vi "NI845X EEPROM Programmer.vi"() -> ()   [LabVIEW 2025]
doc: "This example shows a more generalized way to use the SPI advanced API to write data. It allows the user to change the following parameters: page size, write delay, the endianness of the address bytes, and the number of bytes in an address.\n\nThe parameters will have the following effects:\n\nTarget Page Size (bytes): This places an additional constraint on the amount of bytes written. The smaller value will be used, and that number of bytes written.\nWrite Delay Between Pages (ms): This will force a mandatory delay after writing bytes to a device.\nData Address Width: This will allow the user to specify the EEPROM Data Address as either 1 or 2 bytes.\nData Address Endianness: This control will change the ordering of the bytes in the EEPROM Data Address, note that this only has an effect if there are 2 bytes in the address.\n\nFor connection information see the NI-845x Hardware and Software manual and the manual for your specific SPI device."
uses:
  Subs/ni845x.llb/NI-845x SPI Close Script Reference.vi
  Subs/ni845x.llb/NI-845x SPI Script Us Delay.vi
  <vilib>/LAVA/UI Tools/Dialog/Dialog/Dialog/Dialog__lava_lib_ui_tools.lvclass
  Subs/ni845x.llb/NI-845x SPI Script Ms Delay.vi
  <resource>/objmgr/NI845x.rc
  <userlib>/_OpenG.lib/md5/md5.llb/MD5 Message Digest (Hexadecimal String)__ogtk.vi
  Subs/ni845x.llb/ni845xControl.ctl
  Subs/ni845x.llb/ni845xSpiScriptControl.ctl
panel:
  in  "SPI Script Reference":T1
  in  "Verbose?":bool
  in  "Config INI Save":bool
  in  "Help":bool
  in  "QUIT":bool
  in  "Main Panel":T2(tab)
  in  "Sub-Panel":T3(tab)
  out "Program Data Array":i32(slide) scale=0.0..32.0
  in  "Path to MD5 Fingerprint":path
  in  "Path to BIN file":path
  in  "Upload BIN File":bool
  in  "EEPROM Program Data":string[][](table)
  out "Data Bytes Written":u8[](array[numeric]) format="%x"
  in  "Write Device":bool
  in  "Save to BIN File":bool
  in  "Read Device":bool
  in  "Read ALL Device":bool
  in  "Address":u16 step=1 format="%04x"
  in  "Bytes to Read":u32=2048 min=2 step=2 format="%04x"
  out "Bin Table":string[][](table)
  out "Hex Table":string[][](table)
  in  "Enable Debug?":bool
  in  "Debug Device":bool
  in  "WRITE Data":u8[](array[numeric]) format="%x"
  out "Read Data":u8[](array[numeric]) format="%x"
  out "Status":string
  out "Binary String_Load":string
  out "MD5_File":string
  out "MD5_Calc":string
  out "Binary String_Save":string
  in  "Invert Data Bits [LSB]":bool
  in  "Invert Data Bits [MSB]":bool
  in  "Endianness (WRITE)":bool=TRUE
  in  "Target Page Size (bytes)":u32=2 min=2 step=2 format="%04x"
  in  "Page Write Delay (ms)":u8=7
  in  "Bit Pattern (WRITE ALL)":T4(ring)=enum."All ONES"
  in  "Erase ALL Device":bool
  in  "Write ALL Device":bool
  in  "EWDS":u8=16 format="%08b"
  in  "EWEN":u8=19 format="%08b"
  in  "WRITE":u8=20 format="%08b"
  in  "READ":u8=24 format="%08b"
  in  "ERAL":u8=18 format="%08b"
  in  "WRAL":u8=17 format="%08b"
  in  "Invert Address":bool
  in  "Invert Opcode":bool=TRUE
  in  "CLK Rate (kHz)":u16=2000
  in  "CS/SS Line (0-6)":u32
  in  "IO Level (V)":i32(ring)=33 items=["3.3V"=33, "2.5V"=25, "1.8V"=18, "1.5V"=15, "1.2V"=12]
  in  "CLK Polarity (CPOL)":i32(ring) items=["0 (Idle Low)", "1 (Idle High)"]
  in  "CLK Phase (CPHS)":i32(ring) items=["0 (First Edge)", "1 (Second Edge)"]
  in  "CS Idle Level":enum16{"Low (Assert High)", "High (Assert Low)"}(ring)
  in  "NI845x Device ID":T5="NI-8452"
  in  "Device Mode":enum16{"SPI", "I2C", "DIO"}(ring)
  in  "EEPROM Device Type":T6(ring)=enum."Microchip 93LC86C [8452]"
  in  "Burst Width":enum16{"8 bits", "16 bits", "32 bits"}(ring)=enum."16 bits" caption="Burst Width\n(NI-8452 Only)"
  in  "Address Width":enum16{"8 bits", "16 bits", "32 bits"}(ring)=enum."16 bits"
  # "EEPROM Programmer\n(NI-USB-845x SPI for 8, 16, 32, 64-bit Devices)"
  # "v2.1"
  # "Note: \n1. NI-8451 is 8-bits only!\n2. NI-8452 is 4-64 bits addressable.\n3. NI-845x SPI/I2C programmer device\nsends MSB first!"
  # "<<-- Opcode + 2 bits Address (MSB)"
  # "<<-- Address: 8 bits (LSB)"
  # "<<-- Data: MSB (8 bits)"
  # "<<-- Data: LSB (8 bits)"
  # "WRITE only"
  # "Big Endian"
  # "Little Endian"
  # "WRITE & READ"
  # "Note: SPI programming mode only! I2C & DIO modes not implemented."
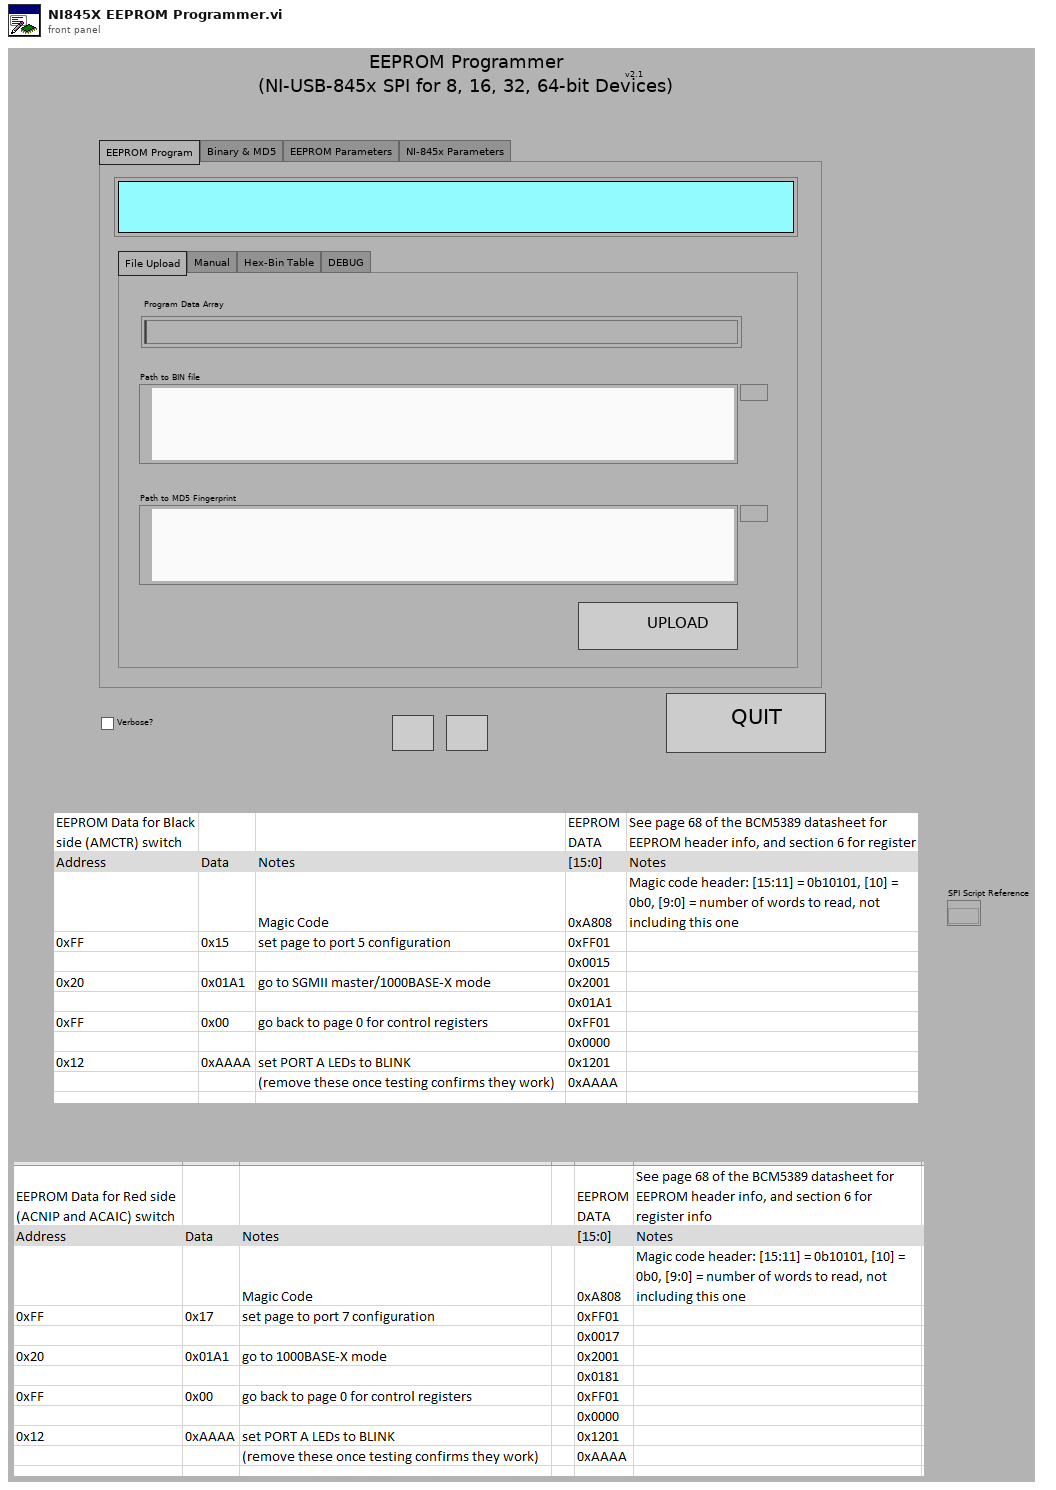
[diagram p1: front panel]
types:
  T1 = typedef "ni845xSpiScriptControl.ctl" = refnum<k20>
  T2 = enum32{"EEPROM Program", "Binary & MD5", "EEPROM Parameters", "NI-845x Parameters"}
  T3 = enum32{"File Upload", "Manual", "Hex-Bin Table", "DEBUG"}
  T4 = enum8{"0xABCD", "0xEEEE", "0xAAAA", "0x5555", "All ONES", "All ZEROES"}
  T5 = typedef "ni845xControl.ctl" = refnum<k21>
  T6 = enum16{"Generic EEPROM", "Microchip LC56BT", "Microchip 93LC86C [8451]", "Microchip 93LC86C [8452]", "ST-M93C86"}
  T7 = enum32{"Invalid", "Standard", "Closed", "Hidden", "Minimized", "Maximized"}
  T8 = enum32{"invalid app kind", "Development System", "Run Time System", "Student Edition", "Embedded LabVIEW", "Evaluation", "Custom"}
  T9 = enum16{"big-endian, network order", "native, host order", "little-endian"}
  T10 = cluster{"INI Path":path, "SPI Script Reference":T1, "NI845x Device ID":T5, "Device Mode":enum16{"SPI", "I2C", "DIO"}, "EEPROM Device Type":enum16{"Generic EEPROM", "Microchip LC56BT", "Microchip 93LC86C [8451]", "Microchip 93LC86C [8452]", "ST-M93C86"}, "Core":cluster{"Current VI Reference":refnum<vi>, "Close Panel on Exit?":bool}, "IO Level (V)":i32, "CS/SS Line (0-6)":u32, "CLK Rate (kHz)":u16, "CLK Polarity (CPOL)":i32, "CLK Phase (CPHS)":i32, " Address Width":enum16{"8 bits", "16 bits", "32 bits"}, "Burst Width":enum16{"8 bits", "16 bits", "32 bits"}, "Address":u16, "Bytes to Read":u32, "Target Page Size (bytes)":u32, "Page Write Delay (ms)":u8, "Array of Write Cluster Information":cluster{"EEPROM Address":u16, "Length":u32, "Data Index":u32}[], "CS Idle Level":enum16{"Low (Assert High)", "High (Assert Low)"}, "script read index":u32, "Bit Pattern (WRITE ALL)":enum8{"0xABCD", "0xEEEE", "0xAAAA", "0x5555", "All ONES", "All ZEROES"}, "READ":u8, "WRITE":u8, "EWEN":u8, "EWDS":u8, "WRAL":u8, "ERAL":u8, "Hex Table":string[][], "Bin Table ":string[][], "EEPROM Program Data ":string[][], "EEPROM Binary File Array":string[][], "Read Data":u8[], "Data Bytes Written":u8[], "WRITE Data":u8[], "Endianness (WRITE)":bool, "Verbose?":bool, "Enable Debug?":bool, "Read ALL":bool, "Invert Data Bits [MSB]":bool, "Invert Data Bits [LSB]":bool, "Invert Opcode":bool, "Invert Address":bool}
  T11 = cluster{"Current VI Reference":refnum<vi>, "Close Panel on Exit?":bool}
  T12 = cluster{"EEPROM Address":u16, "Length":u32, "Data Index":u32}[]
  T13 = typedef "imagedata.ctl" = cluster{"image type":i32, "image depth":i32, "image":u8[], "mask":u8[], "colors":u32[], "Rectangle":cluster{"left":i16, "top":i16, "right":i16, "bottom":i16}}
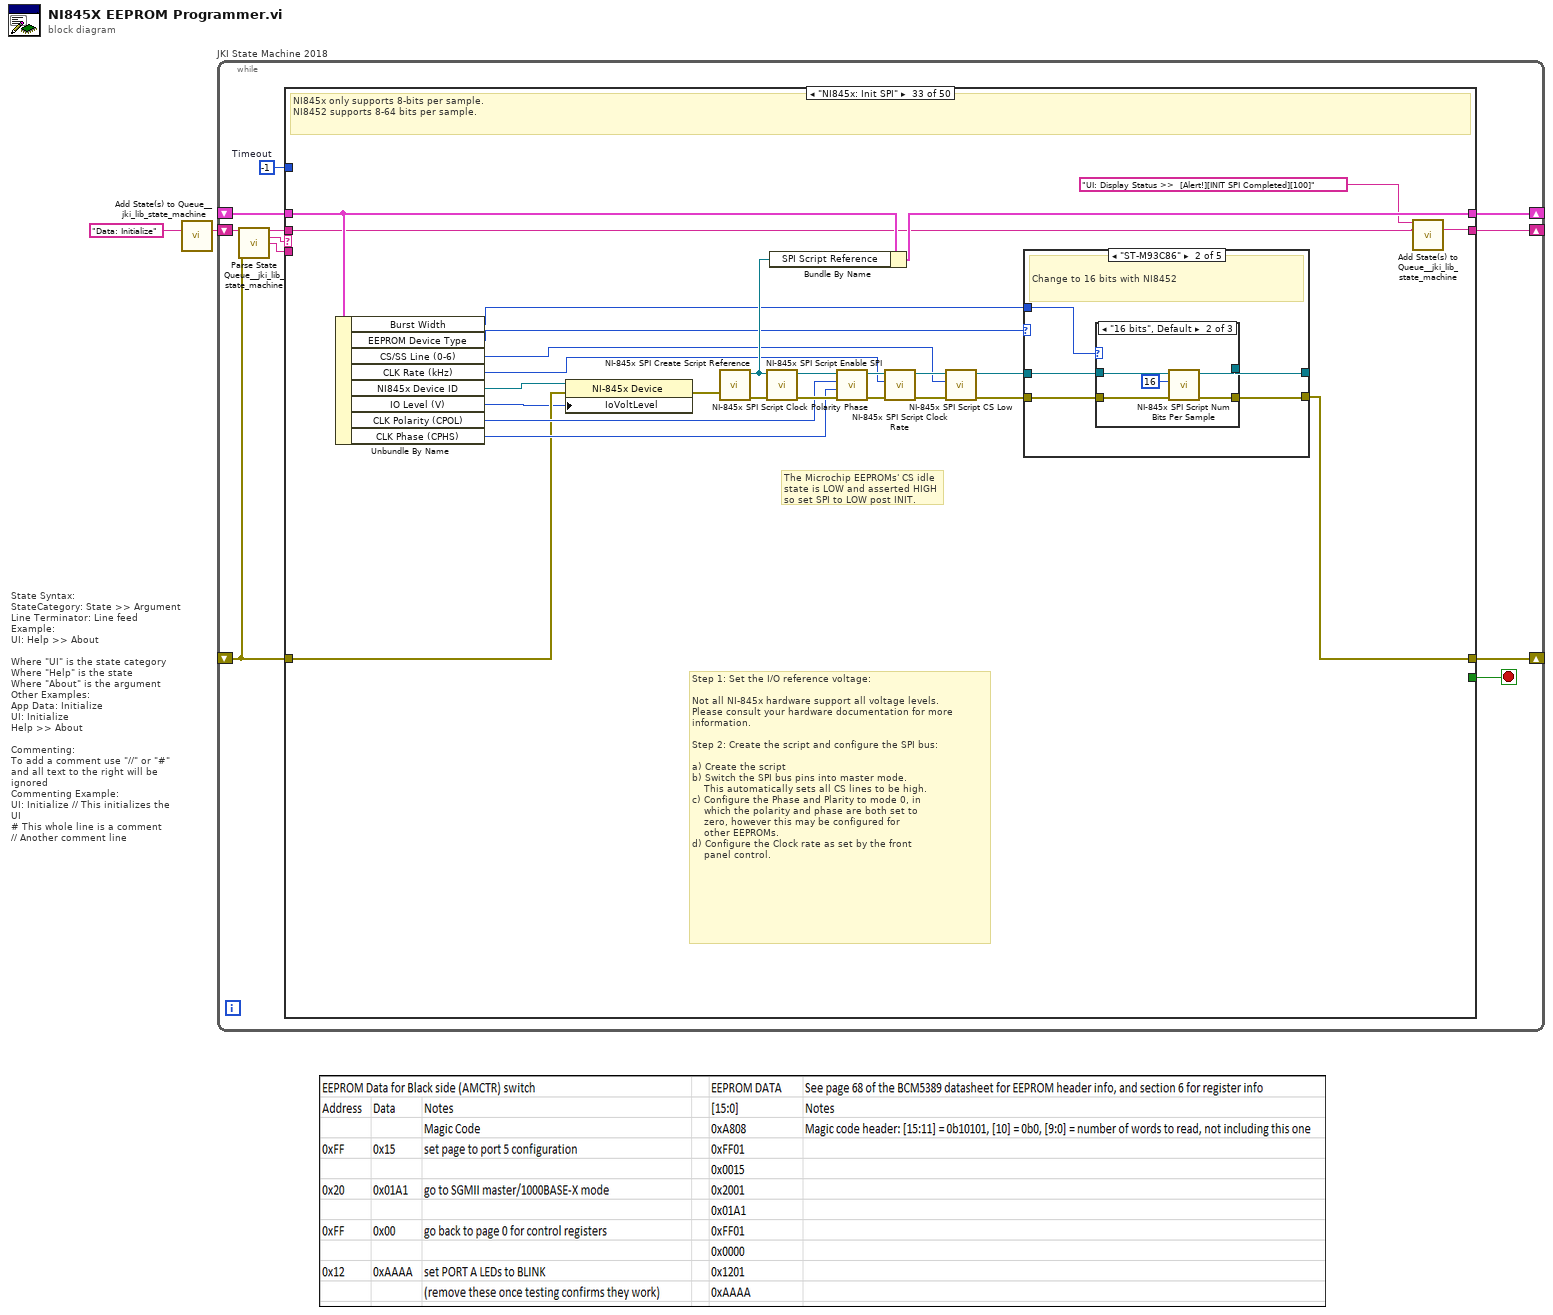
[diagram p0: block diagram]
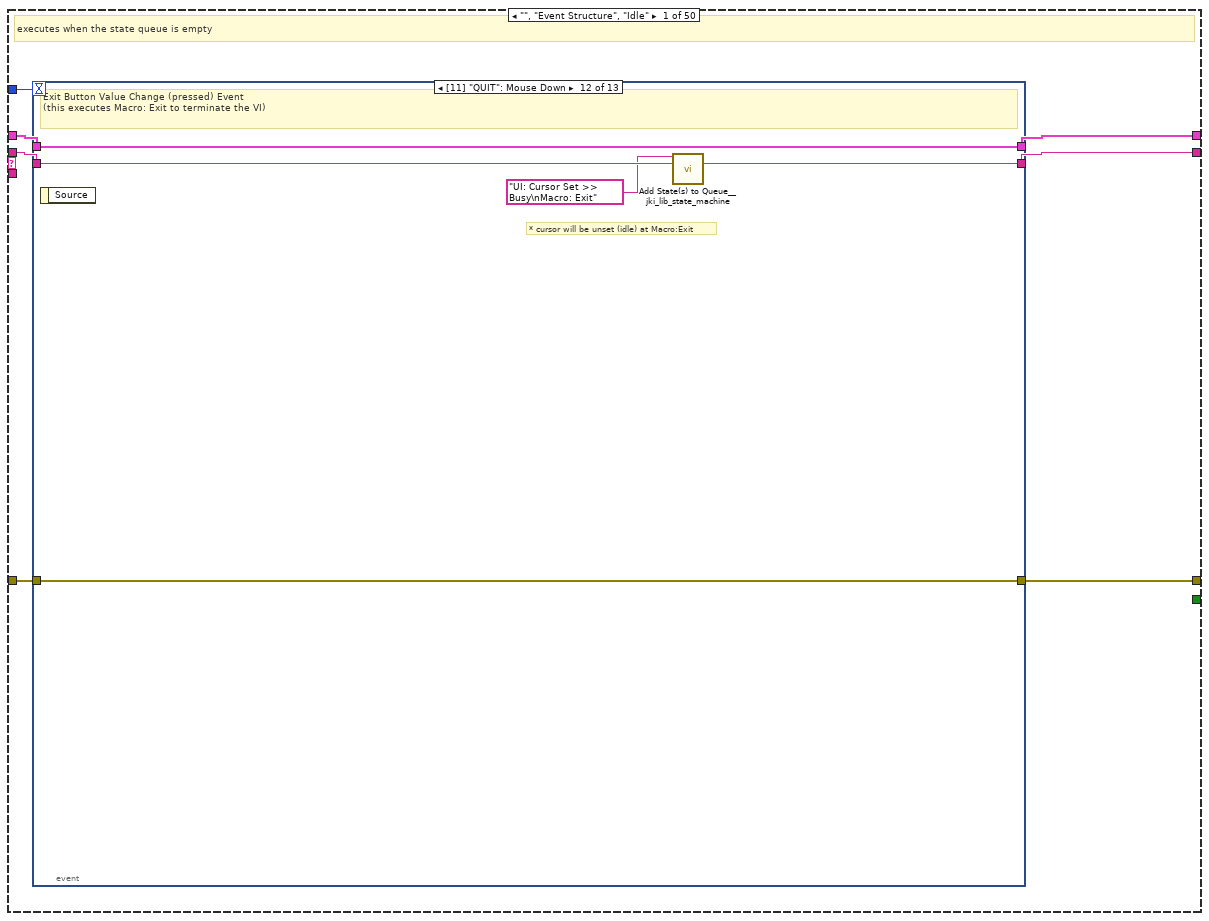
[diagram p2: hidden frame]
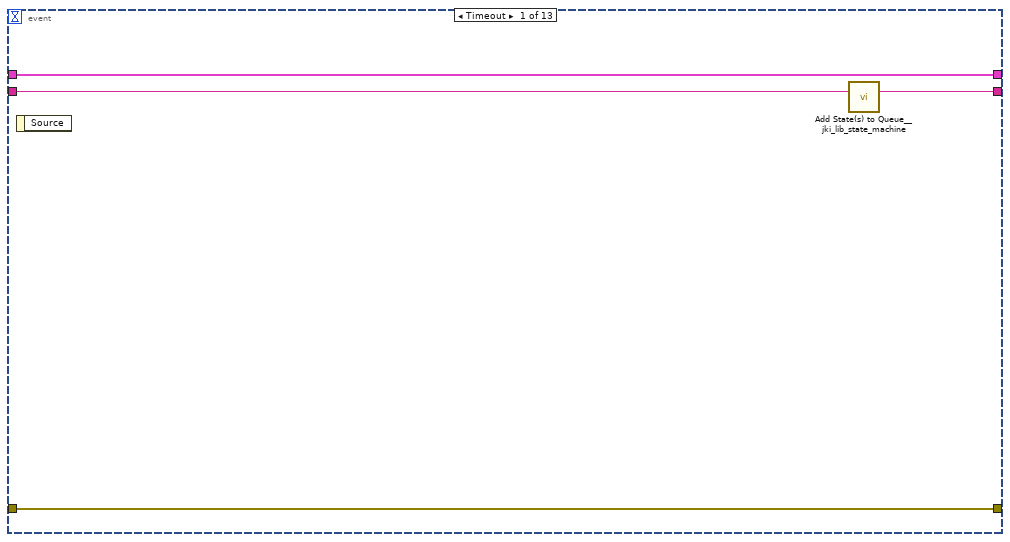
[diagram p3: hidden frame]
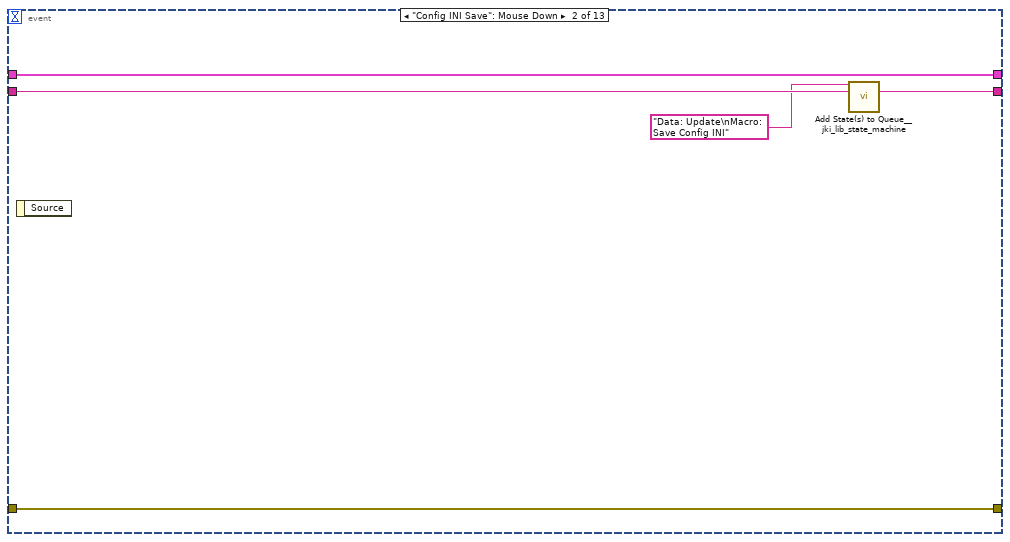
[diagram p4: hidden frame]
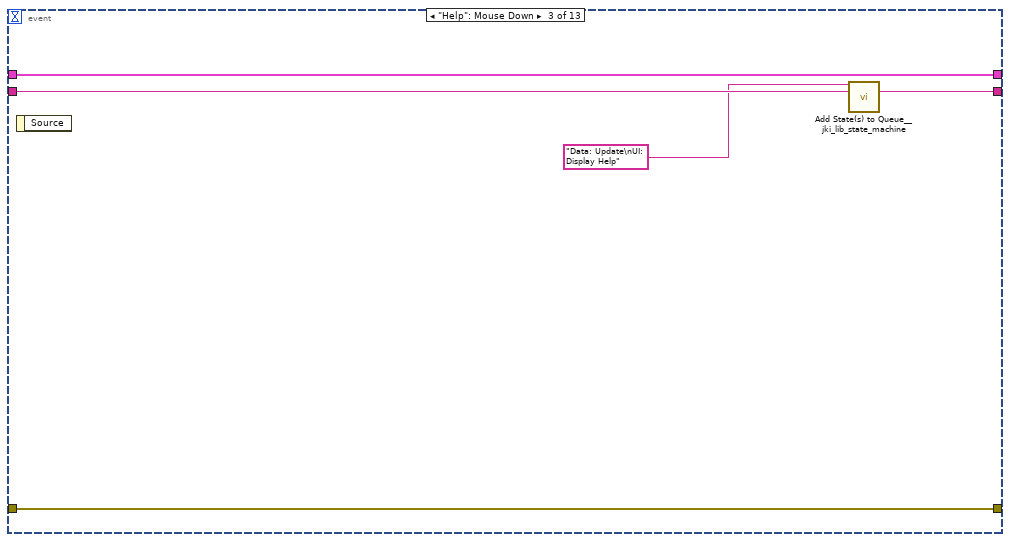
[diagram p5: hidden frame]
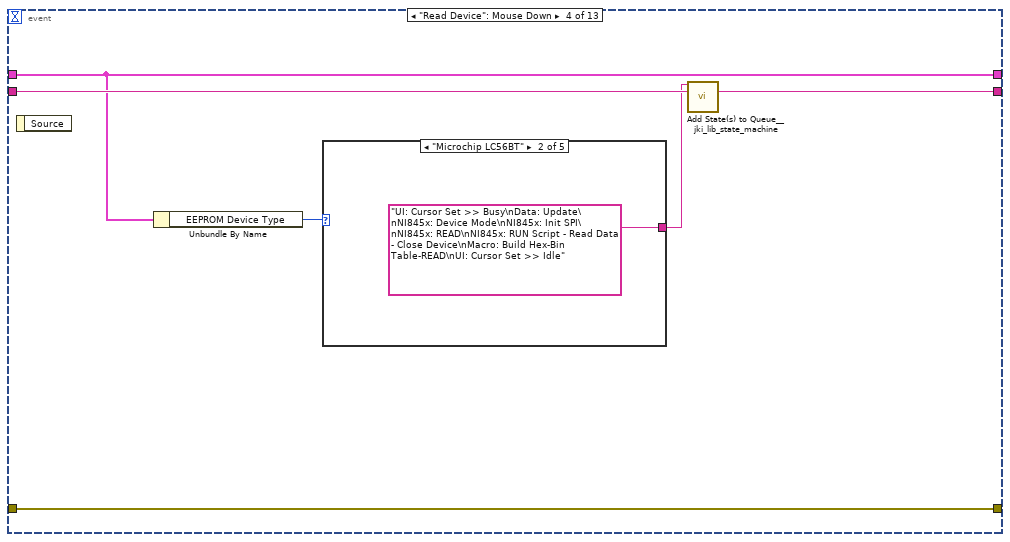
[diagram p6: hidden frame]
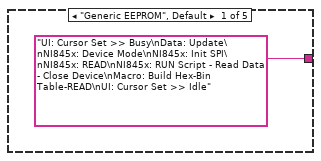
[diagram p7: hidden frame]
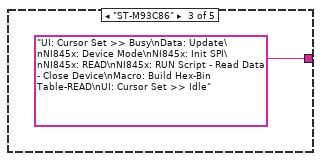
[diagram p8: hidden frame]
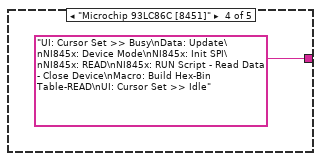
[diagram p9: hidden frame]
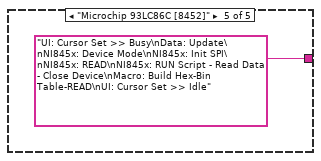
[diagram p10: hidden frame]
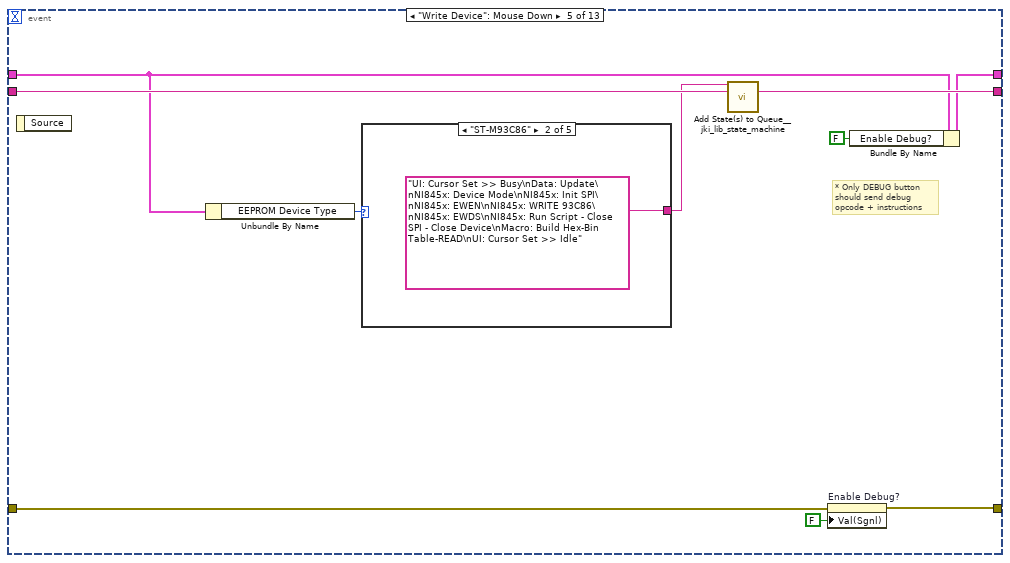
[diagram p11: hidden frame]
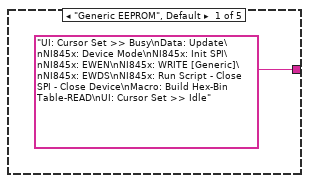
[diagram p12: hidden frame]
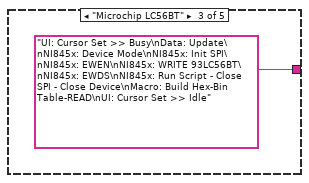
[diagram p13: hidden frame]
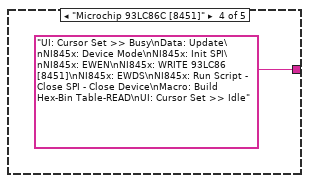
[diagram p14: hidden frame]
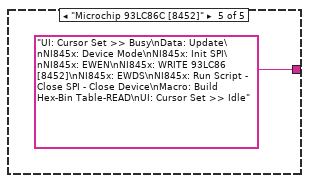
[diagram p15: hidden frame]
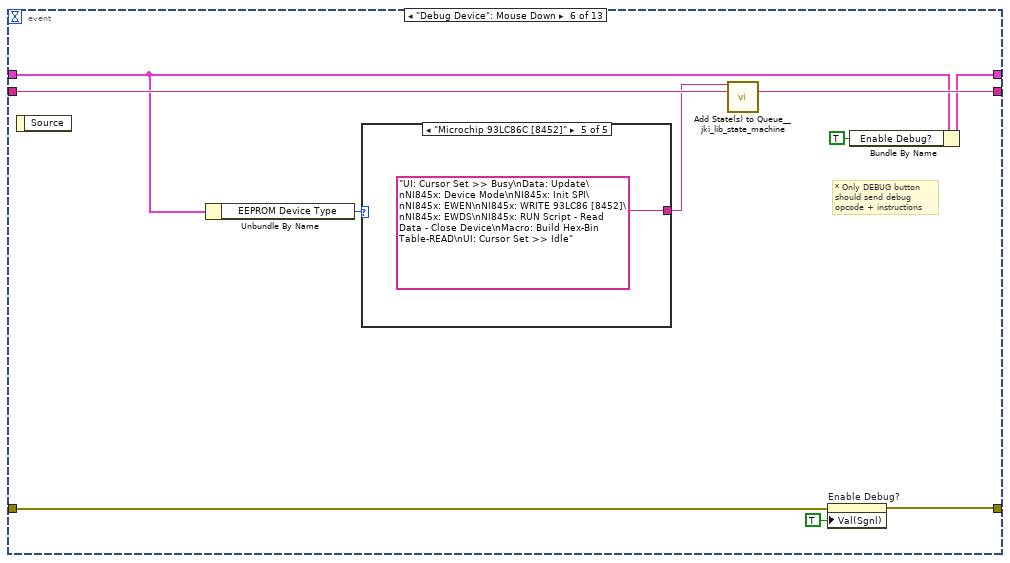
[diagram p16: hidden frame]
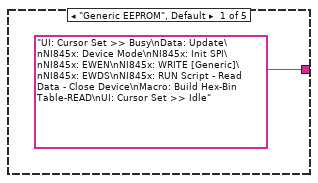
[diagram p17: hidden frame]
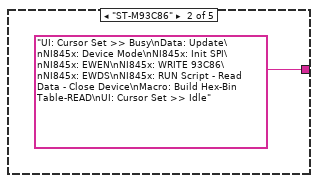
[diagram p18: hidden frame]
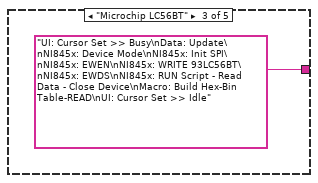
[diagram p19: hidden frame]
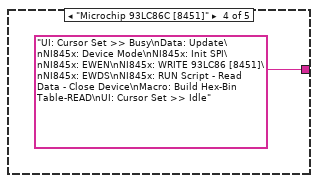
[diagram p20: hidden frame]
diagram:
  # "State Syntax:\nStateCategory: State >> Argument\nLine Terminator: Line feed\nExample:\nUI: Help >> About\n\nWhere \"UI\" is the state category\nWhere \"Help\" is the state\nWhere \"About\" is the argument\nOther Examples:\nApp Data: Initialize\nUI: Initialize\nHelp >> About\n\nCommenting:\nTo add a comment use \"//\" or \"#\" and all text to the right will be ignored\nCommenting Example:\nUI: Initialize // This initializes the UI\n# This whole line is a comment\n// Another comment line"
  n1 = call <vilib>:"Add State(s) to Queue__jki_lib_state_machine.vi"("State(s) in (\"\")"="Data: Initialize") -> ("States Out"=w2:string)  [unwired: 14 in]
  n2 = while "JKI State Machine 2018" {
    shift-right: [w6] -> _
    shift-left: _ -> [w5]
    shift-right: [w9] -> _
    shift-left: _ -> [w3]
    shift-right: [w8] -> _
    shift-left: w2 -> [w10]
    stop <- w7 stop-if-true
    w4 = -1  # Timeout
    n3 = call <vilib>:"Parse State Queue__jki_lib_state_machine.vi"("State Queue"=w10, "Error In (no error)"=w3) -> ("Remaining States"=w12:string, "Current State"=w13:string, "Arguments"=w11:string)  [unwired: 11 in]
    n4 = case shown="\"NI845x: Init SPI\"" w13 {
      selector: w13 -> [_ _ w144 _ _ _ _ _ _ _ _ _ _ _ _ _ _ _ _ _ _ _ _ _ _ _ _ _ _ _ _ _ _ _ _ _ _ _ _ _ _ _ _ _ _ _ _ _ _ _]
      tunnel: w12 -> [w20 w143 w148 w166 w172 w176 w179 w236 w266 w271 w274 w277 w282 w292 w366 w378 w398 w434 w456 w466 w480 w531 w587 w622 w676 w690 w702 w705 w708 w711 w714 w716 w726 w820 w850 w925 w1015 w1103 w1201 w1239 w1348 w1489 w1611 w1653 w1723 w1737 _ w1843 w1860 w1944]
      tunnel: w11 -> [_ _ _ _ _ _ _ _ _ _ _ _ w278 w287 _ w375 w395 _ _ _ _ _ _ _ _ _ _ _ _ _ _ _ _ _ _ _ _ _ _ _ _ _ _ _ _ _ _ _ _ _]
      tunnel: w5 -> [w18 w140 w146 w163 w169 w175 w177 _ w247 w267 w272 w276 w281 w289 w365 w373 w393 w432 w454 w463 w477 w528 w584 w639 w675 w684 w693 w703 w706 w709 w712 w718 w742 w812 w848 w914 w1004 w1093 w1195 w1234 w1343 w1485 w1607 w1646 w1716 w1730 w1766 w1840 w1856 w1941]
      tunnel: [w17 w141 w150 w164 errorcluster {"status"=FALSE, "code"=0, "source"=""} ("error out") w174 w178 w202 w265 w268 w273 w275 w279 w290 w364 w377 w397 w433 w441 w464 w478 w529 w589 w623 w668 w687 w696 w704 w707 w710 w713 w719 w735 w802 w840 w917 w1007 w1095 w1175 w1215 w1319 w1455 w1588 w1648 w1718 w1732 w1768 w1841 w1854 w1934] -> w9
      tunnel: w3 -> [w16 w141 w149 w164 w168 w174 w178 w185 w265 w269 w273 w275 w280 w291 w362 w376 w396 w433 w447 w464 w478 w529 w589 w640 w665 w688 w697 w704 w707 w710 w713 w719 w730 w813 w846 w923 w1013 w1101 w1190 w1230 w1336 w1474 w1587 w1649 w1719 w1733 w1754 w1841 w1855 w1942]
      tunnel: [w19 w142 w147 w166 w171 w176 w179 w235 w266 w271 w274 w277 w282 w292 w366 w378 w398 w434 w455 w465 w479 w530 w586 w621 w676 w689 w701 w705 w708 w711 w714 w720 w725 w819 w849 w924 w1014 w1102 w1200 w1238 w1347 w1488 w1610 w1652 w1722 w1736 w1772 w1842 w1859 w1943] -> w8
      tunnel: [_ _ _ _ _ TRUE _ _ _ _ _ _ _ _ _ _ _ _ _ _ _ _ _ _ _ _ _ _ _ _ _ _ _ _ _ _ _ _ _ _ _ _ _ _ _ _ _ _ _ _] -> w7
      tunnel: [w15 w140 w146 w165 w169 w175 w177 w209 w264 w267 w272 w276 w281 w289 w365 w373 w393 w432 w454 w463 w476 w527 w588 w638 w675 w684 w693 w703 w706 w709 w712 w718 w734 w812 w847 w921 w1011 w1099 w1195 w1232 w1341 w1478 w1597 w1638 w1712 w1726 w1771 w1840 w1850 w1937] -> w6
      tunnel: w4 -> [w14 _ _ _ _ _ _ _ _ _ _ _ _ _ _ _ _ _ _ _ _ _ _ _ _ _ _ _ _ _ _ _ _ _ _ _ _ _ _ _ _ _ _ _ _ _ _ _ _ _]
      frame "", "Event Structure", "Idle" {
        # "executes when the state queue is empty"
        n5 = event shown="[11] \"QUIT\": Mouse Down" {
          selector: _ -> [_ _ _ _ _ _ _ _ _ _ _ _ _]
          dyn-events: _ -> [_ _ _ _ _ _ _ _ _ _ _ _ _]
          timeout: w14 -> [_ _ _ _ _ _ _ _ _ _ _ _ _]
          tunnel: w20 -> [w24 w29 w34 w39 w55 w70 w80 w91 w102 w113 w127 w133 w139]
          tunnel: [w23 w28 w33 w38 w54 w69 w79 w90 w101 w112 w126 w132 w138] -> w19
          tunnel: w18 -> [w21 w26 w31 w36 w52 w67 w77 w88 w99 w110 w124 w130 w136]
          tunnel: [w22 w27 w32 w40 w47 w62 w81 w92 w103 w114 w120 w131 w137] -> w17
          tunnel: w16 -> [w22 w27 w32 w40 w48 w63 w81 w92 w103 w114 w120 w131 w137]
          tunnel: [w21 w26 w31 w36 w50 w65 w77 w88 w99 w110 w122 w130 w136] -> w15
          event Timeout {
            n6 = event-data() -> ()  [unwired: 1 in, 1 out]
            n7 = call <vilib>:"Add State(s) to Queue__jki_lib_state_machine.vi"("State(s) in (\"\")"=w24) -> ("States Out"=w23:string)  [unwired: 14 in]
          }
          event "Config INI Save": Mouse Down {
            n8 = event-data() -> ()  [unwired: 1 in, 1 out]
            n9 = call <vilib>:"Add State(s) to Queue__jki_lib_state_machine.vi"("State(s) in Front (\"\")"="Data: Update\nMacro: Save Config INI" ("State(s) in Front (\"\")"), "State(s) in (\"\")"=w29) -> ("States Out"=w28:string)  [unwired: 13 in]
          }
          event "Help": Mouse Down {
            n10 = event-data() -> ()  [unwired: 1 in, 1 out]
            n11 = call <vilib>:"Add State(s) to Queue__jki_lib_state_machine.vi"("State(s) in Front (\"\")"="Data: Update\nUI: Display Help" ("State(s) in Front (\"\")"), "State(s) in (\"\")"=w34) -> ("States Out"=w33:string)  [unwired: 13 in]
          }
          event "Read Device": Mouse Down {
            n12 = event-data() -> ()  [unwired: 1 in, 1 out]
            n13 = Unbundle By Name(w36) -> ("EEPROM Device Type"=w35:T6)
            n14 = case shown="\"Microchip LC56BT\"" w35 {
              tunnel: ["UI: Cursor Set >> Busy\nData: Update\nNI845x: Device Mode\nNI845x: Init SPI\nNI845x: READ\nNI845x: RUN Script - Read Data - Close Device\nMacro: Build Hex-Bin Table-READ\nUI: Cursor Set >> Idle" ("State(s) in Front (\"\")") "UI: Cursor Set >> Busy\nData: Update\nNI845x: Device Mode\nNI845x: Init SPI\nNI845x: READ\nNI845x: RUN Script - Read Data - Close Device\nMacro: Build Hex-Bin Table-READ\nUI: Cursor Set >> Idle" ("State(s) in Front (\"\")") "UI: Cursor Set >> Busy\nData: Update\nNI845x: Device Mode\nNI845x: Init SPI\nNI845x: READ\nNI845x: RUN Script - Read Data - Close Device\nMacro: Build Hex-Bin Table-READ\nUI: Cursor Set >> Idle" ("State(s) in Front (\"\")") "UI: Cursor Set >> Busy\nData: Update\nNI845x: Device Mode\nNI845x: Init SPI\nNI845x: READ\nNI845x: RUN Script - Read Data - Close Device\nMacro: Build Hex-Bin Table-READ\nUI: Cursor Set >> Idle" ("State(s) in Front (\"\")") "UI: Cursor Set >> Busy\nData: Update\nNI845x: Device Mode\nNI845x: Init SPI\nNI845x: READ\nNI845x: RUN Script - Read Data - Close Device\nMacro: Build Hex-Bin Table-READ\nUI: Cursor Set >> Idle" ("State(s) in Front (\"\")")] -> w37
              frame "Generic EEPROM", Default {
              }
              frame "Microchip LC56BT" {
              }
              frame "ST-M93C86" {
              }
              frame "Microchip 93LC86C [8451]" {
              }
              frame "Microchip 93LC86C [8452]" {
              }
            }
            n15 = call <vilib>:"Add State(s) to Queue__jki_lib_state_machine.vi"("State(s) in Front (\"\")"=w37, "State(s) in (\"\")"=w39) -> ("States Out"=w38:string)  [unwired: 13 in]
          }
          event "Write Device": Mouse Down {
            # "* Only DEBUG button\nshould send debug\nopcode + instructions"
            n16 = event-data() -> ()  [unwired: 1 in, 1 out]
            n17 = Unbundle By Name(w52) -> ("EEPROM Device Type"=w51:T6)
            n18 = case shown="\"ST-M93C86\"" w51 {
              tunnel: ["UI: Cursor Set >> Busy\nData: Update\nNI845x: Device Mode\nNI845x: Init SPI\nNI845x: EWEN\nNI845x: WRITE [Generic]\nNI845x: EWDS\nNI845x: Run Script - Close SPI - Close Device\nMacro: Build Hex-Bin Table-READ\nUI: Cursor Set >> Idle" ("State(s) in Front (\"\")") "UI: Cursor Set >> Busy\nData: Update\nNI845x: Device Mode\nNI845x: Init SPI\nNI845x: EWEN\nNI845x: WRITE 93C86\nNI845x: EWDS\nNI845x: Run Script - Close SPI - Close Device\nMacro: Build Hex-Bin Table-READ\nUI: Cursor Set >> Idle" ("State(s) in Front (\"\")") "UI: Cursor Set >> Busy\nData: Update\nNI845x: Device Mode\nNI845x: Init SPI\nNI845x: EWEN\nNI845x: WRITE 93LC56BT\nNI845x: EWDS\nNI845x: Run Script - Close SPI - Close Device\nMacro: Build Hex-Bin Table-READ\nUI: Cursor Set >> Idle" ("State(s) in Front (\"\")") "UI: Cursor Set >> Busy\nData: Update\nNI845x: Device Mode\nNI845x: Init SPI\nNI845x: EWEN\nNI845x: WRITE 93LC86 [8451]\nNI845x: EWDS\nNI845x: Run Script - Close SPI - Close Device\nMacro: Build Hex-Bin Table-READ\nUI: Cursor Set >> Idle" ("State(s) in Front (\"\")") "UI: Cursor Set >> Busy\nData: Update\nNI845x: Device Mode\nNI845x: Init SPI\nNI845x: EWEN\nNI845x: WRITE 93LC86 [8452]\nNI845x: EWDS\nNI845x: Run Script - Close SPI - Close Device\nMacro: Build Hex-Bin Table-READ\nUI: Cursor Set >> Idle" ("State(s) in Front (\"\")")] -> w53
              frame "Generic EEPROM", Default {
              }
              frame "ST-M93C86" {
              }
              frame "Microchip LC56BT" {
              }
              frame "Microchip 93LC86C [8451]" {
              }
              frame "Microchip 93LC86C [8452]" {
              }
            }
            n19 = call <vilib>:"Add State(s) to Queue__jki_lib_state_machine.vi"("State(s) in Front (\"\")"=w53, "State(s) in (\"\")"=w55) -> ("States Out"=w54:string)  [unwired: 13 in]
            n20 = property on="Enable Debug?" class="Bool (strict)"(error in=w48, "Val(Sgnl)"=FALSE ("Value (Signaling)")) -> (error out=w47:errorcluster)  [unwired: 1 in, 1 out]
            n21 = Bundle By Name(cluster=w52, "Enable Debug?"=FALSE) -> (w50:T10)
          }
          event "Debug Device": Mouse Down {
            # "* Only DEBUG button\nshould send debug\nopcode + instructions"
            n22 = event-data() -> ()  [unwired: 1 in, 1 out]
            n23 = Unbundle By Name(w67) -> ("EEPROM Device Type"=w66:T6)
            n24 = case shown="\"Microchip 93LC86C [8452]\"" w66 {
              tunnel: ["UI: Cursor Set >> Busy\nData: Update\nNI845x: Device Mode\nNI845x: Init SPI\nNI845x: EWEN\nNI845x: WRITE [Generic]\nNI845x: EWDS\nNI845x: RUN Script - Read Data - Close Device\nMacro: Build Hex-Bin Table-READ\nUI: Cursor Set >> Idle" ("State(s) in Front (\"\")") "UI: Cursor Set >> Busy\nData: Update\nNI845x: Device Mode\nNI845x: Init SPI\nNI845x: EWEN\nNI845x: WRITE 93C86\nNI845x: EWDS\nNI845x: RUN Script - Read Data - Close Device\nMacro: Build Hex-Bin Table-READ\nUI: Cursor Set >> Idle" ("State(s) in Front (\"\")") "UI: Cursor Set >> Busy\nData: Update\nNI845x: Device Mode\nNI845x: Init SPI\nNI845x: EWEN\nNI845x: WRITE 93LC56BT\nNI845x: EWDS\nNI845x: RUN Script - Read Data - Close Device\nMacro: Build Hex-Bin Table-READ\nUI: Cursor Set >> Idle" ("State(s) in Front (\"\")") "UI: Cursor Set >> Busy\nData: Update\nNI845x: Device Mode\nNI845x: Init SPI\nNI845x: EWEN\nNI845x: WRITE 93LC86 [8451]\nNI845x: EWDS\nNI845x: RUN Script - Read Data - Close Device\nMacro: Build Hex-Bin Table-READ\nUI: Cursor Set >> Idle" ("State(s) in Front (\"\")") "UI: Cursor Set >> Busy\nData: Update\nNI845x: Device Mode\nNI845x: Init SPI\nNI845x: EWEN\nNI845x: WRITE 93LC86 [8452]\nNI845x: EWDS\nNI845x: RUN Script - Read Data - Close Device\nMacro: Build Hex-Bin Table-READ\nUI: Cursor Set >> Idle" ("State(s) in Front (\"\")")] -> w68
              frame "Generic EEPROM", Default {
              }
              frame "ST-M93C86" {
              }
              frame "Microchip LC56BT" {
              }
              frame "Microchip 93LC86C [8451]" {
              }
              frame "Microchip 93LC86C [8452]" {
              }
            }
            n25 = call <vilib>:"Add State(s) to Queue__jki_lib_state_machine.vi"("State(s) in Front (\"\")"=w68, "State(s) in (\"\")"=w70) -> ("States Out"=w69:string)  [unwired: 13 in]
            n26 = property on="Enable Debug?" class="Bool (strict)"(error in=w63, "Val(Sgnl)"=TRUE ("Value (Signaling)")) -> (error out=w62:errorcluster)  [unwired: 1 in, 1 out]
            n27 = Bundle By Name(cluster=w67, "Enable Debug?"=TRUE) -> (w65:T10)
          }
          event "Read ALL Device": Mouse Down {
            n28 = event-data() -> ()  [unwired: 1 in, 1 out]
            n29 = Unbundle By Name(w77) -> ("EEPROM Device Type"=w76:T6)
            n30 = case shown="\"Generic EEPROM\", Default" w76 {
              tunnel: ["UI: Cursor Set >> Busy\nData: Update\nNI845x: Device Mode\nNI845x: Init SPI\nNI845x: READ ALL\nNI845x: RUN Script - Read Data - Close Device\nMacro: Build Hex-Bin Table-READ-ALL\nUI: Cursor Set >> Idle" ("State(s) in Front (\"\")") "UI: Cursor Set >> Busy\nData: Update\nNI845x: Device Mode\nNI845x: Init SPI\nNI845x: READ ALL\nNI845x: RUN Script - Read Data - Close Device\nMacro: Build Hex-Bin Table-READ-ALL\nUI: Cursor Set >> Idle" ("State(s) in Front (\"\")") "UI: Cursor Set >> Busy\nData: Update\nNI845x: Device Mode\nNI845x: Init SPI\nNI845x: READ ALL\nNI845x: RUN Script - Read Data - Close Device\nMacro: Build Hex-Bin Table-READ-ALL\nUI: Cursor Set >> Idle" ("State(s) in Front (\"\")") "UI: Cursor Set >> Busy\nData: Update\nNI845x: Device Mode\nNI845x: Init SPI\nNI845x: READ ALL\nNI845x: RUN Script - Read Data - Close Device\nMacro: Build Hex-Bin Table-READ-ALL\nUI: Cursor Set >> Idle" ("State(s) in Front (\"\")") "UI: Cursor Set >> Busy\nData: Update\nNI845x: Device Mode\nNI845x: Init SPI\nNI845x: READ ALL\nNI845x: RUN Script - Read Data - Close Device\nMacro: Build Hex-Bin Table-READ-ALL\nUI: Cursor Set >> Idle" ("State(s) in Front (\"\")")] -> w78
              frame "Microchip LC56BT" {
              }
              frame "ST-M93C86" {
              }
              frame "Microchip 93LC86C [8452]" {
              }
              frame "Microchip 93LC86C [8451]" {
              }
              frame "Generic EEPROM", Default {
              }
            }
            n31 = call <vilib>:"Add State(s) to Queue__jki_lib_state_machine.vi"("State(s) in Front (\"\")"=w78, "State(s) in (\"\")"=w80) -> ("States Out"=w79:string)  [unwired: 13 in]
          }
          event "Write ALL Device": Mouse Down {
            n32 = event-data() -> ()  [unwired: 1 in, 1 out]
            n33 = Unbundle By Name(w88) -> ("EEPROM Device Type"=w87:T6)
            n34 = case shown="\"Microchip 93LC86C [8452]\"" w87 {
              tunnel: ["UI: Cursor Set >> Busy\nData: Update\nNI845x: Device Mode\nNI845x: Init SPI\nNI845x: EWEN\nNI845x: WRITE ALL\nNI845x: EWDS\nNI845x: Run Script - Close SPI - Close Device\nUI: Cursor Set >> Idle" ("State(s) in Front (\"\")") "UI: Cursor Set >> Busy\nData: Update\nNI845x: Device Mode\nNI845x: Init SPI\nNI845x: EWEN\nNI845x: WRITE ALL\nNI845x: EWDS\nNI845x: Run Script - Close SPI - Close Device\nUI: Cursor Set >> Idle" ("State(s) in Front (\"\")") "UI: Cursor Set >> Busy\nData: Update\nNI845x: Device Mode\nNI845x: Init SPI\nNI845x: EWEN\nNI845x: WRITE ALL\nNI845x: EWDS\nNI845x: Run Script - Close SPI - Close Device\nUI: Cursor Set >> Idle" ("State(s) in Front (\"\")") "UI: Cursor Set >> Busy\nData: Update\nNI845x: Device Mode\nNI845x: Init SPI\nNI845x: EWEN\nNI845x: WRITE ALL\nNI845x: EWDS\nNI845x: Run Script - Close SPI - Close Device\nUI: Cursor Set >> Idle" ("State(s) in Front (\"\")") "UI: Cursor Set >> Busy\nData: Update\nNI845x: Device Mode\nNI845x: Init SPI\nNI845x: EWEN\nNI845x: WRITE ALL\nNI845x: EWDS\nNI845x: Run Script - Close SPI - Close Device\nUI: Cursor Set >> Idle" ("State(s) in Front (\"\")")] -> w89
              frame "Generic EEPROM", Default {
              }
              frame "ST-M93C86" {
              }
              frame "Microchip LC56BT" {
              }
              frame "Microchip 93LC86C [8451]" {
              }
              frame "Microchip 93LC86C [8452]" {
              }
            }
            n35 = call <vilib>:"Add State(s) to Queue__jki_lib_state_machine.vi"("State(s) in Front (\"\")"=w89, "State(s) in (\"\")"=w91) -> ("States Out"=w90:string)  [unwired: 13 in]
          }
          event "Erase ALL Device": Mouse Down {
            n36 = event-data() -> ()  [unwired: 1 in, 1 out]
            n37 = Unbundle By Name(w99) -> ("EEPROM Device Type"=w98:T6)
            n38 = case shown="\"Microchip 93LC86C [8452]\"" w98 {
              tunnel: ["UI: Cursor Set >> Busy\nData: Update\nNI845x: Device Mode\nNI845x: Init SPI\nNI845x: EWEN\nNI845x: ERASE ALL\nNI845x: EWDS\nNI845x: Run Script - Close SPI - Close Device\nUI: Cursor Set >> Idle" ("State(s) in Front (\"\")") "UI: Cursor Set >> Busy\nData: Update\nNI845x: Device Mode\nNI845x: Init SPI\nNI845x: EWEN\nNI845x: ERASE ALL\nNI845x: EWDS\nNI845x: Run Script - Close SPI - Close Device\nUI: Cursor Set >> Idle" ("State(s) in Front (\"\")") "UI: Cursor Set >> Busy\nData: Update\nNI845x: Device Mode\nNI845x: Init SPI\nNI845x: EWEN\nNI845x: ERASE ALL\nNI845x: EWDS\nNI845x: Run Script - Close SPI - Close Device\nUI: Cursor Set >> Idle" ("State(s) in Front (\"\")") "UI: Cursor Set >> Busy\nData: Update\nNI845x: Device Mode\nNI845x: Init SPI\nNI845x: EWEN\nNI845x: ERASE ALL\nNI845x: EWDS\nNI845x: Run Script - Close SPI - Close Device\nUI: Cursor Set >> Idle" ("State(s) in Front (\"\")") "UI: Cursor Set >> Busy\nData: Update\nNI845x: Device Mode\nNI845x: Init SPI\nNI845x: EWEN\nNI845x: ERASE ALL\nNI845x: EWDS\nNI845x: Run Script - Close SPI - Close Device\nUI: Cursor Set >> Idle" ("State(s) in Front (\"\")")] -> w100
              frame "Generic EEPROM", Default {
              }
              frame "ST-M93C86" {
              }
              frame "Microchip LC56BT" {
              }
              frame "Microchip 93LC86C [8451]" {
              }
              frame "Microchip 93LC86C [8452]" {
              }
            }
            n39 = call <vilib>:"Add State(s) to Queue__jki_lib_state_machine.vi"("State(s) in Front (\"\")"=w100, "State(s) in (\"\")"=w102) -> ("States Out"=w101:string)  [unwired: 13 in]
          }
          event "Save to BIN File": Mouse Down {
            n40 = event-data() -> ()  [unwired: 1 in, 1 out]
            n41 = Unbundle By Name(w110) -> ("EEPROM Device Type"=w109:T6)
            n42 = case shown="\"Microchip 93LC86C [8451]\"" w109 {
              tunnel: ["UI: Cursor Set >> Busy\nData: Update\nNI845x: Device Mode\nNI845x: Init SPI\nNI845x: READ ALL\nNI845x: RUN Script - Read Data - Close Device\nMacro: Build Hex-Bin Table-READ-ALL\nMacro: Save Binary File\nUI: Cursor Set >> Idle" ("State(s) in Front (\"\")") "UI: Cursor Set >> Busy\nData: Update\nNI845x: Device Mode\nNI845x: Init SPI\nNI845x: READ ALL\nNI845x: RUN Script - Read Data - Close Device\nMacro: Build Hex-Bin Table-READ-ALL\nMacro: Save Binary File\nUI: Cursor Set >> Idle" ("State(s) in Front (\"\")") "UI: Cursor Set >> Busy\nData: Update\nNI845x: Device Mode\nNI845x: Init SPI\nNI845x: READ ALL\nNI845x: RUN Script - Read Data - Close Device\nMacro: Build Hex-Bin Table-READ-ALL\nMacro: Save Binary File\nUI: Cursor Set >> Idle" ("State(s) in Front (\"\")") "UI: Cursor Set >> Busy\nData: Update\nNI845x: Device Mode\nNI845x: Init SPI\nNI845x: READ ALL\nNI845x: RUN Script - Read Data - Close Device\nMacro: Build Hex-Bin Table-READ-ALL\nMacro: Save Binary File\nUI: Cursor Set >> Idle" ("State(s) in Front (\"\")") "UI: Cursor Set >> Busy\nData: Update\nNI845x: Device Mode\nNI845x: Init SPI\nNI845x: READ ALL\nNI845x: RUN Script - Read Data - Close Device\nMacro: Build Hex-Bin Table-READ-ALL\nMacro: Save Binary File\nUI: Cursor Set >> Idle" ("State(s) in Front (\"\")")] -> w111
              frame "Microchip LC56BT" {
              }
              frame "ST-M93C86" {
              }
              frame "Microchip 93LC86C [8452]" {
              }
              frame "Microchip 93LC86C [8451]" {
              }
              frame "Generic EEPROM", Default {
              }
            }
            n43 = call <vilib>:"Add State(s) to Queue__jki_lib_state_machine.vi"("State(s) in Front (\"\")"=w111, "State(s) in (\"\")"=w113) -> ("States Out"=w112:string)  [unwired: 13 in]
          }
          event "Upload BIN File": Mouse Down {
            # "* Enable Debug Mode\nfor Binary File Upload\nto EEPROM"
            n44 = event-data() -> ()  [unwired: 1 in, 1 out]
            n45 = Unbundle By Name(w124) -> ("EEPROM Device Type"=w123:T6)
            n46 = case shown="\"Microchip 93LC86C [8452]\", Default" w123 {
              tunnel: ["UI: Display Status >>  [Alert!][Uploading BInary File][100]\nUI: Cursor Set >> Busy\nData: Update\nMacro: Load Binary File\nMacro: Build Program Data\nNI845x: Device Mode\nNI845x: Init SPI\nNI845x: EWEN\nNI845x: Upload BInary File" ("State(s) in Front (\"\")")] -> w125
              frame "Microchip 93LC86C [8452]", Default {
              }
            }
            n47 = call <vilib>:"Add State(s) to Queue__jki_lib_state_machine.vi"("State(s) in Front (\"\")"=w125, "State(s) in (\"\")"=w127) -> ("States Out"=w126:string)  [unwired: 13 in]
            n48 = Bundle By Name(cluster=w124, "Enable Debug?"=TRUE) -> (w122:T10)
          }
          event "QUIT": Mouse Down {
            # "* cursor will be unset (idle) at Macro:Exit"
            # "Exit Button Value Change (pressed) Event\n(this executes Macro: Exit to terminate the VI)"
            n49 = event-data() -> ()  [unwired: 1 in, 1 out]
            n50 = call <vilib>:"Add State(s) to Queue__jki_lib_state_machine.vi"("State(s) in Front (\"\")"="UI: Cursor Set >> Busy\nMacro: Exit", "State(s) in (\"\")"=w133) -> ("States Out"=w132:string)  [unwired: 13 in]
          }
          event Panel Close? {
            # "Discard the event because we'll close the front panel ourselves in Macro: Exit"
            # "Close Panel button (pressed) Event\n(this executes Macro: Exit to terminate the VI)"
            n51 = event-data() -> ()  [unwired: 1 in, 1 out]
            n52 = call <vilib>:"Add State(s) to Queue__jki_lib_state_machine.vi"("State(s) in Front (\"\")"="UI: Cursor Set >> Idle\nMacro: Exit", "State(s) in (\"\")"=w139) -> ("States Out"=w138:string)  [unwired: 13 in]
            n53 = event-data("Discard?"=TRUE) -> ()  [unwired: 1 in, 1 out]
          }
        }
      }
      frame "---------- Core ----------" {
        # "Do not put any code in this frame.\n(it is a separator no-op)"
        n54 = call <vilib>:"Add State(s) to Queue__jki_lib_state_machine.vi"("State(s) in (\"\")"=w143) -> ("States Out"=w142:string)  [unwired: 14 in]
      }
      frame Default {
        w153 = 42 items=["No error", "Argument error", "Memory is full", "Out of zone", "End of file", "File already open", "Generic file I/O error", "File not found", "File permission error", "Disk is full", "Duplicate path", "Too many files open", "System feature not enabled", "Resource file not found", "Cannot add resource", "Resource not found", "Image not found", "Image memory error", "Pen does not exist", "Config type invalid", "Config token not found", "Config parse error", "Config memory error", "Bad external code format", "Bad external code offset", "External code not present", "Null window", "Destroy window error", "Null menu", "Print aborted", "Bad print record", "Print driver error", "Windows error during printing", "Memory error during printing", "Print dialog error", "Generic print error", "Invalid device refnum", "Device not found", "Device parameter error", "Device unit error", "Cannot open device", "Device call aborted", "Generic error", "Cancelled by user", "Object ID too low", "Object ID too high", "Object not in heap", "Unknown heap", "Unknown object (invalid DefProc)", "Unknown object (DefProc not in table)", "Message out of range", "Invalid (null) method", "Unknown message", "Manager call not supported", "Bad address", "Network operation in progress", "Network operation timed out", "Connection is busy", "Network attribute not supported", "Network error", "Address in use", "System out of memory", "Connection aborted", "Connection refused", "Not connected", "Already connected", "Connection closed", "Initialization error (interapplication manager)", "Bad occurrence", "Wait on unbound occurrence handler", "Occurrence queue overflow", "Datalog type conflict", "Unused", "Unrecognized type (interapplication manager)", "Memory corrupt", "Failed to make temporary DLL", "Old CIN version", "Drag socket not found", "Failed to load drop-object", "Failed to register OLE object", "Failed to release OLE object", "Format specifier type mismatch", "Unknown format specifier", "Too few format specifiers", "Too many format specifiers", "Scan failed", "Newer CIN version", "Error converting to variant", "Runtime menu error", "Password tampered", "Variant attribute not found", "Incompatible variant data type", "Event data is not available", "Event Store is not present", "Occurrence is not found", "Event Queue is not created", "Event info is not available", "Refnum passed is NULL", "Error retrieving Class GUID", "Error retrieving CoClass GUID", "Error retrieving TypeLib GUID.", "Bad built application magic bytes.", "Specific driver is different from the specific driver associated with the Logical Name.", "There is no session opened to the class driver.", "Max Error", "MAX - Error with config objects", "MAX - Error loading configuration", "MAX - Group not supported"]
        # "Current State"
        # "Handle mistyped state name (developer tool)"
        # "Do not delete, rename, or modify this frame.\n(this is used to capture unhandled states and typos)"
        n55 = Format Into String(format string="Software Exception: Unhandled State \"%s\"." ("message"), error in=w149, w144) -> (resulting string=w152:string, error out=w151:errorcluster)  [unwired: 1 in]
        n56 = call <vilib>:"Error Cluster From Error Code.vi"("show call chain? (False)"=TRUE, "error in (no error)"=w151, "error message (\"\")"=w152, "error code (0)"=w153) -> ("error out"=w150:errorcluster)  [unwired: 5 in]
        n57 = call <vilib>:"Add State(s) to Queue__jki_lib_state_machine.vi"("State(s) in (\"\")"=w148) -> ("States Out"=w147:string)  [unwired: 14 in]
      }
      frame "Initialize Core Data" {
        # "originally closed?"
        # "exe?"
        # "If panel starts closed or is an EXE, then close it when we exit"
        # "Do not delete, rename, or modify this frame.\n(this is used to determine panel behavior on exit)"
        n58 = property class="VI"() -> ("FP.State"=w158:T7)  [unwired: 2 in, 2 out]
        n59 = property class="App"() -> ("App.Kind"=w161:T8)  [unwired: 2 in, 2 out]
        n60 = control-ref of="Current VI Reference"() -> (w162:refnum<vi>)
        n61 = Equal?(x=w158, y=T7."Closed" ("Front Panel Window:State")) -> (x = y?=w156:bool)
        n62 = Equal?(x=w161, y=T8."Run Time System" ("Application:Kind")) -> (x = y?=w159:bool)
        n63 = Or(x=w156, y=w159) -> (x .or. y?=w155:bool)
        n64 = Bundle By Name(cluster=w163, "Core.Current VI Reference"=w162, "Core.Close Panel on Exit?"=w155) -> (w165:T10)
      }
      frame "Error Handler" {
        # "Unhandled Error -- Display it"
        # "Clear error"
        # "Handle any errors here.\nYou can also output any states to clean-up after errors occur"
        n65 = call <vilib>:"General Error Handler.vi"("error in (no error)"=w168) -> ()  [unwired: 10 in, 5 out]
        n66 = call <vilib>:"Add State(s) to Queue__jki_lib_state_machine.vi"("State(s) in Front (\"\")"="/* Post Error States", "State(s) in (\"\")"=w172) -> ("States Out"=w171:string)  [unwired: 13 in]
      }
      frame "Exit" {
        # "Do not put any code in this frame.\n(No errors that occur here will be handled.)"
      }
      frame "---------- Data ----------" {
        # "Do not put any code in this frame.\n(It is a separator no-op. You can make a copy of this frame to create a new Data frame)"
      }
      frame "Data: Initialize" {
        w180 = string[][] []  # EEPROM Program Data
        w181 = string[][] []  # EEPROM Binary File Array
        w183 = ""
        w192 = FALSE  # Read ALL
        w195 = string[][] []  # Bin Table
        w196 = string[][] []  # Hex Table
        w197 = string[][] []  # Hex Table
        w199 = u8[] []  # Data Bytes Written
        w200 = u8[] []  # Read Data
        w210 = path ""  # INI Path
        w219 = u8[] [] ("Read Data")
        w224 = u32 0  # script read index
        w205 = T11 {"Current VI Reference"=refnum, "Close Panel on Exit?"=FALSE}  # Core
        # "do not delete - used by framework"
        # "Initialize variables & master cluster here\n(data names are defined by what you wire into the bundle function)"
        n67 = property on="QUIT" class="Bool (strict)"(error in=w185, "Value"=FALSE ("QUIT")) -> (error out=w186:errorcluster)  [unwired: 1 in, 1 out]
        n68 = call "CreateWriteCluster.vi"("Page Size in Bytes"="Target Page Size (bytes)", "EEPROM Starting Address"="Address", "Number of Bytes to Write"="Bytes to Read") -> ("Array of Write Cluster Information"=w213:T12)  [unwired: 1 in]
        n69 = control-ref of="This VI"() -> (w203:refnum<vi>)
        n70 = call "Set Config INI PATH.vi"("error in (no error)"=w186, "reference"=w203) -> ("error out"=w202:errorcluster, "appended path"=w201:path)  [unwired: 2 in]
        n71 = Bundle("INI Path"=w210, "SPI Script Reference"="SPI Script Reference", "NI845x Device ID"="NI845x Device ID", "Device Mode"="Device Mode", "EEPROM Device Type"="EEPROM Device Type", "Core"=w205, "IO Level (V)"="IO Level (V)", "CS/SS Line (0-6)"="CS/SS Line (0-6)", "CLK Rate (kHz)"="CLK Rate (kHz)", "CLK Polarity (CPOL)"="CLK Polarity (CPOL)", "CLK Phase (CPHS)"="CLK Phase (CPHS)", "Address Width"="Address Width", "Burst Width"="Burst Width", "Address"="Address", "Bytes to Read"="Bytes to Read", "Target Page Size (bytes)"="Target Page Size (bytes)", "Page Write Delay (ms)"="Page Write Delay (ms)", "Array of Write Cluster Information"=w213, "CS Idle Level"="CS Idle Level", "script read index"=w224, "Bit Pattern (WRITE ALL)"="Bit Pattern (WRITE ALL)", "READ"="READ", "WRITE"="WRITE", "EWEN"="EWEN", "EWDS"="EWDS", "WRAL"="WRAL", "ERAL"="ERAL", "Hex Table"=w196, "Bin Table"=w195, "EEPROM Program Data"=w180, "EEPROM Binary File Array"=w181, "Read Data"=w200, "Data Bytes Written"=w199, "WRITE Data"="WRITE Data", "Endianness (WRITE)"="Endianness (WRITE)", "Verbose?"="Verbose?", "Enable Debug?"="Enable Debug?", "Read ALL"=w192, "Invert Data Bits [MSB]"="Invert Data Bits [MSB]", "Invert Data Bits [LSB]"="Invert Data Bits [LSB]", "Invert Opcode"="Invert Opcode", "Invert Address"="Invert Address") -> (w234:T10)  [unwired: 1 in]
        n72 = Bundle By Name(cluster=w234, "INI Path"=w201) -> (w209:T10)
        n73 = call <vilib>:"Add State(s) to Queue__jki_lib_state_machine.vi"("State(s) in Front (\"\")"="Initialize Core Data\nMacro: Initialize", "State(s) in (\"\")"=w236) -> ("States Out"=w235:string)  [unwired: 13 in]
        "Read Data" <- w219
        "Data Bytes Written" <- w219
        "Hex Table" <- w197
        "Bin Table" <- w197
        "Status" <- w183
        "Binary String_Load" <- w183
        "Binary String_Save" <- w183
        "Program Data Array" <- u8 0 ("Slide")
      }
      frame "Data: Update" {
        # "Update the master cluster for any config changes"
        n74 = Unbundle By Name(w247) -> ("Hex Table"=w246:string[][], "Bin Table"=w245:string[][])
        n75 = local write "Hex Table"(w246) -> ()
        n76 = local write "Bin Table"(w245) -> ()
        n77 = local read "Target Page Size (bytes)"() -> (w257:u32)
        n78 = local read "Bit Pattern (WRITE ALL)"() -> (w240:T4)
        n79 = local read "EEPROM Program Data"() -> (w244:string[][])
        n80 = local read "EEPROM Device Type"() -> (w250:T6)
        n81 = local read "Page Write Delay (ms)"() -> (w263:u8)
        n82 = local read "Bytes to Read"() -> (w259:u32)
        n83 = local read "Invert Data Bits [MSB]"() -> (w241:bool)
        n84 = local read "Invert Data Bits [LSB]"() -> (w239:bool)
        n85 = local read "Endianness (WRITE)"() -> (w249:bool)
        n86 = local read "NI845x Device ID"() -> (w253:T5)
        n87 = local read "Burst Width"() -> (w251:enum16{"8 bits", "16 bits", "32 bits"})
        n88 = local read "CLK Rate (kHz)"() -> (w256:u16)
        n89 = local read "Address Width"() -> (w261:enum16{"8 bits", "16 bits", "32 bits"})
        n90 = local read "Enable Debug?"() -> (w243:bool)
        n91 = local read "Invert Address"() -> (w237:bool)
        n92 = local read "Invert Opcode"() -> (w238:bool)
        n93 = local read "Device Mode"() -> (w252:enum16{"SPI", "I2C", "DIO"})
        n94 = local read "CS Idle Level"() -> (w262:enum16{"Low (Assert High)", "High (Assert Low)"})
        n95 = local read "Address"() -> (w258:u16)
        n96 = local read "WRITE Data"() -> (w242:u8[])
        n97 = local read "IO Level (V)"() -> (w254:i32)
        n98 = local read "CS/SS Line (0-6)"() -> (w255:u32)
        n99 = local read "Verbose?"() -> (w248:bool)
        n100 = call "CreateWriteCluster.vi"("Page Size in Bytes"=w257, "EEPROM Starting Address"=w258, "Number of Bytes to Write"=w259) -> ("Array of Write Cluster Information"=w260:T12)  [unwired: 1 in]
        n101 = Bundle By Name(cluster=w247, "EEPROM Device Type"=w250, "NI845x Device ID"=w253, "Device Mode"=w252, "IO Level (V)"=w254, "CS/SS Line (0-6)"=w255, "CLK Rate (kHz)"=w256, "Bit Pattern (WRITE ALL)"=w240, "Bytes to Read"=w259, "Target Page Size (bytes)"=w257, "Page Write Delay (ms)"=w263, "CS Idle Level"=w262, "script read index"=w261, "Burst Width"=w251, "Address"=w258, "Array of Write Cluster Information"=w260, "WRITE Data"=w242, "Invert Opcode"=w238, "Invert Address"=w237, "Endianness (WRITE)"=w249, "Verbose?"=w248, "Enable Debug?"=w243, "Invert Data Bits [MSB]"=w241, "Invert Data Bits [LSB]"=w239, "EEPROM Program Data"=w244) -> (w264:T10)
      }
      frame "Data: Cleanup" {
        # "Cleanup any data and references, here.\n(this is called automatically, by the Macro: Exit)"
        n102 = Unbundle By Name(w267) -> ("Core.Current VI Reference"=w270:refnum<vi>)
        n103 = Close Reference(reference=w270, error in (no error)=w269) -> (error out=w268:errorcluster)
      }
      frame "---------- UI ----------" {
        # "Do not put any code in this frame.\n(It is a separator no-op. You can make a copy of this frame to create a new UI frame)"
      }
      frame "UI: Initialize" {
        # "Initialize the User Interface, here.\n(this is called automatically, by the Macro: Init)"
      }
      frame "UI: Cursor Set" {
        # "Argument"
        # "Set and Unset Cursor Busy.\n(Usage: \"UI: Cursor Set >> Busy|Idle\")"
        n104 = case shown="\"Busy\"" w278 {
          tunnel: w280 -> [w284 w286]
          tunnel: [w283 w285] -> w279
          frame "Idle", Default {
            n105 = call <vilib>:"Unset Busy.vi"("error in (no error)"=w284) -> ("error out"=w283:errorcluster)  [unwired: 10 in]
          }
          frame "Busy" {
            n106 = call <vilib>:"Set Busy.vi"("error in (no error)"=w286) -> ("error out"=w285:errorcluster)  [unwired: 9 in, 1 out]
          }
        }
      }
      frame "UI: Front Panel State" {
        # "Argument"
        # "Set Front Panel Open or Closed\n(Usage: \"UI: Front Panel State >> Open|Close\")"
        n107 = Unbundle By Name(w289) -> ("Core.Current VI Reference"=w288:refnum<vi>)
        n108 = case shown="\"Minimize\", \"Minimized\"" w287 {
          tunnel: w291 -> [w298 w313 w324 w337 w350]
          tunnel: [w300 w314 w326 w339 w352] -> w290
          tunnel: w288 -> [w299 w311 w325 w338 w351]
          frame "Open", "Standard", Default {
            w293 = T7."Standard" ("State")
            n109 = property class="VI"(reference=w299, error in=w298) -> (reference out=w296:refnum<vi>, error out=w297:errorcluster, "FP.State"=w295:T7)
            n110 = Not Equal?(x=w295, y=w293) -> (x != y?=w294:bool)
            n111 = case shown="True" w294 {
              tunnel: [w304 w306] -> w300
              tunnel: w297 -> [w303 w306]
              tunnel: w296 -> [w302 _]
              tunnel: w293 -> [w301 _]
              frame True {
                n112 = invoke class="VI" method="FP.Open"(reference=w302, error in=w303, "Activate"=TRUE, "State"=w301) -> (error out=w304:errorcluster)  [unwired: 1 in, 4 out]
              }
              frame False {
              }
            }
          }
          frame "Close", "Closed" {
            n113 = property class="VI"(reference=w311, error in=w313) -> (reference out=w310:refnum<vi>, error out=w312:errorcluster, "FP.State"=w308:T7)
            n114 = Not Equal?(x=w308, y=T7."Closed" ("Front Panel Window:State")) -> (x != y?=w307:bool)
            n115 = case shown="True" w307 {
              tunnel: [w315 w318] -> w314
              tunnel: w312 -> [w315 w317]
              tunnel: w310 -> [_ w316]
              frame False {
              }
              frame True {
                n116 = invoke class="VI" method="FP.Close"(reference=w316, error in=w317) -> (error out=w318:errorcluster)  [unwired: 1 in, 2 out]
              }
            }
          }
          frame "Hidden", "Hide" {
            w319 = T7."Hidden" ("State")
            n117 = property class="VI"(reference=w325, error in=w324) -> (reference out=w322:refnum<vi>, error out=w323:errorcluster, "FP.State"=w321:T7)
            n118 = Not Equal?(x=w321, y=w319) -> (x != y?=w320:bool)
            n119 = case shown="True" w320 {
              tunnel: [w330 w331] -> w326
              tunnel: w323 -> [w329 w331]
              tunnel: w322 -> [w328 _]
              tunnel: w319 -> [w327 _]
              frame True {
                n120 = invoke class="VI" method="FP.Open"(reference=w328, error in=w329, "State"=w327) -> (error out=w330:errorcluster)  [unwired: 2 in, 4 out]
              }
              frame False {
              }
            }
          }
          frame "Minimize", "Minimized" {
            w332 = T7."Minimized" ("State")
            n121 = property class="VI"(reference=w338, error in=w337) -> (reference out=w335:refnum<vi>, error out=w336:errorcluster, "FP.State"=w334:T7)
            n122 = Not Equal?(x=w334, y=w332) -> (x != y?=w333:bool)
            n123 = case shown="True" w333 {
              tunnel: [w343 w344] -> w339
              tunnel: w336 -> [w342 w344]
              tunnel: w335 -> [w341 _]
              tunnel: w332 -> [w340 _]
              frame True {
                n124 = invoke class="VI" method="FP.Open"(reference=w341, error in=w342, "State"=w340) -> (error out=w343:errorcluster)  [unwired: 2 in, 4 out]
              }
              frame False {
              }
            }
          }
          frame "Maximize", "Maximized" {
            w345 = T7."Maximized" ("State")
            n125 = property class="VI"(reference=w351, error in=w350) -> (reference out=w348:refnum<vi>, error out=w349:errorcluster, "FP.State"=w347:T7)
            n126 = Not Equal?(x=w347, y=w345) -> (x != y?=w346:bool)
            n127 = case shown="True" w346 {
              tunnel: [w356 w357] -> w352
              tunnel: w349 -> [w355 w357]
              tunnel: w348 -> [w354 _]
              tunnel: w345 -> [w353 _]
              frame True {
                n128 = invoke class="VI" method="FP.Open"(reference=w354, error in=w355, "State"=w353) -> (error out=w356:errorcluster)  [unwired: 2 in, 4 out]
              }
              frame False {
              }
            }
          }
        }
      }
      frame "UI: Display Help" {
        n129 = call <vilib>:"Read JPEG File.vi"("error in (no error)"=w362, "path to JPEG file"=path "C:/projects/AldrinA_Test_Apps/NI-845x I2C-SPI Programmer GUI/NI8451_J6_wiring.jpg" ("Path")) -> ("error out"=w361:errorcluster, "image data"=w360:T13)  [unwired: 7 in, 1 out]
        n130 = call <vilib>:"Draw Flattened Pixmap.vi"("image data"=w360, "picture"=picture data[5B]) -> ("new picture"=w359:picture)  [unwired: 7 in]
        n131 = call "Picture Prompt.vi"("error in (no error)"=w361, "2D Picture 2"=w359) -> ("error out"=w364:errorcluster)  [unwired: 9 in]
      }
      frame "UI: Display Status" {
        # "// Command Format:  \"UI: Display Status >> [Window Title] [Message] [Timeout]\""
        n132 = call <vilib>:"Trim Whitespace.vi"("string"=w375) -> ("trimmed string"=w374:string)  [unwired: 1 in]
        n133 = Empty String/Path?(string/path=w374) -> (empty?=w372:bool)
        n134 = case shown="False" w372 {
          tunnel: w374 -> [w389 _]
          tunnel: [w386 w390] -> w370
          tunnel: [w385 w390] -> w368
          tunnel: [w379 -1] -> w367
          frame False {
            w382 = string[] ["[", "]"] ("delimiters (\\s,\\t,\\r,\\n)")
            n135 = Scan String For Tokens(6:w382, 9:w389) -> (1:w386:string, 2:w388:i32, 3:w387:string)  [unwired: 4 in, 1 out]
            n136 = Scan String For Tokens(6:w382, 8:w388, 9:w387) -> (1:w385:string, 2:w383:i32, 3:w384:string)  [unwired: 3 in, 1 out]
            n137 = Scan String For Tokens(6:w382, 8:w383, 9:w384) -> (1:w381:string)  [unwired: 3 in, 3 out]
            n138 = Decimal String To Number(string=w381, default (0L)=10000 ("Timeout (-1)")) -> (number=w379:i32)  [unwired: 1 in, 1 out]
          }
          frame True {
            w390 = "Important Message" ("token string")
          }
        }
        n139 = Wait (ms)(milliseconds to wait=w367) -> ()  [unwired: 1 out]
        n140 = Format Into String(format string="\n%s", initial string=w370, error in=w376, w368) -> (resulting string=w371:string, error out=w377:errorcluster)
        n141 = local write "Status"(w371) -> ()
      }
      frame "UI: Display Dialog" {
        # "// Command Format:  \"UI: Display Dialog >> [Window Title] [Message] [Timeout]\""
        n142 = Unbundle By Name(w393) -> ("Verbose?"=w392:bool)
        n143 = call <vilib>:"Trim Whitespace.vi"("string"=w395) -> ("trimmed string"=w394:string)  [unwired: 1 in]
        n144 = case shown="True" w392 {
          tunnel: [w399 w408] -> w397
          tunnel: w396 -> [w399 w407]
          tunnel: w394 -> [_ w406]
          frame False {
          }
          frame True {
            n145 = Empty String/Path?(string/path=w406) -> (empty?=w400:bool)
            n146 = case shown="False" w400 {
              tunnel: w406 -> [w419 _]
              tunnel: [w416 w420] -> w403
              tunnel: [w415 w420] -> w402
              tunnel: [w409 -1] -> w401
              frame False {
                w412 = string[] ["[", "]"] ("delimiters (\\s,\\t,\\r,\\n)")
                n147 = Scan String For Tokens(6:w412, 9:w419) -> (1:w416:string, 2:w418:i32, 3:w417:string)  [unwired: 4 in, 1 out]
                n148 = Scan String For Tokens(6:w412, 8:w418, 9:w417) -> (1:w415:string, 2:w413:i32, 3:w414:string)  [unwired: 3 in, 1 out]
                n149 = Scan String For Tokens(6:w412, 8:w413, 9:w414) -> (1:w411:string)  [unwired: 3 in, 3 out]
                n150 = Decimal String To Number(string=w411, default (0L)=10000 ("Timeout (-1)")) -> (number=w409:i32)  [unwired: 1 in, 1 out]
              }
              frame True {
                w420 = "Important Message" ("token string")
              }
            }
            n151 = call <vilib>:"Init Dialog__lava_lib_ui_tools.vi"("error in (no error)"=w407, "Timeout (-1)"=w401, "Message"=w402, "Dialog Title"=w403) -> ("error out"=w404:errorcluster, "Dialog out"=w405:refnum<class "Dialog__lava_lib_ui_tools.lvclass">)  [unwired: 6 in]
            n152 = while {
              tunnel: w405 -> [w429]
              shift-right: [w427] -> w408
              shift-left: w404 -> [w428]
              stop <- w424 stop-if-true
              n153 = call-dynamic "Dialog Box__lava_lib_ui_tools.vi"("error in (no error)"=w428, "Dialog in"=w429) -> ("error out"=w427:errorcluster, "timed out?"=w423:bool, "Selection"=w426:string)  [unwired: 6 in, 1 out]
              n154 = case shown="\"False\", Default" w426 {
                tunnel: [TRUE FALSE] -> w425
                frame "False", Default {
                }
                frame "True" {
                }
              }
              n155 = Or(x=w425, y=w423) -> (x .or. y?=w424:bool)
              n156 = Wait (ms)(milliseconds to wait=u32 100) -> ()  [unwired: 1 out]
            }
          }
        }
      }
      frame "---------- Macro ----------" {
        # "Do not put any code in this frame.\n(It is a separator no-op. You can make a copy of this frame to create a new Macro frame)"
      }
      frame "Macro: Initialize" {
        w438 = string[][] [] ("Hex Table")
        w444 = string[] ["Address", "1", "2", "3", "4"] ("Column Header Strings[]")
        w440 = FALSE ("QUIT")
        w453 = "UI: Initialize\nUI: Front Panel State >> Open\nMacro: Load Config INI\nData: Update"  # UI: Initialize UI: Front Panel State >> Open Macro: Load Config INI Data: Update
        # "Initialization Macro\n(This is called once, when the VI starts)"
        n157 = property on="Hex Table" class="Tbl (strict)"(error in=w447, "Column Headers[]"=w444, "Number of Columns"=u32 5, "Value"=w438) -> (error out=w445:errorcluster)  [unwired: 1 in, 1 out]
        n158 = property on="Bin Table" class="Tbl (strict)"(error in=w445, "Column Headers[]"=w444, "Number of Columns"=u32 5, "Value"=w438) -> (error out=w439:errorcluster)  [unwired: 1 in, 1 out]
        n159 = property on="EEPROM Program Data" class="Tbl (strict)"(error in=w439, "Column Headers[]"=string[] ["Address", "Data"] ("Column Header Strings[]"), "Number of Columns"=u32 2, "Value"=w438) -> (error out=w435:errorcluster)  [unwired: 1 in, 1 out]
        n160 = property on="QUIT" class="Bool (strict)"(error in=w435, "Value"=w440) -> (error out=w449:errorcluster)  [unwired: 1 in, 1 out]
        n161 = property on="Read ALL Device" class="Bool (strict)"(error in=w449, "Value"=w440) -> (error out=w450:errorcluster)  [unwired: 1 in, 1 out]
        n162 = property on="Write Device" class="Bool (strict)"(error in=w450, "Value"=w440) -> (error out=w451:errorcluster)  [unwired: 1 in, 1 out]
        n163 = property on="Write ALL Device" class="Bool (strict)"(error in=w451, "Value"=w440) -> (error out=w452:errorcluster)  [unwired: 1 in, 1 out]
        n164 = property on="Erase ALL Device" class="Bool (strict)"(error in=w452, "Value"=w440) -> (error out=w448:errorcluster)  [unwired: 1 in, 1 out]
        n165 = property on="Help" class="Bool (strict)"(error in=w448, "Value"=w440) -> (error out=w442:errorcluster)  [unwired: 1 in, 1 out]
        n166 = property on="Config INI Save" class="Bool (strict)"(error in=w442, "Value"=w440) -> (error out=w441:errorcluster)  [unwired: 1 in, 1 out]
        n167 = call <vilib>:"Add State(s) to Queue__jki_lib_state_machine.vi"("State(s) in Front (\"\")"=w453, "State(s) in (\"\")"=w456) -> ("States Out"=w455:string)  [unwired: 13 in]
      }
      frame "Macro: Exit" {
        # "// connecting this will close\nthe window immediately.\n// disconnect to keep window\nopen to re-launch when needed"
        # "Exit Macro\n(This is called once, when the VI exits)"
        n168 = Unbundle By Name(w463) -> ()  [unwired: 1 out]
        n169 = Select(t="UI: Front Panel State >> Close", s=FALSE, f="") -> (s? t:f=w460:string)
        n170 = call <vilib>:"Add State(s) to Queue__jki_lib_state_machine.vi"("State(s) in (\"\")"=w460, "State(s) at Back (\"\")"="Data: Cleanup\nMacro: Save Config INI\nUI: Cursor Set >> Idle\nExit") -> ("States Out"=w458:string)  [unwired: 13 in]
        n171 = call <vilib>:"Add State(s) to Queue__jki_lib_state_machine.vi"("State(s) in Front (\"\")"=w458, "State(s) in (\"\")"=w466) -> ("States Out"=w465:string)  [unwired: 13 in]
      }
      frame "Macro: Build Hex-Bin Table-READ" {
        w474 = string[][] [] ("array")
        # "Update the Hex strings display post data capture from device"
        n172 = Unbundle By Name(w477) -> ("Address"=w471:u16, "Read Data"=w470:u8[], "Target Page Size (bytes)"=w467:u32)
        n173 = for {
          N: 1 -> [_]
          shift-right: [w499] -> w473
          shift-left: w474 -> [w498]
          shift-right: [w492] -> w472
          shift-left: w474 -> [w491]
          tunnel: w467 -> [w490]
          tunnel: w471 -> [w488]
          tunnel: w470 -> [w483]
          tunnel: string[] [] ("array") -> [w482]
          i -> [w489]
          w486 = ""
          # "This is how many 8-bit columns\nare displayed on Hex-Bin tables"
          n174 = for {
            tunnel: w483 -> [w514] mode=indexing
            shift-right: [w512] -> _
            shift-left: w486 -> [w511]
            shift-right: [w510] -> _
            shift-left: w486 -> [w509]
            shift-right: [w507] -> w484
            shift-left: w482 -> [w505]
            shift-right: [w501] -> w485
            shift-left: w482 -> [w502]
            i -> [w504]
            w508 = "\t"
            n175 = Number To Hexadecimal String(2:w514) -> (0:w513:string)  [unwired: 1 in]
            n176 = call "Hex_String_to_Binary_String.vi"("bitness"=enum16{"8", "16", "32", "64"}."8", "Hexadecimal String"=w513) -> ("Hex String"=w506:string, "Binary String"=w503:string)  [unwired: 1 in, 1 out]
            n177 = Concatenate Strings(w511, w503, w508) -> (w512:string)
            n178 = Insert Into Array(array=w502, index=w504, new element=w503) -> (w501:string[])
            n179 = Concatenate Strings(w509, w506, w508) -> (w510:string)
            n180 = Insert Into Array(array=w505, index=w504, new element=w506) -> (w507:string[])
          }
          n181 = Number To Hexadecimal String(1:i16 4 ("width (-)"), 2:w488) -> (0:w494:string)
          n182 = Increment(x=w490) -> (x+1=w481:u32)
          n183 = Build Array (concatenate)(w494, w484) -> (w497:string[])
          n184 = Build Array (concatenate)(w494, w485) -> (w495:string[])
          n185 = Reshape Array(w497, w481) -> (w496:string[])
          n186 = Reshape Array(w495, w481) -> (w493:string[])
          n187 = Insert Into Array(array=w491, index (row)=w489, new element=w493) -> (w492:string[][])  [unwired: 1 in]
          n188 = Insert Into Array(array=w498, index (row)=w489, new element=w496) -> (w499:string[][])  [unwired: 1 in]
        }
        n189 = local write "Bin Table"(w472) -> ()
        n190 = local write "Hex Table"(w473) -> ()
        n191 = call <vilib>:"Add State(s) to Queue__jki_lib_state_machine.vi"("State(s) in Front (\"\")"="UI: Display Status >>  [Alert!][Hex & Binary Table Parsed][100]" ("State(s) in Front (\"\")"), "State(s) in (\"\")"=w480) -> ("States Out"=w479:string)  [unwired: 13 in]
        n192 = Bundle By Name(cluster=w477, "Bin Table"=w472, "Hex Table"=w473) -> (w476:T10)
      }
      frame "Macro: Build Hex-Bin Table-READ-ALL" {
        w525 = string[][] [] ("array")
        # "// always start READ from address  0x000 to max address of chip"
        # "Update the Hex strings display post data capture from device"
        n193 = Unbundle By Name(w528) -> ("EEPROM Device Type"=w518:T6, "Read Data"=w521:u8[], "Target Page Size (bytes)"=w516:u32)
        n194 = case shown="\"ST-M93C86\"" w518 {
          tunnel: [u32 130 ("number") u32 2048 ("number") u32 2048 ("number") u32 2048 ("number") u32 2048 ("number")] -> w517
          frame "Microchip LC56BT" {
          }
          frame "Microchip 93LC86C [8451]" {
          }
          frame "Microchip 93LC86C [8452]" {
          }
          frame "ST-M93C86" {
          }
          frame "Generic EEPROM", Default {
          }
        }
        n195 = Quotient & Remainder(x=w517, y=w516) -> (floor(x/y)=w515:u32)  [unwired: 1 out]
        n196 = To Long Integer(number=u16 0) -> (32bit integer=w519:i32)
        n197 = for {
          N: w515 -> [_]
          shift-right: [w558] -> _
          shift-left: w521 -> [w557]
          shift-right: [w556] -> w524
          shift-left: w525 -> [w555]
          shift-right: [w549] -> w523
          shift-left: w525 -> [w548]
          tunnel: string[] [] ("array") -> [w540]
          tunnel: w516 -> [w539]
          tunnel: w519 -> [w537]
          i -> [w544]
          w545 = ""
          # "Extract n bytes at a time (per page size)\nRemaining elements to shift register"
          n198 = Delete From Array(array=w557, length=w539, index=0) -> (deleted portion=w559:u8[], array with subset deleted=w558:u8[])
          n199 = for {
            tunnel: w559 -> [w574] mode=indexing
            shift-right: [w572] -> _
            shift-left: w545 -> [w571]
            shift-right: [w570] -> _
            shift-left: w545 -> [w569]
            shift-right: [w567] -> w543
            shift-left: w540 -> [w565]
            shift-right: [w561] -> w542
            shift-left: w540 -> [w562]
            i -> [w564]
            w568 = "\t"
            n200 = Number To Hexadecimal String(2:w574) -> (0:w573:string)  [unwired: 1 in]
            n201 = call "Hex_String_to_Binary_String.vi"("bitness"=enum16{"8", "16", "32", "64"}."8", "Hexadecimal String"=w573) -> ("Hex String"=w566:string, "Binary String"=w563:string)  [unwired: 1 in, 1 out]
            n202 = Concatenate Strings(w571, w563, w568) -> (w572:string)
            n203 = Insert Into Array(array=w562, index=w564, new element=w563) -> (w561:string[])
            n204 = Concatenate Strings(w569, w566, w568) -> (w570:string)
            n205 = Insert Into Array(array=w565, index=w564, new element=w566) -> (w567:string[])
          }
          n206 = Add(x=w537, y=w544) -> (x+y=w538:i32)
          n207 = Number To Hexadecimal String(1:i16 4 ("width (-)"), 2:w538) -> (0:w551:string)
          n208 = Increment(x=w539) -> (x+1=w541:u32)
          n209 = Build Array (concatenate)(w551, w543) -> (w554:string[])
          n210 = Build Array (concatenate)(w551, w542) -> (w552:string[])
          n211 = Reshape Array(w554, w541) -> (w553:string[])
          n212 = Reshape Array(w552, w541) -> (w550:string[])
          n213 = Insert Into Array(array=w548, index (row)=w544, new element=w550) -> (w549:string[][])  [unwired: 1 in]
          n214 = Insert Into Array(array=w555, index (row)=w544, new element=w553) -> (w556:string[][])  [unwired: 1 in]
        }
        n215 = local write "Bin Table"(w523) -> ()
        n216 = local write "Hex Table"(w524) -> ()
        n217 = call <vilib>:"Add State(s) to Queue__jki_lib_state_machine.vi"("State(s) in Front (\"\")"="UI: Display Status >>  [Alert!][Hex & Binary Table Parsed][100]" ("State(s) in Front (\"\")"), "State(s) in (\"\")"=w531) -> ("States Out"=w530:string)  [unwired: 13 in]
        n218 = Bundle By Name(cluster=w528, "Bin Table"=w523, "Hex Table"=w524) -> (w527:T10)
      }
      frame "Macro: Build Program Data" {
        n219 = Unbundle By Name(w584) -> ("EEPROM Device Type"=w582:T6, "Target Page Size (bytes)"=w580:u32, "WRITE Data"=w583:u8[])
        n220 = case shown="\"Microchip 93LC86C [8452]\"" w582 {
          tunnel: [u32 128 ("number") u32 2050 ("number") u32 2048 ("number") u32 2048 ("number") u32 2048 ("number")] -> w581
          frame "Microchip LC56BT" {
          }
          frame "Microchip 93LC86C [8451]" {
          }
          frame "Microchip 93LC86C [8452]" {
          }
          frame "ST-M93C86" {
          }
          frame "Generic EEPROM", Default {
          }
        }
        n221 = Quotient & Remainder(x=w581, y=w580) -> (floor(x/y)=w579:u32)  [unwired: 1 out]
        n222 = Initialize Array("", w579, 2 ("dimension size")) -> (w576:string[][])
        n223 = for {
          N: w579 -> [_]
          tunnel: w580 -> [_]
          shift-right: [w610] -> w575
          shift-left: w576 -> [w611]
          shift-right: [w602] -> _
          shift-left: w583 -> [w604]
          i -> [w605]
          w612 = i16 4 ("width (-)")
          n224 = for {
            N: 2 -> [_]
            tunnel: [w616] -> w600
            tunnel: w604 -> [w619]
            tunnel: [w617] -> w602
            n225 = Delete From Array(array=w619, length=2, index=0) -> (deleted portion=w616:u8[], array with subset deleted=w617:u8[])
          }
          n226 = Add(x=u16 0 ("number"), y=w605) -> (x+y=w613:i32)
          n227 = To Unsigned Word Integer(number=w613) -> (unsigned 16bit integer=w601:u16)
          n228 = Number To Hexadecimal String(1:w612, 2:w601) -> (0:w608:string)
          n229 = Index Array(array=w600, index #1=0 ("index")) -> (element #1=w597:u8, element #2=w598:u8)  [unwired: 1 in]
          n230 = Join Numbers(hi=w597, lo=w598) -> ((hi.lo)=w596:u16)
          n231 = To Unsigned Word Integer(number=w596) -> (unsigned 16bit integer=w595:u16)
          n232 = Number To Hexadecimal String(1:w612, 2:w595) -> (0:w606:string)
          n233 = Replace Array Subset(array=w611, new element #1=w608, index (row) #1=w605, index (col) #1=0 ("disabled index (col)"), new element #2=w606, index (row) #2=w605, index (col) #2=1 ("index (row)")) -> (w610:string[][])
        }
        n234 = Bundle By Name(cluster=w584, "EEPROM Program Data"=w575, "EEPROM Binary File Array"=w575) -> (w588:T10)
        n235 = call <vilib>:"Add State(s) to Queue__jki_lib_state_machine.vi"("State(s) in Front (\"\")"="UI: Display Status >>  [Alert!][Build Program Data Completed][100]" ("State(s) in Front (\"\")"), "State(s) in (\"\")"=w587) -> ("States Out"=w586:string)  [unwired: 13 in]
      }
      frame "Macro: Load Binary File" {
        w633 = u8 0  # u8
        # "Use this string indicator to calculate the MD5 fingerprint"
        n236 = Unbundle By Name(w639) -> ("Burst Width"=w637:enum16{"8 bits", "16 bits", "32 bits"}, "Endianness (WRITE)"=w636:bool)
        n237 = case shown="True" w636 {
          tunnel: [T9."big-endian, network order" ("byte order (0:big-endian, network order)") T9."little-endian" ("byte order (0:big-endian, network order)")] -> w635
          frame True {
          }
          frame False {
          }
        }
        n238 = case shown="\"16 bits\"" w637 {
          tunnel: [u8[] [] u16[] [] u32[] []] -> _
          frame "8 bits" {
          }
          frame "16 bits" {
          }
          frame "32 bits" {
          }
        }
        n239 = Read from Binary File(5:w633, 8:w640, 9:w635, 10:-1 ("count (1)"), 11:"Path to BIN file") -> (0:w629:errorcluster, 2:w631:u8[])  [unwired: 1 in, 2 out]
        n240 = Byte Array To String(unsigned byte array=w631) -> (string=w630:string)
        n241 = Bundle By Name(cluster=w639, "WRITE Data"=w631) -> (w638:T10)
        n242 = local write "Binary String_Load"(w630) -> ()
        n243 = call-poly <userlib>:"MD5 Message Digest__ogtk.vi"("Message"=w630) -> ("MD5 Message Digest"=w627:string)
        "MD5_Calc" <- w627
        n244 = Read from Text File(file (use dialog)="Path to MD5 Fingerprint", error in=w629) -> (text=w626:string, error out=w624:errorcluster)  [unwired: 2 in, 2 out]
        "MD5_File" <- w626
        n245 = Equal?(x=w627, y=w626) -> (x = y?=w625:bool)
        n246 = case shown="True" w625 {
          tunnel: w624 -> [_ w647]
          tunnel: [errorcluster {"status"=TRUE, "code"=1, "source"="MD5 Checksum Mismatched!!"} ("error out") w647] -> w623
          tunnel: w622 -> [_ w646]
          tunnel: [w642 w645] -> w621
          tunnel: "NI845x: EWDS\nNI845x: Run Script - Close SPI - Close Device\nUI: Display Status >>  [Alert!][MD5 Fingerprint (Checksum) Verification Failed][3000]\nUI: Cursor Set >> Idle\nMacro: Exit" ("State(s) in Front (\"\")") -> [w641 _]
          frame False {
            # "MD5 Checksum Mismatched"
            n247 = call <vilib>:"Add State(s) to Queue__jki_lib_state_machine.vi"("State(s) in (\"\")"=w641) -> ("States Out"=w642:string)  [unwired: 14 in]
          }
          frame True {
            # "Checksum Matches"
            n248 = call <vilib>:"Add State(s) to Queue__jki_lib_state_machine.vi"("State(s) in Front (\"\")"="UI: Display Status >>  [Alert!][Checksum Check Passed][3000]" ("State(s) in Front (\"\")"), "State(s) in (\"\")"=w646) -> ("States Out"=w645:string)  [unwired: 13 in]
          }
        }
      }
      frame "Macro: Save Binary File" {
        # "// Prepends the string length at start of binary file\n// in this case it will add 0x00 0x00 0x08 0x02 at\n// the beginning of the file."
        n249 = Unbundle By Name(w675) -> ("Read Data"=w672:u8[], "Endianness (WRITE)"=w674:bool)
        n250 = control-ref of="This VI"() -> (w664:refnum<vi>)
        n251 = property class="VI"(reference=w664, error in=w665) -> (error out=w666:errorcluster, "Name"=w662:string)  [unwired: 1 out]
        n252 = case shown="True" w674 {
          tunnel: [T9."big-endian, network order" ("byte order (0:big-endian, network order)") T9."little-endian" ("byte order (0:big-endian, network order)")] -> w673
          frame True {
          }
          frame False {
          }
        }
        n253 = Match Pattern(string=w662, regular expression="[.]" ("search string")) -> (before substring=w654:string)  [unwired: 1 in, 3 out]
        n254 = Byte Array To String(unsigned byte array=w672) -> (string=w667:string)
        n255 = call "AMCTRDV Create File Path Type.vi"("File Type"=".bin", "Filename-Description"=w654, "Timestamp?"=FALSE, "Folder Name"=w654, "Serial #"="") -> ("File Path"=w658:path)  [unwired: 2 in]
        n256 = Write to Binary File(file (use dialog)=w658, data=w667, error in=w666, 5:FALSE ("prepend array or string size? (T)"), 9:w673) -> (error out=w670:errorcluster)  [unwired: 1 in, 2 out]
        n257 = call "AMCTRDV Create File Path Type.vi"("File Type"=".md5", "Filename-Description"=w654, "Timestamp?"=FALSE, "Folder Name"=w654, "Serial #"="") -> ("File Path"=w653:path)  [unwired: 2 in]
        n258 = local write "Binary String_Save"(w667) -> ()
        n259 = call-poly <userlib>:"MD5 Message Digest__ogtk.vi"("Message"=w667) -> ("MD5 Message Digest"=w669:string)
        n260 = Write to Text File(file (use dialog)=w653, text=w669, error in=w670) -> (error out=w668:errorcluster)  [unwired: 1 in, 2 out]
      }
      frame "Macro: Save Config INI" {
        # "// Save control values & states to INI file\n// Config.INI saved in directory as this VI"
        n261 = Unbundle By Name(w684) -> ("INI Path"=w683:path)
        n262 = control-ref of="This VI"() -> (w685:refnum<vi>)
        n263 = call "Utility Write Config INI to File.vi"("File Type"=".ini", "Error In"=w688, "reference"=w685, "Path In"=w683) -> ("Error Out"=w687:errorcluster, "Path Out"=w682:path)  [unwired: 6 in]
        n264 = Path To String(path=w682) -> (string=w680:string)
        n265 = Format Into String(format string="UI: Display Status >> [Configuration INI Saved To PATH: ][%s][100]" ("State(s) in Front (\"\")"), w680) -> (resulting string=w679:string)  [unwired: 2 in, 1 out]
        n266 = call <vilib>:"Add State(s) to Queue__jki_lib_state_machine.vi"("State(s) in Front (\"\")"=w679, "State(s) in (\"\")"=w690) -> ("States Out"=w689:string)  [unwired: 13 in]
      }
      frame "Macro: Load Config INI" {
        n267 = Unbundle By Name(w693) -> ("INI Path"=w692:path)
        n268 = control-ref of="This VI"() -> (w700:refnum<vi>)
        n269 = call "Utility Load Config INI from File.vi"("File Type"=".ini", "Error In"=w697, "reference"=w700, "Path In"=w692) -> ("Error Out"=w696:errorcluster, "Path Out"=w699:path)  [unwired: 6 in]
        n270 = Path To String(path=w699) -> (string=w694:string)
        n271 = Format Into String(format string="UI: Display Status >> [Configuration INI Loaded From PATH: ][%s][100]" ("State(s) in Front (\"\")"), w694) -> (resulting string=w691:string)  [unwired: 2 in, 1 out]
        n272 = call <vilib>:"Add State(s) to Queue__jki_lib_state_machine.vi"("State(s) in Front (\"\")"=w691, "State(s) in (\"\")"=w702) -> ("States Out"=w701:string)  [unwired: 13 in]
      }
      frame "---------- NI845x: Template ----------" {
        # "Template Separator\n(You can make a copy of, or modify, this frame)"
      }
      frame "NI-845x Notes" {
        # "Template Separator\n(You can make a copy of, or modify, this frame)"
      }
      frame "93LC56BT Notes" {
        # "Template Separator\n(You can make a copy of, or modify, this frame)"
        n273 = disable-structure shown="Enabled" {
          frame Enabled {
          }
          frame Disabled {
          }
          frame Disabled {
          }
        }
      }
      frame "93C86 Notes" {
        # "Microchip 93C76/86 8K/16K 5.0V Microwire Serial EEPROM"
        n274 = disable-structure shown="Enabled" {
          frame Enabled {
          }
          frame Disabled {
          }
          frame Disabled {
          }
        }
      }
      frame "NI845x: Device Mode" {
        # "Send Message if Mode is not yet supported\nCommand Format:  \"UI: Display Status >> [Window Title] [Message] [Timeout]\""
        n275 = Unbundle By Name(w718) -> ("Device Mode"=w717:enum16{"SPI", "I2C", "DIO"})
        n276 = case shown="\"SPI\", Default" w717 {
          tunnel: ["UI: Display Status >>  [Alert!][SPI Device Mode Set][100]" "UI: Display Status >>  [Alert!][I2C Mode is NOT supported at this time][100]\n" "UI: Display Status >>  [Alert!][DIO Mode is NOT supported at this time][100]"] -> w715
          frame "SPI", Default {
          }
          frame "I2C" {
          }
          frame "DIO" {
          }
        }
        n277 = call <vilib>:"Add State(s) to Queue__jki_lib_state_machine.vi"("State(s) in Front (\"\")"=w715, "State(s) in (\"\")"=w716) -> ("States Out"=w720:string)  [unwired: 13 in]
      }
      frame "NI845x: Init SPI" {
        # "The Microchip EEPROMs' CS idle\nstate is LOW and asserted HIGH\nso set SPI to LOW post INIT."
        # "Step 1: Set the I/O reference voltage:\n\nNot all NI-845x hardware support all voltage levels. \nPlease consult your hardware documentation for more information.\n\nStep 2: Create the script and configure the SPI bus:\n\na) Create the script\nb) Switch the SPI bus pins into master mode. \n    This automatically sets all CS lines to be high.\nc) Configure the Phase and Plarity to mode 0, in \n    which the polarity and phase are both set to \n    zero, however this may be configured for \n    other EEPROMs. \nd) Configure the Clock rate as set by the front \n    panel control."
        # "NI845x only supports 8-bits per sample. \nNI8452 supports 8-64 bits per sample."
        n278 = Unbundle By Name(w742) -> ("Burst Width"=w731:enum16{"8 bits", "16 bits", "32 bits"}, "EEPROM Device Type"=w732:T6, "CS/SS Line (0-6)"=w739:u32, "CLK Rate (kHz)"=w740:u16, "NI845x Device ID"=w727:T5, "IO Level (V)"=w728:i32, "CLK Polarity (CPOL)"=w738:i32, "CLK Phase (CPHS)"=w737:i32)
        n279 = property class="NI-845x Device"(reference=w727, error in=w730, "IoVoltLevel"=w728) -> (error out=w729:errorcluster)  [unwired: 1 out]
        n280 = call "NI-845x SPI Create Script Reference.vi"("error in (no error)"=w729) -> ("error out"=w745:errorcluster, "spi script reference"=w741:T1)  [unwired: 9 out]
        n281 = call "NI-845x SPI Script Enable SPI.vi"("error in (no error)"=w745, "spi script reference in"=w741) -> ("error out"=w746:errorcluster, "spi script reference out"=w747:T1)  [unwired: 8 out]
        n282 = Bundle By Name(cluster=w742, "SPI Script Reference"=w741) -> (w734:T10)
        n283 = call "NI-845x SPI Script Clock Polarity Phase.vi"("error in (no error)"=w746, "clock phase (0)"=w737, "clock polarity (0)"=w738, "spi script reference in"=w747) -> ("error out"=w743:errorcluster, "spi script reference out"=w744:T1)  [unwired: 2 in, 4 out]
        n284 = call "NI-845x SPI Script Clock Rate.vi"("error in (no error)"=w743, "clock rate in kHz (1000)"=w740, "spi script reference in"=w744) -> ("error out"=w748:errorcluster, "spi script reference out"=w749:T1)  [unwired: 1 in, 6 out]
        n285 = call "NI-845x SPI Script CS Low.vi"("error in (no error)"=w748, "chip select (0)"=w739, "spi script reference in"=w749) -> ("error out"=w736:errorcluster, "spi script reference out"=w733:T1)  [unwired: 7 in]
        n286 = case shown="\"ST-M93C86\"" w732 {
          tunnel: w736 -> [w751 w756 w773 w775 w780]
          tunnel: [w751 w755 w773 w775 w779] -> w735
          tunnel: w733 -> [w750 w753 w772 w774 w777]
          tunnel: [w750 w754 w772 w774 w778] -> _
          tunnel: w731 -> [_ w752 _ _ w776]
          frame "Generic EEPROM", Default {
            # "NI-8451 is 8-bit ONLY"
          }
          frame "ST-M93C86" {
            # "Change to 16 bits with NI8452"
            n287 = case shown="\"16 bits\", Default" w752 {
              tunnel: w756 -> [w761 w766 w771]
              tunnel: w753 -> [w760 w765 w770]
              tunnel: [w759 w764 w769] -> w754
              tunnel: [w758 w763 w768] -> w755
              frame "8 bits" {
                n288 = call "NI-845x SPI Script Num Bits Per Sample.vi"("error in (no error)"=w761, "num bits per sample (8)"=u16 8, "spi script reference in"=w760) -> ("error out"=w758:errorcluster, "spi script reference out"=w759:T1)  [unwired: 7 in]
              }
              frame "16 bits", Default {
                n289 = call "NI-845x SPI Script Num Bits Per Sample.vi"("error in (no error)"=w766, "num bits per sample (8)"=u16 16, "spi script reference in"=w765) -> ("error out"=w763:errorcluster, "spi script reference out"=w764:T1)  [unwired: 7 in]
              }
              frame "32 bits" {
                n290 = call "NI-845x SPI Script Num Bits Per Sample.vi"("error in (no error)"=w771, "num bits per sample (8)"=u16 32, "spi script reference in"=w770) -> ("error out"=w768:errorcluster, "spi script reference out"=w769:T1)  [unwired: 7 in]
              }
            }
          }
          frame "Microchip LC56BT" {
            # "NI-8451 is 8-bit ONLY"
          }
          frame "Microchip 93LC86C [8451]" {
            # "NI-8451 is 8-bit ONLY"
          }
          frame "Microchip 93LC86C [8452]" {
            # "Change to 16 bits with NI8452"
            n291 = case shown="\"8 bits\"" w776 {
              tunnel: w780 -> [w785 w790 w795]
              tunnel: w777 -> [w784 w789 w794]
              tunnel: [w783 w788 w793] -> w778
              tunnel: [w782 w787 w792] -> w779
              frame "8 bits" {
                n292 = call "NI-845x SPI Script Num Bits Per Sample.vi"("error in (no error)"=w785, "num bits per sample (8)"=u16 8, "spi script reference in"=w784) -> ("error out"=w782:errorcluster, "spi script reference out"=w783:T1)  [unwired: 7 in]
              }
              frame "16 bits", Default {
                n293 = call "NI-845x SPI Script Num Bits Per Sample.vi"("error in (no error)"=w790, "num bits per sample (8)"=u16 16, "spi script reference in"=w789) -> ("error out"=w787:errorcluster, "spi script reference out"=w788:T1)  [unwired: 7 in]
              }
              frame "32 bits" {
                n294 = call "NI-845x SPI Script Num Bits Per Sample.vi"("error in (no error)"=w795, "num bits per sample (8)"=u16 32, "spi script reference in"=w794) -> ("error out"=w792:errorcluster, "spi script reference out"=w793:T1)  [unwired: 7 in]
              }
            }
          }
        }
        n295 = call <vilib>:"Add State(s) to Queue__jki_lib_state_machine.vi"("State(s) in Front (\"\")"="UI: Display Status >>  [Alert!][INIT SPI Completed][100]" ("State(s) in Front (\"\")"), "State(s) in (\"\")"=w726) -> ("States Out"=w725:string)  [unwired: 13 in]
      }
      frame "NI845x: EWEN" {
        # "1. Send SB & EWEN Opcode for 93LC56BT\n2. A dummy address byte\n3. A dummy data byte"
        n296 = Unbundle By Name(w812) -> ("EEPROM Device Type"=w809:T6, "EWEN"=w810:u8, "SPI Script Reference"=w811:T1, "CS/SS Line (0-6)"=w803:u32)
        n297 = case shown="\"Microchip 93LC86C [8452]\"" w809 {
          tunnel: [w822 w825 w829 w831 w835] -> w818
          tunnel: w810 -> [w821 w824 w828 w830 w834]
          frame "Generic EEPROM", Default {
            w823 = u8 0
            # "16-bit Data & 8-bit Address"
            n298 = Build Array(w821, w823, w823) -> (w822:u8[])
          }
          frame "Microchip LC56BT" {
            w826 = u8 0
            # "16-bit Data & 8-bit Address"
            n299 = Build Array(w824, w826, w826) -> (w825:u8[])
          }
          frame "ST-M93C86" {
            w827 = u16 0
            # "16-bit Data & Address"
            n300 = Build Array(w828, w827, w827) -> (w829:u16[])
          }
          frame "Microchip 93LC86C [8451]" {
            w832 = u8 0
            # "16-bit Data & 8-bit Address"
            n301 = Build Array(w830, w832, w832) -> (w831:u8[])
          }
          frame "Microchip 93LC86C [8452]" {
            w833 = u8 0
            # "16-bit Data & Address"
            n302 = Build Array(w834, w833, w833, w833) -> (w835:u8[])
          }
        }
        n303 = call "NI-845x SPI Script CS High.vi"("error in (no error)"=w813, "chip select (0)"=w803, "spi script reference in"=w811) -> ("error out"=w814:errorcluster, "spi script reference out"=w815:T1)  [unwired: 7 in]
        n304 = call "NI-845x SPI Script Write Read.vi"("error in (no error)"=w814, "write data"=w818, "spi script reference in"=w815) -> ("error out"=w816:errorcluster, "spi script reference out"=w817:T1)  [unwired: 1 in, 6 out]
        n305 = call "NI-845x SPI Script CS Low.vi"("error in (no error)"=w816, "chip select (0)"=w803, "spi script reference in"=w817) -> ("error out"=w808:errorcluster, "spi script reference out"=w807:T1)  [unwired: 7 in]
        n306 = call-poly "NI-845x SPI Script Delay.vi"("error in (no error)"=w808, "delay in microseconds (0)"=u16 1, "spi script reference in"=w807) -> ("error out"=w805:errorcluster, "spi script reference out"=w804:T1)  [unwired: 7 in]
        n307 = call "NI-845x SPI Script CS High.vi"("error in (no error)"=w805, "chip select (0)"=w803, "spi script reference in"=w804) -> ("error out"=w801:errorcluster, "spi script reference out"=w800:T1)  [unwired: 7 in]
        n308 = call-poly "NI-845x SPI Script Delay.vi"("error in (no error)"=w801, "delay in microseconds (0)"=u16 1, "spi script reference in"=w800) -> ("error out"=w799:errorcluster, "spi script reference out"=w798:T1)  [unwired: 7 in]
        n309 = call "NI-845x SPI Script CS Low.vi"("error in (no error)"=w799, "chip select (0)"=w803, "spi script reference in"=w798) -> ("error out"=w802:errorcluster)  [unwired: 7 in, 1 out]
        n310 = call <vilib>:"Add State(s) to Queue__jki_lib_state_machine.vi"("State(s) in Front (\"\")"="UI: Display Status >>  [Alert!][WRITE ENABLE Completed][100]" ("State(s) in Front (\"\")"), "State(s) in (\"\")"=w820) -> ("States Out"=w819:string)  [unwired: 13 in]
      }
      frame "NI845x: WRITE 93LC56BT" {
        # "The Microchip 93LC56BT CS idle state is LOW and asserted HIGH\nNote: the NI-8451 can only send 8-bits at a time. Make sure the INIT configures the device properly\nData provided in write data and read back using script read index is organized in big endian format. \nEach sample is stored using the minimum number of bytes required, with the most significant bits padded with 0."
        n311 = Unbundle By Name(w848) -> ("CS/SS Line (0-6)"=w842:u32, "Page Write Delay (ms)"=w838:u8, "SPI Script Reference"=w843:T1, "WRITE"=w844:u8, "EEPROM Program Data"=w845:string[][], "Endianness (WRITE)"=w839:bool, "Invert Data Bits [MSB]"=w837:bool)
        n312 = for {
          tunnel: w846 -> [w884]
          tunnel: w843 -> [w883]
          tunnel: [w897] -> w841
          tunnel: w844 -> [w863]
          tunnel: w842 -> [w885]
          tunnel: [w869] -> w840
          tunnel: w845 -> [w876] mode=indexing
          tunnel: w839 -> [w874]
          tunnel: w838 -> [w870]
          tunnel: w837 -> [w853]
          # "93LC56BT address is only 7 bits!\nstrip the 8th bit!"
          # "Data"
          # "Address"
          # "Tcsl"
          n313 = Index Array(array=w876, index=1) -> (element=w882:string)
          n314 = Index Array(array=w876, index=0) -> (element=w879:string)
          n315 = Number To Boolean Array(number=w863) -> (Boolean array=w867:bool[])
          n316 = call "Hex_String_to_Binary_String.vi"("bitness"=enum16{"8", "16", "32", "64"}."16", "Hexadecimal String"=w879) -> ("number"=w856:u64)  [unwired: 1 in, 2 out]
          n317 = Delete From Array(array=w867, length=5 ("index"), index=0) -> (deleted portion=w860:bool[])  [unwired: 1 out]
          n318 = call "Hex_String_to_Binary_String.vi"("bitness"=enum16{"8", "16", "32", "64"}."16", "Hexadecimal String"=w882) -> ("number"=w875:u64)  [unwired: 1 in, 2 out]
          n319 = To Unsigned Word Integer(number=w875) -> (unsigned 16bit integer=w873:u16)
          n320 = Boolean Array To Number(Boolean array=w860) -> (number=w865:u32)
          n321 = Number To Boolean Array(number=w856) -> (Boolean array=w859:bool[])
          n322 = case shown="True" w874 {
            tunnel: [w901 w904] -> w871
            tunnel: [w900 w905] -> w872
            tunnel: w873 -> [w899 w903]
            tunnel: w853 -> [w898 w902]
            frame True {
              # "Big Endian\nMSB first"
              n323 = call "Split and Invert u16 to two u8.vi"("Invert MSB [F]"=w898, "Input (u16)"=w899) -> ("LSB (u8)"=w901:u8, "MSB (u8)"=w900:u8)  [unwired: 7 in, 1 out]
            }
            frame False {
              # "Little Endian\nLSB first"
              n324 = call "Split and Invert u16 to two u8.vi"("Invert MSB [F]"=w902, "Input (u16)"=w903) -> ("LSB (u8)"=w905:u8, "MSB (u8)"=w904:u8)  [unwired: 7 in, 1 out]
            }
          }
          n325 = To Unsigned Byte Integer(number=w865) -> (unsigned 8bit integer=w862:u8)
          n326 = Delete From Array(array=w859, length=7 ("index"), index=0) -> (deleted portion=w855:bool[])  [unwired: 1 out]
          n327 = Boolean Array To Number(Boolean array=w855) -> (number=w854:u32)
          n328 = To Unsigned Byte Integer(number=w854) -> (unsigned 8bit integer=w861:u8)
          n329 = call "NI-845x SPI Script CS High.vi"("error in (no error)"=w884, "chip select (0)"=w885, "spi script reference in"=w883) -> ("error out"=w888:errorcluster, "spi script reference out"=w889:T1)  [unwired: 7 in]
          n330 = Build Array(w862, w861, w872, w871) -> (w868:u8[])
          n331 = call "NI-845x SPI Script Write Read.vi"("error in (no error)"=w888, "write data"=w868, "spi script reference in"=w889) -> ("error out"=w896:errorcluster, "script read index"=w897:u32, "spi script reference out"=w895:T1)  [unwired: 1 in, 5 out]
          n332 = local write "Data Bytes Written"(w868) -> ()
          n333 = call "NI-845x SPI Script CS Low.vi"("error in (no error)"=w896, "chip select (0)"=w885, "spi script reference in"=w895) -> ("error out"=w894:errorcluster, "spi script reference out"=w893:T1)  [unwired: 7 in]
          n334 = call-poly "NI-845x SPI Script Delay.vi"("error in (no error)"=w894, "delay in microseconds (0)"=u16 1, "spi script reference in"=w893) -> ("error out"=w891:errorcluster, "spi script reference out"=w890:T1)  [unwired: 7 out]
          n335 = call "NI-845x SPI Script CS High.vi"("error in (no error)"=w891, "chip select (0)"=w885, "spi script reference in"=w890) -> ("error out"=w886:errorcluster, "spi script reference out"=w887:T1)  [unwired: 7 in]
          n336 = call-poly "NI-845x SPI Script Delay.vi"("error in (no error)"=w886, "delay in milliseconds (0)"=w870, "spi script reference in"=w887) -> ("error out"=w852:errorcluster, "spi script reference out"=w851:T1)  [unwired: 7 out]
          n337 = call "NI-845x SPI Script CS Low.vi"("error in (no error)"=w852, "chip select (0)"=w885, "spi script reference in"=w851) -> ("error out"=w869:errorcluster)  [unwired: 7 in, 1 out]
        }
        n338 = Bundle By Name(cluster=w848, "script read index"=w841) -> (w847:T10)
        n339 = call <vilib>:"Add State(s) to Queue__jki_lib_state_machine.vi"("State(s) in Front (\"\")"="UI: Display Status >>  [Alert!][WRITE Data Completed][100]" ("State(s) in Front (\"\")"), "State(s) in (\"\")"=w850) -> ("States Out"=w849:string)  [unwired: 13 in]
      }
      frame "NI845x: WRITE 93C86" {
        # "For MC93C86 the MSB is transmitted first (high endian). The Microchip 93C86 CS idle state is LOW and asserted HIGH\nNote: the NI-8452 can send 8-64 bits at a time. Make sure the INIT configures the device properly\nData provided in write data and read back using script read index is organized in big endian format. \nEach sample is stored using the minimum number of bytes required, with the most significant bits padded with 0."
        n340 = Unbundle By Name(w914) -> ("CS/SS Line (0-6)"=w918:u32, "Page Write Delay (ms)"=w916:u8, "SPI Script Reference"=w922:T1, "WRITE"=w919:u8, "Invert Opcode"=w907:bool, "EEPROM Program Data"=w915:string[][], "Endianness (WRITE)"=w910:bool, "Invert Data Bits [MSB]"=w909:bool, "Invert Data Bits [LSB]"=w908:bool)
        n341 = Unbundle By Name(w914) -> ("WRITE Data"=w913:u8[], "Enable Debug?"=w912:bool, "Burst Width"=w911:enum16{"8 bits", "16 bits", "32 bits"})
        n342 = for {
          tunnel: w923 -> [w960]
          tunnel: w922 -> [w961]
          tunnel: [w971] -> w920
          tunnel: w919 -> [w953]
          tunnel: w918 -> [w969]
          tunnel: [w930] -> w917
          tunnel: w916 -> [w966]
          tunnel: w915 -> [w976] mode=indexing
          tunnel: w912 -> [w952]
          tunnel: w913 -> [w951]
          tunnel: w911 -> [_]
          tunnel: w910 -> [w945]
          tunnel: w909 -> [w941]
          tunnel: w908 -> [w938]
          tunnel: w907 -> [w926]
          w929 = FALSE ("Invert [F]")
          w942 = 10 ("index")
          # "1. 93C86 has 10-bit address field 2 MSB bits must be merged\ninto the LSB of the opcode field\n2. NI-845x transmits MSb (bit) first so rotate the bits??\n3. ST MC93C86 is big-endian arrangement (MSB byte stored at higher-order byte of word and stored at lowest address."
          # "Data"
          # "Address"
          n343 = Number To Boolean Array(number=w953) -> (Boolean array=w964:bool[])
          n344 = Index Array(array=w976, index=0) -> (element=w978:string)
          n345 = Index Array(array=w976, index=1) -> (element=w974:string)
          n346 = Delete From Array(array=w964, length=5 ("index"), index=0) -> (deleted portion=w928:bool[])  [unwired: 1 out]
          n347 = call "Hex_String_to_Binary_String.vi"("bitness"=enum16{"8", "16", "32", "64"}."16", "Hexadecimal String"=w974) -> ("number"=w973:u64)  [unwired: 1 in, 2 out]
          n348 = case shown="True" w926 {
            tunnel: w928 -> [w981 w983]
            tunnel: [w981 w982] -> w927
            frame False {
            }
            frame True {
              n349 = Reverse 1D Array(array=w983) -> (reversed array=w982:bool[])
            }
          }
          n350 = call "Hex_String_to_Binary_String.vi"("bitness"=enum16{"8", "16", "32", "64"}."16", "Hexadecimal String"=w978) -> ("number"=w965:u64)  [unwired: 1 in, 2 out]
          n351 = To Unsigned Word Integer(number=w973) -> (unsigned 16bit integer=w944:u16)
          n352 = To Unsigned Word Integer(number=w965) -> (unsigned 16bit integer=w954:u16)
          n353 = Number To Boolean Array(number=w954) -> (Boolean array=w958:bool[])
          n354 = case shown="False" w945 {
            tunnel: [w988 w992] -> w947
            tunnel: [w987 w993] -> w946
            tunnel: w944 -> [w986 w991]
            tunnel: w941 -> [w985 w990]
            tunnel: w938 -> [w984 w989]
            frame True {
              # "Big Endian\nMSB first"
              n355 = call "Split and Invert u16 to two u8.vi"("Invert LSB [F]"=w984, "Invert MSB [F]"=w985, "Input (u16)"=w986) -> ("LSB (u8)"=w988:u8, "MSB (u8)"=w987:u8)  [unwired: 6 in, 1 out]
            }
            frame False {
              # "Little Endian\nLSB first"
              n356 = call "Split and Invert u16 to two u8.vi"("Invert LSB [F]"=w989, "Invert MSB [F]"=w990, "Input (u16)"=w991) -> ("LSB (u8)"=w993:u8, "MSB (u8)"=w992:u8)  [unwired: 6 in, 1 out]
            }
          }
          n357 = Delete From Array(array=w958, length=w942, index=0) -> (deleted portion=w943:bool[])  [unwired: 1 out]
          n358 = Insert Into Array(array=w943, index=w942, new element=w927) -> (w962:bool[])
          n359 = Boolean Array To Number(Boolean array=w962) -> (number=w949:u32)
          n360 = call "Split and Invert u16 to two u8.vi"("Invert LSB [F]"=w929, "Invert MSB [F]"=w929, "Input (u16)"=w949) -> ("LSB (u8)"=w939:u8, "MSB (u8)"=w940:u8)  [unwired: 6 in, 1 out]
          n361 = call "NI-845x SPI Script CS High.vi"("error in (no error)"=w960, "chip select (0)"=w969, "spi script reference in"=w961) -> ("error out"=w956:errorcluster, "spi script reference out"=w955:T1)  [unwired: 7 in]
          n362 = Build Array(w940, w939, w946, w947) -> (w950:u8[])
          n363 = case shown="False" w952 {
            tunnel: w951 -> [_ w995]
            tunnel: w950 -> [w994 _]
            tunnel: [w994 w995] -> w948
            frame False {
            }
            frame True {
            }
          }
          n364 = call "NI-845x SPI Script Write Read.vi"("error in (no error)"=w956, "write data"=w948, "spi script reference in"=w955) -> ("error out"=w972:errorcluster, "script read index"=w971:u32, "spi script reference out"=w970:T1)  [unwired: 1 in, 5 out]
          n365 = local write "Data Bytes Written"(w948) -> ()
          n366 = call "NI-845x SPI Script CS Low.vi"("error in (no error)"=w972, "chip select (0)"=w969, "spi script reference in"=w970) -> ("error out"=w937:errorcluster, "spi script reference out"=w936:T1)  [unwired: 7 in]
          n367 = call-poly "NI-845x SPI Script Delay.vi"("error in (no error)"=w937, "delay in microseconds (0)"=u16 1, "spi script reference in"=w936) -> ("error out"=w934:errorcluster, "spi script reference out"=w933:T1)  [unwired: 7 in]
          n368 = call "NI-845x SPI Script CS High.vi"("error in (no error)"=w934, "chip select (0)"=w969, "spi script reference in"=w933) -> ("error out"=w968:errorcluster, "spi script reference out"=w967:T1)  [unwired: 7 in]
          n369 = call-poly "NI-845x SPI Script Delay.vi"("error in (no error)"=w968, "delay in milliseconds (0)"=w966, "spi script reference in"=w967) -> ("error out"=w932:errorcluster, "spi script reference out"=w931:T1)  [unwired: 7 in]
          n370 = call "NI-845x SPI Script CS Low.vi"("error in (no error)"=w932, "spi script reference in"=w931) -> ("error out"=w930:errorcluster)  [unwired: 8 in, 1 out]
        }
        n371 = Bundle By Name(cluster=w914, "script read index"=w920) -> (w921:T10)
        n372 = call <vilib>:"Add State(s) to Queue__jki_lib_state_machine.vi"("State(s) in Front (\"\")"="UI: Display Status >>  [Alert!][WRITE Data Completed][100]" ("State(s) in Front (\"\")"), "State(s) in (\"\")"=w925) -> ("States Out"=w924:string)  [unwired: 13 in]
      }
      frame "NI845x: WRITE 93LC86 [8452]" {
        # "For 93LC86 the MSB is transmitted first (high endian). The Microchip 93LC86 CS idle state is LOW and asserted HIGH\nNote: the NI-8452 can send 8-64 bits at a time. Make sure the INIT configures the device properly\nData provided in write data and read back using script read index is organized in big endian format. \nEach sample is stored using the minimum number of bytes required, with the most significant bits padded with 0."
        n373 = Unbundle By Name(w1004) -> ("CS/SS Line (0-6)"=w1008:u32, "Page Write Delay (ms)"=w1006:u8, "SPI Script Reference"=w1012:T1, "WRITE"=w1009:u8, "Invert Opcode"=w997:bool, "EEPROM Program Data"=w1005:string[][], "Endianness (WRITE)"=w1000:bool, "Invert Data Bits [MSB]"=w999:bool, "Invert Data Bits [LSB]"=w998:bool)
        n374 = Unbundle By Name(w1004) -> ("WRITE Data"=w1003:u8[], "Enable Debug?"=w1002:bool, "Burst Width"=w1001:enum16{"8 bits", "16 bits", "32 bits"})
        n375 = for {
          tunnel: w1013 -> [w1031]
          tunnel: w1012 -> [w1030]
          tunnel: [w1061] -> w1010
          tunnel: w1009 -> [w1041]
          tunnel: w1008 -> [w1059]
          tunnel: [w1021] -> w1007
          tunnel: w1006 -> [w1056]
          tunnel: w1005 -> [w1066] mode=indexing
          tunnel: w1002 -> [w1035]
          tunnel: w1003 -> [w1040]
          tunnel: w1001 -> [_]
          tunnel: w1000 -> [w1028]
          tunnel: w999 -> [w1029]
          tunnel: w998 -> [w1020]
          tunnel: w997 -> [w1016]
          w1019 = FALSE ("Invert LSB [F]")
          w1034 = 10 ("index")
          # "1. 93C86 has 10-bit address field 2 MSB bits must be merged\ninto the LSB of the opcode field\n2. NI-845x transmits MSb (bit) first so rotate the bits??\n3. ST MC93C86 is big-endian arrangement (MSB byte stored at higher-order byte of word and stored at lowest address."
          # "// 93LC series EEPROMs do need the CS low\nbetween last CLK rising edge to next CLK\nrising edge. Just toggle the CS to assert"
          # "Data"
          # "Address"
          n376 = Number To Boolean Array(number=w1041) -> (Boolean array=w1054:bool[])
          n377 = Index Array(array=w1066, index=0) -> (element=w1068:string)
          n378 = Index Array(array=w1066, index=1) -> (element=w1064:string)
          n379 = Delete From Array(array=w1054, length=5 ("index"), index=0) -> (deleted portion=w1018:bool[])  [unwired: 1 out]
          n380 = call "Hex_String_to_Binary_String.vi"("bitness"=enum16{"8", "16", "32", "64"}."16", "Hexadecimal String"=w1068) -> ("number"=w1055:u64)  [unwired: 1 in, 2 out]
          n381 = case shown="True" w1016 {
            tunnel: w1018 -> [w1071 w1073]
            tunnel: [w1071 w1072] -> w1017
            frame False {
            }
            frame True {
              n382 = Reverse 1D Array(array=w1073) -> (reversed array=w1072:bool[])
            }
          }
          n383 = call "Hex_String_to_Binary_String.vi"("bitness"=enum16{"8", "16", "32", "64"}."16", "Hexadecimal String"=w1064) -> ("number"=w1063:u64)  [unwired: 1 in, 2 out]
          n384 = To Unsigned Word Integer(number=w1055) -> (unsigned 16bit integer=w1042:u16)
          n385 = To Unsigned Word Integer(number=w1063) -> (unsigned 16bit integer=w1027:u16)
          n386 = Number To Boolean Array(number=w1042) -> (Boolean array=w1046:bool[])
          n387 = case shown="True" w1028 {
            tunnel: [w1078 w1082] -> w1026
            tunnel: [w1077 w1083] -> w1025
            tunnel: w1027 -> [w1076 w1081]
            tunnel: w1029 -> [w1075 w1080]
            tunnel: w1020 -> [w1074 w1079]
            frame True {
              # "Big Endian\nMSB first"
              n388 = call "Split and Invert u16 to two u8.vi"("Invert LSB [F]"=w1074, "Invert MSB [F]"=w1075, "Input (u16)"=w1076) -> ("LSB (u8)"=w1078:u8, "MSB (u8)"=w1077:u8)  [unwired: 6 in, 1 out]
            }
            frame False {
              # "Little Endian\nLSB first"
              n389 = call "Split and Invert u16 to two u8.vi"("Invert LSB [F]"=w1079, "Invert MSB [F]"=w1080, "Input (u16)"=w1081) -> ("LSB (u8)"=w1083:u8, "MSB (u8)"=w1082:u8)  [unwired: 6 in, 1 out]
            }
          }
          n390 = Delete From Array(array=w1046, length=w1034, index=0) -> (deleted portion=w1024:bool[])  [unwired: 1 out]
          n391 = Insert Into Array(array=w1024, index=w1034, new element=w1017) -> (w1048:bool[])
          n392 = Boolean Array To Number(Boolean array=w1048) -> (number=w1038:u32)
          n393 = call "Split and Invert u16 to two u8.vi"("Invert LSB [F]"=w1019, "Invert MSB [F]"=w1019, "Input (u16)"=w1038) -> ("LSB (u8)"=w1032:u8, "MSB (u8)"=w1033:u8)  [unwired: 6 in, 1 out]
          n394 = call "NI-845x SPI Script CS High.vi"("error in (no error)"=w1031, "chip select (0)"=w1059, "spi script reference in"=w1030) -> ("error out"=w1044:errorcluster, "spi script reference out"=w1043:T1)  [unwired: 7 in]
          n395 = Build Array(w1033, w1032, w1025, w1026) -> (w1039:u8[])
          n396 = case shown="True" w1035 {
            tunnel: w1040 -> [_ w1085]
            tunnel: w1039 -> [w1084 _]
            tunnel: [w1084 w1085] -> w1037
            frame False {
            }
            frame True {
            }
          }
          n397 = call "NI-845x SPI Script Write Read.vi"("error in (no error)"=w1044, "write data"=w1037, "spi script reference in"=w1043) -> ("error out"=w1062:errorcluster, "script read index"=w1061:u32, "spi script reference out"=w1060:T1)  [unwired: 1 in, 5 out]
          n398 = local write "Data Bytes Written"(w1037) -> ()
          n399 = call "NI-845x SPI Script CS Low.vi"("error in (no error)"=w1062, "chip select (0)"=w1059, "spi script reference in"=w1060) -> ("error out"=w1052:errorcluster, "spi script reference out"=w1050:T1)  [unwired: 7 in]
          n400 = call-poly "NI-845x SPI Script Delay.vi"("error in (no error)"=w1052, "delay in microseconds (0)"=u16 1, "spi script reference in"=w1050) -> ("error out"=w1051:errorcluster, "spi script reference out"=w1049:T1)  [unwired: 7 in]
          n401 = call "NI-845x SPI Script CS High.vi"("error in (no error)"=w1051, "chip select (0)"=w1059, "spi script reference in"=w1049) -> ("error out"=w1058:errorcluster, "spi script reference out"=w1057:T1)  [unwired: 7 in]
          n402 = call-poly "NI-845x SPI Script Delay.vi"("error in (no error)"=w1058, "delay in milliseconds (0)"=w1056, "spi script reference in"=w1057) -> ("error out"=w1023:errorcluster, "spi script reference out"=w1022:T1)  [unwired: 7 in]
          n403 = call "NI-845x SPI Script CS Low.vi"("error in (no error)"=w1023, "spi script reference in"=w1022) -> ("error out"=w1021:errorcluster)  [unwired: 8 in, 1 out]
        }
        n404 = Bundle By Name(cluster=w1004, "script read index"=w1010) -> (w1011:T10)
        n405 = call <vilib>:"Add State(s) to Queue__jki_lib_state_machine.vi"("State(s) in Front (\"\")"="UI: Display Status >>  [Alert!][WRITE Data Completed][100]" ("State(s) in Front (\"\")"), "State(s) in (\"\")"=w1015) -> ("States Out"=w1014:string)  [unwired: 13 in]
      }
      frame "NI845x: WRITE 93LC86 [8451]" {
        # "For MC93C86 the MSB is transmitted first (high endian). The Microchip 93C86 CS idle state is LOW and asserted HIGH\nNote: the NI-8451 can only send 8 bits at a time. Make sure the INIT configures the device properly\nData provided in write data and read back using script read index is organized in big endian format. \nEach sample is stored using the minimum number of bytes required, with the most significant bits padded with 0."
        n406 = Unbundle By Name(w1093) -> ("Page Write Delay (ms)"=w1088:u8, "CS/SS Line (0-6)"=w1096:u32, "SPI Script Reference"=w1100:T1, "WRITE"=w1097:u8, "EEPROM Program Data"=w1094:string[][], "Endianness (WRITE)"=w1090:bool, "Invert Data Bits [MSB]"=w1089:bool, "Invert Data Bits [LSB]"=w1087:bool)
        n407 = Unbundle By Name(w1093) -> ("WRITE Data"=w1092:u8[], "Enable Debug?"=w1091:bool)
        n408 = for {
          tunnel: w1101 -> [w1135]
          tunnel: w1100 -> [w1136]
          tunnel: [w1150] -> w1098
          tunnel: w1097 -> [w1129]
          tunnel: w1096 -> [w1148]
          tunnel: [w1111] -> w1095
          tunnel: w1088 -> [w1145]
          tunnel: w1094 -> [w1155] mode=indexing
          tunnel: w1091 -> [w1123]
          tunnel: w1092 -> [w1128]
          tunnel: w1090 -> [w1117]
          tunnel: w1089 -> [w1118]
          tunnel: w1087 -> [w1109]
          w1106 = 10 ("index")
          # "1. 93C86 has 10-bit address field 2 MSB bits must be merged\ninto the LSB of the opcode field\n2. NI-845x transmits MSb (bit) first so rotate the bits??\n3. ST MC93C86 is big-endian arrangement (MSB byte stored at higher-order byte of word and stored at lowest address."
          # "// 93LC series EEPROMs do need the CS low\nbetween last CLK rising edge to next CLK\nrising edge. Just toggle the CS to assert"
          # "Data"
          # "Address"
          n409 = Number To Boolean Array(number=w1129) -> (Boolean array=w1143:bool[])
          n410 = Index Array(array=w1155, index=0) -> (element=w1157:string)
          n411 = Index Array(array=w1155, index=1) -> (element=w1153:string)
          n412 = Delete From Array(array=w1143, length=5 ("index"), index=0) -> (deleted portion=w1122:bool[])  [unwired: 1 out]
          n413 = call "Hex_String_to_Binary_String.vi"("bitness"=enum16{"8", "16", "32", "64"}."16", "Hexadecimal String"=w1157) -> ("number"=w1144:u64)  [unwired: 1 in, 2 out]
          n414 = call "Hex_String_to_Binary_String.vi"("bitness"=enum16{"8", "16", "32", "64"}."16", "Hexadecimal String"=w1153) -> ("number"=w1152:u64)  [unwired: 1 in, 2 out]
          n415 = To Unsigned Word Integer(number=w1144) -> (unsigned 16bit integer=w1130:u16)
          n416 = To Unsigned Word Integer(number=w1152) -> (unsigned 16bit integer=w1116:u16)
          n417 = Number To Boolean Array(number=w1130) -> (Boolean array=w1133:bool[])
          n418 = case shown="True" w1117 {
            tunnel: [w1164 w1168] -> w1115
            tunnel: [w1163 w1169] -> w1114
            tunnel: w1116 -> [w1162 w1167]
            tunnel: w1118 -> [w1161 w1166]
            tunnel: w1109 -> [w1160 w1165]
            frame True {
              # "Big Endian\nMSB first"
              n419 = call "Split and Invert u16 to two u8.vi"("Invert LSB [F]"=w1160, "Invert MSB [F]"=w1161, "Input (u16)"=w1162) -> ("LSB (u8)"=w1164:u8, "MSB (u8)"=w1163:u8)  [unwired: 6 in, 1 out]
            }
            frame False {
              # "Little Endian\nLSB first"
              n420 = call "Split and Invert u16 to two u8.vi"("Invert LSB [F]"=w1165, "Invert MSB [F]"=w1166, "Input (u16)"=w1167) -> ("LSB (u8)"=w1169:u8, "MSB (u8)"=w1168:u8)  [unwired: 6 in, 1 out]
            }
          }
          n421 = Delete From Array(array=w1133, length=w1106, index=0) -> (deleted portion=w1121:bool[])  [unwired: 1 out]
          n422 = Reverse 1D Array(array=w1121) -> (reversed array=w1108:bool[])
          n423 = Insert Into Array(array=w1108, index=w1106, new element=w1122) -> (w1137:bool[])
          n424 = Boolean Array To Number(Boolean array=w1137) -> (number=w1126:u32)
          n425 = To Unsigned Word Integer(number=w1126) -> (unsigned 16bit integer=w1104:u16)
          n426 = call "Split and Invert u16 to two u8.vi"("Invert LSB [F]"=TRUE, "Invert MSB [F]"=FALSE, "Input (u16)"=w1104) -> ("LSB (u8)"=w1119:u8, "MSB (u8)"=w1120:u8)  [unwired: 6 in, 1 out]
          n427 = call "NI-845x SPI Script CS High.vi"("error in (no error)"=w1135, "chip select (0)"=w1148, "spi script reference in"=w1136) -> ("error out"=w1132:errorcluster, "spi script reference out"=w1131:T1)  [unwired: 7 in]
          n428 = Build Array(w1120, w1119, w1114, w1115) -> (w1127:u8[])
          n429 = case shown="False" w1123 {
            tunnel: w1128 -> [_ w1171]
            tunnel: w1127 -> [w1170 _]
            tunnel: [w1170 w1171] -> w1125
            frame False {
            }
            frame True {
            }
          }
          n430 = call "NI-845x SPI Script Write Read.vi"("error in (no error)"=w1132, "write data"=w1125, "spi script reference in"=w1131) -> ("error out"=w1151:errorcluster, "script read index"=w1150:u32, "spi script reference out"=w1149:T1)  [unwired: 1 in, 5 out]
          n431 = local write "Data Bytes Written"(w1125) -> ()
          n432 = call "NI-845x SPI Script CS Low.vi"("error in (no error)"=w1151, "chip select (0)"=w1148, "spi script reference in"=w1149) -> ("error out"=w1141:errorcluster, "spi script reference out"=w1139:T1)  [unwired: 7 in]
          n433 = call-poly "NI-845x SPI Script Delay.vi"("error in (no error)"=w1141, "delay in microseconds (0)"=u16 1, "spi script reference in"=w1139) -> ("error out"=w1140:errorcluster, "spi script reference out"=w1138:T1)  [unwired: 7 in]
          n434 = call "NI-845x SPI Script CS High.vi"("error in (no error)"=w1140, "chip select (0)"=w1148, "spi script reference in"=w1138) -> ("error out"=w1147:errorcluster, "spi script reference out"=w1146:T1)  [unwired: 7 in]
          n435 = call-poly "NI-845x SPI Script Delay.vi"("error in (no error)"=w1147, "delay in milliseconds (0)"=w1145, "spi script reference in"=w1146) -> ("error out"=w1113:errorcluster, "spi script reference out"=w1112:T1)  [unwired: 7 in]
          n436 = call "NI-845x SPI Script CS Low.vi"("error in (no error)"=w1113, "spi script reference in"=w1112) -> ("error out"=w1111:errorcluster)  [unwired: 8 in, 1 out]
        }
        n437 = Bundle By Name(cluster=w1093, "script read index"=w1098) -> (w1099:T10)
        n438 = call <vilib>:"Add State(s) to Queue__jki_lib_state_machine.vi"("State(s) in Front (\"\")"="UI: Display Status >>  [Alert!][WRITE Data Completed][100]" ("State(s) in Front (\"\")"), "State(s) in (\"\")"=w1103) -> ("States Out"=w1102:string)  [unwired: 13 in]
      }
      frame "NI845x: EWDS" {
        w1199 = u8 0
        # "1. Send SB & EWDS Opcode\n2. A dummy address byte\n3. A dummy data byte"
        n439 = Unbundle By Name(w1195) -> ("EWDS"=w1193:u8, "EEPROM Device Type"=w1185:T6, "SPI Script Reference"=w1188:T1, "CS/SS Line (0-6)"=w1173:u32, "Page Write Delay (ms)"=w1174:u8)
        n440 = case shown="\"ST-M93C86\"" w1185 {
          tunnel: w1190 -> [w1207 w1208]
          tunnel: [w1206 w1208] -> w1189
          tunnel: w1188 -> [w1205 w1209]
          tunnel: [w1204 w1209] -> w1187
          frame "ST-M93C86" {
            w1202 = 0 items=["0 (First Edge)", "1 (Second Edge)"] ("clock phase (0)")
            w1203 = 0 items=["0 (Idle Low)", "1 (Idle High)"] ("clock polarity (0)")
            n441 = call "NI-845x SPI Script Clock Polarity Phase.vi"("error in (no error)"=w1207, "clock phase (0)"=w1202, "clock polarity (0)"=w1203, "spi script reference in"=w1205) -> ("error out"=w1206:errorcluster, "spi script reference out"=w1204:T1)  [unwired: 6 in]
          }
          frame "Generic EEPROM", Default {
          }
        }
        n442 = call "NI-845x SPI Script CS Low.vi"("error in (no error)"=w1189, "chip select (0)"=w1173, "spi script reference in"=w1187) -> ("spi script reference out"=w1192:T1)  [unwired: 7 in, 1 out]
        n443 = To Unsigned Byte Integer(number=w1193) -> (unsigned 8bit integer=w1186:u8)
        n444 = call "NI-845x SPI Script CS High.vi"("error in (no error)"=w1189, "chip select (0)"=w1173, "spi script reference in"=w1192) -> ("error out"=w1191:errorcluster, "spi script reference out"=w1194:T1)  [unwired: 7 in]
        n445 = Build Array(w1186, w1199, w1199) -> (w1198:u8[])
        n446 = call "NI-845x SPI Script Write Read.vi"("error in (no error)"=w1191, "write data"=w1198, "spi script reference in"=w1194) -> ("error out"=w1196:errorcluster, "spi script reference out"=w1197:T1)  [unwired: 1 in, 6 out]
        n447 = call "NI-845x SPI Script CS Low.vi"("error in (no error)"=w1196, "chip select (0)"=w1173, "spi script reference in"=w1197) -> ("error out"=w1184:errorcluster, "spi script reference out"=w1183:T1)  [unwired: 7 in]
        n448 = call-poly "NI-845x SPI Script Delay.vi"("error in (no error)"=w1184, "delay in microseconds (0)"=u16 1, "spi script reference in"=w1183) -> ("error out"=w1181:errorcluster, "spi script reference out"=w1180:T1)  [unwired: 7 in]
        n449 = call "NI-845x SPI Script CS High.vi"("error in (no error)"=w1181, "chip select (0)"=w1173, "spi script reference in"=w1180) -> ("error out"=w1179:errorcluster, "spi script reference out"=w1178:T1)  [unwired: 7 in]
        n450 = call-poly "NI-845x SPI Script Delay.vi"("error in (no error)"=w1179, "delay in milliseconds (0)"=w1174, "spi script reference in"=w1178) -> ("error out"=w1177:errorcluster, "spi script reference out"=w1176:T1)  [unwired: 7 in]
        n451 = call "NI-845x SPI Script CS Low.vi"("error in (no error)"=w1177, "chip select (0)"=w1173, "spi script reference in"=w1176) -> ("error out"=w1175:errorcluster)  [unwired: 7 in, 1 out]
        n452 = call <vilib>:"Add State(s) to Queue__jki_lib_state_machine.vi"("State(s) in Front (\"\")"="UI: Display Status >>  [Alert!][WRITE/ERASE DISABLE Completed][100]" ("State(s) in Front (\"\")"), "State(s) in (\"\")"=w1201) -> ("States Out"=w1200:string)  [unwired: 13 in]
      }
      frame "NI845x: READ ALL" {
        # "For Microchip 93C86 the MSB is transmitted first (high endian)\nThe Microchip 93C86 CS idle state is LOW and asserted HIGH\nThis node needs the NI8452 model. NI845x only supports 8 bits\n*** READ ALL starts reading from address 0x0000 to 0xXXXX ***"
        n453 = Unbundle By Name(w1234) -> ("CS/SS Line (0-6)"=w1214:u32, "Page Write Delay (ms)"=w1218:u8, "SPI Script Reference"=w1229:T1, "EEPROM Device Type"=w1212:T6, "Invert Opcode"=w1211:bool, "READ"=w1233:u8, "Invert Address"=w1210:bool)
        n454 = case shown="\"ST-M93C86\"" w1212 {
          tunnel: w1233 -> [w1243 w1256 w1278 w1285 w1300]
          tunnel: [w1242 w1267 w1277 w1284 w1309] -> w1226
          tunnel: w1211 -> [_ w1248 _ _ w1290]
          tunnel: w1210 -> [_ w1247 _ _ w1289]
          frame "Generic EEPROM", Default {
            n455 = Initialize Array(u8 255 ("element"), 255 ("element")) -> (w1245:u8[])
            n456 = To Unsigned Byte Integer(number=w1243) -> (unsigned 8bit integer=w1244:u8)
            n457 = Build Array (concatenate)(w1244, u8 0 ("t"), w1245) -> (w1242:u8[])
          }
          frame "ST-M93C86" {
            w1249 = FALSE ("Invert MSB [F]")
            w1255 = 0 ("index")
            w1258 = 10 ("index")
            # "The Microchip/ST-M93C86 is organized as:\n1024 x16 bits,  *ORG = 1\n* here we read 2x the # mem array (0x800 + 2)\nsince the array is loaded from two 8-bits per element"
            n458 = Number To Boolean Array(number=w1256) -> (Boolean array=w1262:bool[])
            n459 = Number To Boolean Array(number=w1255) -> (Boolean array=w1261:bool[])
            n460 = Delete From Array(array=w1262, length=6 ("index"), index=0) -> (deleted portion=w1259:bool[])  [unwired: 1 out]
            n461 = Delete From Array(array=w1261, length=w1258, index=w1255) -> (deleted portion=w1260:bool[])  [unwired: 1 out]
            n462 = case shown="True" w1248 {
              tunnel: w1259 -> [w1272 w1274]
              tunnel: [w1272 w1273] -> w1250
              frame False {
              }
              frame True {
                n463 = Reverse 1D Array(array=w1274) -> (reversed array=w1273:bool[])
              }
            }
            n464 = case shown="True" w1247 {
              tunnel: w1260 -> [w1269 w1271]
              tunnel: [w1269 w1270] -> w1257
              frame False {
              }
              frame True {
                n465 = Reverse 1D Array(array=w1271) -> (reversed array=w1270:bool[])
              }
            }
            n466 = Insert Into Array(array=w1257, index=w1258, new element=w1250) -> (w1251:bool[])
            n467 = Boolean Array To Number(Boolean array=w1251) -> (number=w1254:u32)
            n468 = Initialize Array(u8 255 ("t"), 2050 ("t")) -> (w1268:u8[])
            n469 = call "Split and Invert u16 to two u8.vi"("Invert LSB [F]"=w1249, "Invert MSB [F]"=w1249, "Input (u16)"=w1254) -> ("LSB (u8)"=w1252:u8, "MSB (u8)"=w1253:u8)  [unwired: 6 in, 1 out]
            n470 = Build Array (concatenate)(w1253, w1252, w1268) -> (w1267:u8[])
          }
          frame "Microchip LC56BT" {
            # "* Dummy address"
            # "The LC56BT is organized as:\n128x16 bits *ORG = 1\n* here we read 2x the # mem array (0xFF + 1)\nsince the array is loaded 8 bits per element"
            n471 = Initialize Array(u8 255 ("element"), 258 ("t")) -> (w1281:u8[])
            n472 = To Unsigned Byte Integer(number=w1278) -> (unsigned 8bit integer=w1279:u8)
            n473 = Build Array (concatenate)(w1279, u8 0 ("t"), w1281) -> (w1277:u8[])
          }
          frame "Microchip 93LC86C [8451]" {
            # "* Dummy address"
            # "The Microchip 93C86 is organized as:\n1024 x16 bits,  *ORG = 1\n* here we read 2x the # mem array (0x800 + 2)\nsince the array is loaded from two 8-bits per element"
            n474 = Initialize Array(u8 255 ("element"), 2050 ("t")) -> (w1288:u8[])
            n475 = To Unsigned Byte Integer(number=w1285) -> (unsigned 8bit integer=w1286:u8)
            n476 = Build Array (concatenate)(w1286, u8 0 ("t"), w1288) -> (w1284:u8[])
          }
          frame "Microchip 93LC86C [8452]" {
            w1294 = FALSE ("Invert MSB [F]")
            w1299 = 0 ("index")
            w1302 = 10 ("index")
            # "invert address bit order"
            # "invert opcode bit order"
            # "The Microchip 93C86 is organized as:\n1024 x16 bits,  *ORG = 1\n* here we read 2x the # mem array (0x800 + 2)\nsince the array is loaded from two 8-bits per element"
            n477 = Number To Boolean Array(number=w1300) -> (Boolean array=w1304:bool[])
            n478 = Number To Boolean Array(number=w1299) -> (Boolean array=w1303:bool[])
            n479 = Delete From Array(array=w1304, length=6 ("index"), index=0) -> (deleted portion=w1292:bool[])  [unwired: 1 out]
            n480 = Delete From Array(array=w1303, length=w1302, index=w1299) -> (deleted portion=w1301:bool[])  [unwired: 1 out]
            n481 = case shown="True" w1290 {
              tunnel: w1292 -> [w1314 w1316]
              tunnel: [w1314 w1315] -> w1291
              frame False {
              }
              frame True {
                n482 = Reverse 1D Array(array=w1316) -> (reversed array=w1315:bool[])
              }
            }
            n483 = case shown="True" w1289 {
              tunnel: w1301 -> [w1311 w1313]
              tunnel: [w1311 w1312] -> w1293
              frame False {
              }
              frame True {
                n484 = Reverse 1D Array(array=w1313) -> (reversed array=w1312:bool[])
              }
            }
            n485 = Insert Into Array(array=w1293, index=w1302, new element=w1291) -> (w1295:bool[])
            n486 = Initialize Array(u8 255 ("t"), 2050 ("t")) -> (w1310:u8[])
            n487 = Boolean Array To Number(Boolean array=w1295) -> (number=w1298:u32)
            n488 = call "Split and Invert u16 to two u8.vi"("Invert LSB [F]"=w1294, "Invert MSB [F]"=w1294, "Input (u16)"=w1298) -> ("LSB (u8)"=w1296:u8, "MSB (u8)"=w1297:u8)  [unwired: 6 in, 1 out]
            n489 = Build Array (concatenate)(w1297, w1296, w1310) -> (w1309:u8[])
          }
        }
        n490 = call "NI-845x SPI Script CS High.vi"("error in (no error)"=w1230, "chip select (0)"=w1214, "spi script reference in"=w1229) -> ("error out"=w1228:errorcluster, "spi script reference out"=w1235:T1)  [unwired: 7 in]
        n491 = call "NI-845x SPI Script Write Read.vi"("error in (no error)"=w1228, "write data"=w1226, "spi script reference in"=w1235) -> ("error out"=w1237:errorcluster, "script read index"=w1231:u32, "spi script reference out"=w1236:T1)  [unwired: 1 in, 5 out]
        n492 = local write "Data Bytes Written"(w1226) -> ()
        n493 = call "NI-845x SPI Script CS Low.vi"("error in (no error)"=w1237, "chip select (0)"=w1214, "spi script reference in"=w1236) -> ("error out"=w1225:errorcluster, "spi script reference out"=w1224:T1)  [unwired: 7 in]
        n494 = Bundle By Name(cluster=w1234, "script read index"=w1231, "Read ALL"=TRUE) -> (w1232:T10)
        n495 = call-poly "NI-845x SPI Script Delay.vi"("error in (no error)"=w1225, "delay in microseconds (0)"=u16 1, "spi script reference in"=w1224) -> ("error out"=w1223:errorcluster, "spi script reference out"=w1222:T1)  [unwired: 7 in]
        n496 = call "NI-845x SPI Script CS High.vi"("error in (no error)"=w1223, "chip select (0)"=w1214, "spi script reference in"=w1222) -> ("error out"=w1220:errorcluster, "spi script reference out"=w1219:T1)  [unwired: 7 in]
        n497 = call-poly "NI-845x SPI Script Delay.vi"("error in (no error)"=w1220, "delay in milliseconds (0)"=w1218, "spi script reference in"=w1219) -> ("error out"=w1217:errorcluster, "spi script reference out"=w1216:T1)  [unwired: 7 in]
        n498 = call "NI-845x SPI Script CS Low.vi"("error in (no error)"=w1217, "chip select (0)"=w1214, "spi script reference in"=w1216) -> ("error out"=w1215:errorcluster)  [unwired: 7 in, 1 out]
        n499 = call <vilib>:"Add State(s) to Queue__jki_lib_state_machine.vi"("State(s) in Front (\"\")"="UI: Display Status >>  [Alert!][READ Data Completed][100]" ("State(s) in Front (\"\")"), "State(s) in (\"\")"=w1239) -> ("States Out"=w1238:string)  [unwired: 13 in]
      }
      frame "NI845x: READ" {
        # "FYI: The READ opcode works for all Microchip\n93C or 93LC EEPROM series with the only\ndifference of ORG data sizes. All return an\ninitial dummy bit \"0\" after the last address\nbit (LSb) is transferred."
        # "For Microchip 93C86 the MSB is transmitted first (high endian)\nThe Microchip 93C86 CS idle state is LOW and asserted HIGH\nThis node needs the NI8452 model. NI845x only supports 8 bits\n*** READ reads one  EEPROM address (8 or 16-bits) ***"
        n500 = Unbundle By Name(w1343) -> ("CS/SS Line (0-6)"=w1331:u32, "SPI Script Reference"=w1335:T1, "Invert Opcode"=w1318:bool, "READ"=w1342:u8, "Address"=w1339:u16, "EEPROM Device Type"=w1330:T6, "Invert Address"=w1317:bool, "Invert Data Bits [MSB]"=w1324:bool)  [unwired: 1 out]
        n501 = case shown="\"Microchip 93LC86C [8452]\"" w1330 {
          tunnel: w1342 -> [w1354 w1366 w1400 w1422 w1448]
          tunnel: [w1352 w1364 w1404 w1427 w1453] -> w1325
          tunnel: w1339 -> [w1353 w1365 w1395 w1411 w1437]
          tunnel: w1324 -> [_ _ _ _ _]
          tunnel: w1318 -> [_ w1358 _ w1406 _]
          tunnel: w1317 -> [_ w1357 _ w1405 _]
          frame "Generic EEPROM", Default {
            n502 = To Unsigned Byte Integer(number=w1354) -> (unsigned 8bit integer=w1355:u8)
            n503 = To Unsigned Byte Integer(number=w1353) -> (unsigned 8bit integer=w1356:u8)
            n504 = Initialize Array(u8 255 ("element"), 2 ("dimension size")) -> (w1350:u8[])
            n505 = Build Array (concatenate)(w1355, w1356, w1350) -> (w1352:u8[])
          }
          frame "ST-M93C86" {
            w1371 = 10 ("index")
            # "MSb transmitted first\nby NI-8452"
            # "93C86 has 10-bit address field\n2 MSB bits must be merged\ninto the LSB of the opcode field"
            n506 = Number To Boolean Array(number=w1366) -> (Boolean array=w1377:bool[])
            n507 = Number To Boolean Array(number=w1365) -> (Boolean array=w1375:bool[])
            n508 = Delete From Array(array=w1377, length=6 ("index"), index=0) -> (deleted portion=w1361:bool[])  [unwired: 1 out]
            n509 = Delete From Array(array=w1375, length=w1371, index=0) -> (deleted portion=w1372:bool[])  [unwired: 1 out]
            n510 = case shown="True" w1358 {
              tunnel: w1361 -> [w1384 w1386]
              tunnel: [w1384 w1385] -> w1359
              frame False {
              }
              frame True {
                n511 = Reverse 1D Array(array=w1386) -> (reversed array=w1385:bool[])
              }
            }
            n512 = case shown="True" w1357 {
              tunnel: w1372 -> [w1381 w1383]
              tunnel: [w1381 w1382] -> w1368
              frame False {
              }
              frame True {
                n513 = Reverse 1D Array(array=w1383) -> (reversed array=w1382:bool[])
              }
            }
            n514 = Insert Into Array(array=w1368, index=w1371, new element=w1359) -> (w1379:bool[])
            n515 = Boolean Array To Number(Boolean array=w1379) -> (number=w1374:u32)
            n516 = Initialize Array(u8 255 ("element"), 4 ("dimension size")) -> (w1370:u8[])
            n517 = call "Split and Invert u16 to two u8.vi"("Invert LSB [F]"=FALSE, "Invert MSB [F]"=FALSE ("Invert LSB [F]"), "Input (u16)"=w1374) -> ("LSB (u8)"=w1363:u8, "MSB (u8)"=w1362:u8)  [unwired: 6 in, 1 out]
            n518 = Build Array (concatenate)(w1362, w1363, w1370) -> (w1364:u8[])
          }
          frame "Microchip LC56BT" {
            # "LC56BT has 7-bit address field.\n93LC56BT opcode and address fits nicely in their separate\n8-bit fields. The READ data field is a dummy (1 or 0 bits) to\nindicate to self-timed READ how many addresses to automatically\nread post the first address."
            n519 = Number To Boolean Array(number=w1400) -> (Boolean array=w1401:bool[])
            n520 = Number To Boolean Array(number=w1395) -> (Boolean array=w1398:bool[])
            n521 = Delete From Array(array=w1401, length=5 ("index"), index=0) -> (deleted portion=w1394:bool[])  [unwired: 1 out]
            n522 = Delete From Array(array=w1398, length=7 ("index"), index=0) -> (deleted portion=w1392:bool[])  [unwired: 1 out]
            n523 = Boolean Array To Number(Boolean array=w1394) -> (number=w1393:u32)
            n524 = Boolean Array To Number(Boolean array=w1392) -> (number=w1391:u32)
            n525 = To Unsigned Byte Integer(number=w1393) -> (unsigned 8bit integer=w1387:u8)
            n526 = To Unsigned Byte Integer(number=w1391) -> (unsigned 8bit integer=w1390:u8)
            n527 = Initialize Array(u8 255 ("element"), 2 ("t")) -> (w1396:u8[])
            n528 = Build Array (concatenate)(w1387, w1390, w1396) -> (w1404:u8[])
          }
          frame "Microchip 93LC86C [8452]" {
            w1408 = FALSE ("Invert LSB [F]")
            w1415 = 10 ("index")
            # "MSb transmitted first\nby NI-8452"
            # "93C86 has 10-bit address field\n2 MSB bits must be merged\ninto the LSB of the opcode field"
            n529 = Number To Boolean Array(number=w1422) -> (Boolean array=w1423:bool[])
            n530 = Number To Boolean Array(number=w1411) -> (Boolean array=w1420:bool[])
            n531 = Delete From Array(array=w1423, length=6 ("index"), index=0) -> (deleted portion=w1416:bool[])  [unwired: 1 out]
            n532 = Delete From Array(array=w1420, length=w1415, index=0) -> (deleted portion=w1417:bool[])  [unwired: 1 out]
            n533 = case shown="True" w1406 {
              tunnel: w1416 -> [w1431 w1433]
              tunnel: [w1431 w1432] -> w1407
              frame False {
              }
              frame True {
                n534 = Reverse 1D Array(array=w1433) -> (reversed array=w1432:bool[])
              }
            }
            n535 = case shown="True" w1405 {
              tunnel: w1417 -> [w1428 w1430]
              tunnel: [w1428 w1429] -> w1409
              frame False {
              }
              frame True {
                n536 = Reverse 1D Array(array=w1430) -> (reversed array=w1429:bool[])
              }
            }
            n537 = Insert Into Array(array=w1409, index=w1415, new element=w1407) -> (w1425:bool[])
            n538 = Boolean Array To Number(Boolean array=w1425) -> (number=w1419:u32)
            n539 = Initialize Array(u8 255 ("element"), 4 ("dimension size")) -> (w1414:u8[])
            n540 = call "Split and Invert u16 to two u8.vi"("Invert LSB [F]"=w1408, "Invert MSB [F]"=w1408, "Input (u16)"=w1419) -> ("LSB (u8)"=w1413:u8, "MSB (u8)"=w1412:u8)  [unwired: 6 in, 1 out]
            n541 = Build Array (concatenate)(w1412, w1413, w1414) -> (w1427:u8[])
          }
          frame "Microchip 93LC86C [8451]" {
            w1434 = FALSE ("Invert LSB [F]")
            w1441 = 10 ("index")
            # "MSb transmitted first\nby NI-8452"
            # "93C86 has 10-bit address field\n2 MSB bits must be merged\ninto the LSB of the opcode field"
            n542 = Number To Boolean Array(number=w1437) -> (Boolean array=w1446:bool[])
            n543 = Number To Boolean Array(number=w1448) -> (Boolean array=w1449:bool[])
            n544 = Delete From Array(array=w1449, length=5 ("index"), index=0) -> (deleted portion=w1442:bool[])  [unwired: 1 out]
            n545 = Delete From Array(array=w1446, length=w1441, index=0) -> (deleted portion=w1443:bool[])  [unwired: 1 out]
            n546 = Reverse 1D Array(array=w1443) -> (reversed array=w1435:bool[])
            n547 = Insert Into Array(array=w1435, index=w1441, new element=w1442) -> (w1451:bool[])
            n548 = Boolean Array To Number(Boolean array=w1451) -> (number=w1445:u32)
            n549 = Initialize Array(u8 255 ("element"), 4 ("dimension size")) -> (w1440:u8[])
            n550 = call "Split and Invert u16 to two u8.vi"("Invert LSB [F]"=w1434, "Invert MSB [F]"=w1434, "Input (u16)"=w1445) -> ("LSB (u8)"=w1439:u8, "MSB (u8)"=w1438:u8)  [unwired: 6 in, 1 out]
            n551 = Build Array (concatenate)(w1438, w1439, w1440) -> (w1453:u8[])
          }
        }
        n552 = call "NI-845x SPI Script CS High.vi"("error in (no error)"=w1336, "chip select (0)"=w1331, "spi script reference in"=w1335) -> ("error out"=w1334:errorcluster, "spi script reference out"=w1344:T1)  [unwired: 7 in]
        n553 = call "NI-845x SPI Script Write Read.vi"("error in (no error)"=w1334, "write data"=w1325, "spi script reference in"=w1344) -> ("error out"=w1346:errorcluster, "script read index"=w1340:u32, "spi script reference out"=w1345:T1)  [unwired: 1 in, 5 out]
        n554 = local write "Data Bytes Written"(w1325) -> ()
        n555 = call "NI-845x SPI Script CS Low.vi"("error in (no error)"=w1346, "chip select (0)"=w1331, "spi script reference in"=w1345) -> ("error out"=w1338:errorcluster, "spi script reference out"=w1337:T1)  [unwired: 7 in]
        n556 = call-poly "NI-845x SPI Script Delay.vi"("error in (no error)"=w1338, "delay in microseconds (0)"=u16 1, "spi script reference in"=w1337) -> ("error out"=w1333:errorcluster, "spi script reference out"=w1332:T1)  [unwired: 7 in]
        n557 = Bundle By Name(cluster=w1343, "script read index"=w1340, "Read ALL"=FALSE) -> (w1341:T10)
        n558 = call "NI-845x SPI Script CS High.vi"("error in (no error)"=w1333, "chip select (0)"=w1331, "spi script reference in"=w1332) -> ("error out"=w1328:errorcluster, "spi script reference out"=w1327:T1)  [unwired: 7 in]
        n559 = call-poly "NI-845x SPI Script Delay.vi"("error in (no error)"=w1328, "delay in microseconds (0)"=u16 1, "spi script reference in"=w1327) -> ("error out"=w1321:errorcluster, "spi script reference out"=w1320:T1)  [unwired: 7 in]
        n560 = call "NI-845x SPI Script CS Low.vi"("error in (no error)"=w1321, "spi script reference in"=w1320) -> ("error out"=w1319:errorcluster)  [unwired: 8 in, 1 out]
        n561 = call <vilib>:"Add State(s) to Queue__jki_lib_state_machine.vi"("State(s) in Front (\"\")"="UI: Display Status >>  [Alert!][READ Data Completed][100]" ("State(s) in Front (\"\")"), "State(s) in (\"\")"=w1348) -> ("States Out"=w1347:string)  [unwired: 13 in]
      }
      frame "NI845x: WRITE ALL" {
        # "93LC56BT opcode and address fits nicely in their separate\n8-bit fields. The WRITE ALL address starts at 0x0000.\nData fiels are two 8-bit of endianness you want."
        # "Delay for Tcsl"
        # "1. Send SB & WRAL opcode.\n2. A dummy address byte.\n3. Desired data pattern to write."
        n562 = Unbundle By Name(w1485) -> ("WRAL"=w1483:u8, "EEPROM Device Type"=w1470:T6, "Bit Pattern (WRITE ALL)"=w1468:T4, "Endianness (WRITE)"=w1462:bool, "Invert Data Bits [MSB]"=w1461:bool, "Invert Data Bits [LSB]"=w1460:bool, "SPI Script Reference"=w1473:T1, "CS/SS Line (0-6)"=w1454:u32, "Page Write Delay (ms)"=w1463:u8)
        n563 = call "Bit Test Pattern.vi"("Bit Pattern(u64)"=w1468) -> ("msb-lo(u16)"=w1467:u16)  [unwired: 5 in, 5 out]
        n564 = case shown="\"Microchip 93LC86C [8452]\"" w1470 {
          tunnel: [w1498 w1514 w1534 w1554 w1576] -> w1469
          tunnel: w1483 -> [w1497 w1513 w1533 w1553 w1575]
          tunnel: w1467 -> [w1494 w1508 w1528 w1550 w1570]
          tunnel: w1462 -> [w1490 w1509 w1527 w1549 w1571]
          tunnel: w1461 -> [_ w1510 w1526 w1548 w1572]
          tunnel: w1460 -> [_ w1511 w1525 w1547 w1573]
          frame "Generic EEPROM", Default {
            n565 = To Unsigned Word Integer(number=w1494) -> (unsigned 16bit integer=w1491:u16)
            n566 = case shown="True" w1490 {
              tunnel: w1491 -> [w1499 w1502]
              tunnel: [w1501 w1503] -> w1492
              tunnel: [w1500 w1504] -> w1493
              frame True {
                # "Big Endian"
                n567 = call "Split and Invert u16 to two u8.vi"("Input (u16)"=w1499) -> ("LSB (u8)"=w1501:u8, "MSB (u8)"=w1500:u8)  [unwired: 8 in, 1 out]
              }
              frame False {
                # "Little Endian"
                n568 = call "Split and Invert u16 to two u8.vi"("Input (u16)"=w1502) -> ("LSB (u8)"=w1504:u8, "MSB (u8)"=w1503:u8)  [unwired: 8 in, 1 out]
              }
            }
            n569 = To Unsigned Byte Integer(number=w1497) -> (unsigned 8bit integer=w1496:u8)
            n570 = Build Array(w1496, u8 0 ("element"), w1493, w1492) -> (w1498:u8[])
          }
          frame "ST-M93C86" {
            # "93C/LC86 opcode + 2 bits of address MSB 8-bit burst. \nThe WRITE ALL address starts at 0x0000.\nData fiels are two 8-bit of endianness you want."
            n571 = case shown="True" w1509 {
              tunnel: [w1518 w1523] -> w1505
              tunnel: [w1517 w1524] -> w1506
              tunnel: w1508 -> [w1516 w1522]
              tunnel: w1511 -> [_ w1521]
              tunnel: w1510 -> [_ w1520]
              tunnel: [w1515 w1519] -> _
              frame True {
                # "Big Endian\nMSB first"
                n572 = call "Split and Invert u16 to two u8.vi"("Input (u16)"=w1516) -> ("Output(u16)"=w1515:u32, "LSB (u8)"=w1518:u8, "MSB (u8)"=w1517:u8)  [unwired: 8 in]
              }
              frame False {
                # "Little Endian\nLSB first"
                n573 = call "Split and Invert u16 to two u8.vi"("Invert LSB [F]"=w1521, "Invert MSB [F]"=w1520, "Input (u16)"=w1522) -> ("Output(u16)"=w1519:u32, "LSB (u8)"=w1524:u8, "MSB (u8)"=w1523:u8)  [unwired: 6 in]
              }
            }
            n574 = To Unsigned Byte Integer(number=w1513) -> (unsigned 8bit integer=w1512:u8)
            n575 = Build Array(w1512, u8 0 ("element"), w1506, w1505) -> (w1514:u8[])
          }
          frame "Microchip LC56BT" {
            # "93LC56BT opcode and address fits nicely in their separate\n8-bit fields. The WRITE ALL address starts at 0x0000.\nData fiels are two 8-bit of endianness you want."
            n576 = case shown="True" w1527 {
              tunnel: w1528 -> [w1537 w1542]
              tunnel: [w1539 w1543] -> w1529
              tunnel: [w1538 w1544] -> w1530
              tunnel: w1526 -> [w1536 w1541]
              tunnel: w1525 -> [w1535 w1540]
              frame True {
                # "Big Endian"
                n577 = call "Split and Invert u16 to two u8.vi"("Invert LSB [F]"=w1535, "Invert MSB [F]"=w1536, "Input (u16)"=w1537) -> ("LSB (u8)"=w1539:u8, "MSB (u8)"=w1538:u8)  [unwired: 6 in, 1 out]
              }
              frame False {
                # "Little Endian"
                n578 = call "Split and Invert u16 to two u8.vi"("Invert LSB [F]"=w1540, "Invert MSB [F]"=w1541, "Input (u16)"=w1542) -> ("LSB (u8)"=w1544:u8, "MSB (u8)"=w1543:u8)  [unwired: 6 in, 1 out]
              }
            }
            n579 = To Unsigned Byte Integer(number=w1533) -> (unsigned 8bit integer=w1532:u8)
            n580 = Build Array(w1532, u8 0 ("element"), w1530, w1529) -> (w1534:u8[])
          }
          frame "Microchip 93LC86C [8451]" {
            # "93C/LC86 opcode is 5 bits and address is 10-bit fields. \nThe WRITE ALL address starts at 0x0000.\nData fiels are two 8-bit of endianness you want."
            n581 = case shown="True" w1549 {
              tunnel: w1550 -> [w1558 w1564]
              tunnel: [w1560 w1565] -> w1545
              tunnel: [w1559 w1566] -> w1546
              tunnel: w1548 -> [w1557 w1563]
              tunnel: w1547 -> [w1556 w1562]
              tunnel: [w1555 w1561] -> _
              frame True {
                # "Big Endian"
                n582 = call "Split and Invert u16 to two u8.vi"("Invert LSB [F]"=w1556, "Invert MSB [F]"=w1557, "Input (u16)"=w1558) -> ("Output(u16)"=w1555:u32, "LSB (u8)"=w1560:u8, "MSB (u8)"=w1559:u8)  [unwired: 6 in]
              }
              frame False {
                # "Little Endian"
                n583 = call "Split and Invert u16 to two u8.vi"("Invert LSB [F]"=w1562, "Invert MSB [F]"=w1563, "Input (u16)"=w1564) -> ("Output(u16)"=w1561:u32, "LSB (u8)"=w1566:u8, "MSB (u8)"=w1565:u8)  [unwired: 6 in]
              }
            }
            n584 = To Unsigned Byte Integer(number=w1553) -> (unsigned 8bit integer=w1552:u8)
            n585 = Build Array(w1552, u8 0 ("element"), w1546, w1545) -> (w1554:u8[])
          }
          frame "Microchip 93LC86C [8452]" {
            # "93C/LC86 opcode is 5 bits and address is 10-bits.\nThe WRITE ALL address starts at 0x0000.\nData fiels are two 8-bit of endianness you want."
            n586 = case shown="True" w1571 {
              tunnel: [w1579 w1583] -> w1567
              tunnel: [w1578 w1584] -> w1568
              tunnel: w1570 -> [w1577 w1582]
              tunnel: w1573 -> [_ w1581]
              tunnel: w1572 -> [_ w1580]
              frame True {
                # "Big Endian\nMSB first"
                n587 = call "Split and Invert u16 to two u8.vi"("Input (u16)"=w1577) -> ("LSB (u8)"=w1579:u8, "MSB (u8)"=w1578:u8)  [unwired: 8 in, 1 out]
              }
              frame False {
                # "Little Endian\nLSB first"
                n588 = call "Split and Invert u16 to two u8.vi"("Invert LSB [F]"=w1581, "Invert MSB [F]"=w1580, "Input (u16)"=w1582) -> ("LSB (u8)"=w1584:u8, "MSB (u8)"=w1583:u8)  [unwired: 6 in, 1 out]
              }
            }
            n589 = To Unsigned Byte Integer(number=w1575) -> (unsigned 8bit integer=w1574:u8)
            n590 = Build Array(w1574, u8 0 ("element"), w1568, w1567) -> (w1576:u8[])
          }
        }
        n591 = call "NI-845x SPI Script CS High.vi"("error in (no error)"=w1474, "chip select (0)"=w1454, "spi script reference in"=w1473) -> ("error out"=w1482:errorcluster, "spi script reference out"=w1484:T1)  [unwired: 7 in]
        n592 = call "NI-845x SPI Script Write Read.vi"("error in (no error)"=w1482, "write data"=w1469, "spi script reference in"=w1484) -> ("error out"=w1486:errorcluster, "script read index"=w1477:u32, "spi script reference out"=w1487:T1)  [unwired: 1 in, 5 out]
        n593 = local write "Data Bytes Written"(w1469) -> ()
        n594 = call "NI-845x SPI Script CS Low.vi"("error in (no error)"=w1486, "chip select (0)"=w1454, "spi script reference in"=w1487) -> ("error out"=w1472:errorcluster, "spi script reference out"=w1471:T1)  [unwired: 7 in]
        n595 = Bundle By Name(cluster=w1485, "script read index"=w1477) -> (w1478:T10)
        n596 = call-poly "NI-845x SPI Script Delay.vi"("error in (no error)"=w1472, "delay in microseconds (0)"=u16 1, "spi script reference in"=w1471) -> ("error out"=w1481:errorcluster, "spi script reference out"=w1480:T1)  [unwired: 7 in]
        n597 = call "NI-845x SPI Script CS High.vi"("error in (no error)"=w1481, "chip select (0)"=w1454, "spi script reference in"=w1480) -> ("error out"=w1475:errorcluster, "spi script reference out"=w1476:T1)  [unwired: 7 in]
        n598 = call-poly "NI-845x SPI Script Delay.vi"("error in (no error)"=w1475, "delay in milliseconds (0)"=w1463, "spi script reference in"=w1476) -> ("error out"=w1466:errorcluster, "spi script reference out"=w1465:T1)  [unwired: 7 in]
        n599 = call "NI-845x SPI Script CS Low.vi"("error in (no error)"=w1466, "spi script reference in"=w1465) -> ("error out"=w1459:errorcluster, "spi script reference out"=w1458:T1)  [unwired: 8 in]
        n600 = call "NI-845x SPI Script CS High.vi"("error in (no error)"=w1459, "chip select (0)"=w1454, "spi script reference in"=w1458) -> ("error out"=w1457:errorcluster, "spi script reference out"=w1456:T1)  [unwired: 7 in]
        n601 = call "NI-845x SPI Script CS Low.vi"("error in (no error)"=w1457, "chip select (0)"=w1454, "spi script reference in"=w1456) -> ("error out"=w1455:errorcluster)  [unwired: 7 in, 1 out]
        n602 = call <vilib>:"Add State(s) to Queue__jki_lib_state_machine.vi"("State(s) in Front (\"\")"="UI: Display Status >>  [Alert!][WRITE ALL Completed][100]" ("State(s) in Front (\"\")"), "State(s) in (\"\")"=w1489) -> ("States Out"=w1488:string)  [unwired: 13 in]
      }
      frame "NI845x: ERASE ALL" {
        # "It takes a few ms to complete\nthe ERASE ALL cycle"
        # "Then assert the CS line\nto start the ERASE ALL\ncycle. The ERASE ALL\ncycle is self-timed. \nNo need to CLK"
        # "Delay for Tcsl"
        # "1. Send SB & ERAL Opcode\n2. A dummy address byte\n3. A dummy data byte"
        n603 = Unbundle By Name(w1607) -> ("ERAL"=w1605:u8, "EEPROM Device Type"=w1592:T6, "SPI Script Reference"=w1586:T1, "CS/SS Line (0-6)"=w1585:u32, "Page Write Delay (ms)"=w1593:u8)
        n604 = case shown="\"ST-M93C86\"" w1592 {
          tunnel: [w1615 w1619 w1623 w1627 w1631] -> w1591
          tunnel: w1605 -> [w1614 w1618 w1622 w1626 w1628]
          frame "Generic EEPROM", Default {
            # "5-bits for each opcode  10-bits address  (two u8 array elements) only"
            n605 = To Unsigned Byte Integer(number=w1614) -> (unsigned 8bit integer=w1613:u8)
            n606 = Build Array(w1613, u8 0 ("element")) -> (w1615:u8[])
          }
          frame "ST-M93C86" {
            # "5-bits for each opcode  10-bits address  (two u8 array elements) only"
            n607 = To Unsigned Byte Integer(number=w1618) -> (unsigned 8bit integer=w1617:u8)
            n608 = Build Array(w1617, u8 0 ("element")) -> (w1619:u8[])
          }
          frame "Microchip LC56BT" {
            # "5-bits for each opcode  10-bits address  (two u8 array elements) only"
            n609 = To Unsigned Byte Integer(number=w1622) -> (unsigned 8bit integer=w1621:u8)
            n610 = Build Array(w1621, u8 0 ("element")) -> (w1623:u8[])
          }
          frame "Microchip 93LC86C [8451]" {
            # "5-bits for each opcode  10-bits address  (two u8 array elements) only"
            n611 = To Unsigned Byte Integer(number=w1626) -> (unsigned 8bit integer=w1625:u8)
            n612 = Build Array(w1625, u8 0 ("element")) -> (w1627:u8[])
          }
          frame "Microchip 93LC86C [8452]" {
            # "5-bits for each opcode  10-bits address  (two u8 array elements) only"
            n613 = To Unsigned Byte Integer(number=w1628) -> (unsigned 8bit integer=w1630:u8)
            n614 = Build Array(w1630, u8 0 ("element")) -> (w1631:u8[])
          }
        }
        n615 = call "NI-845x SPI Script CS High.vi"("error in (no error)"=w1587, "chip select (0)"=w1585, "spi script reference in"=w1586) -> ("error out"=w1601:errorcluster, "spi script reference out"=w1606:T1)  [unwired: 7 in]
        n616 = call "NI-845x SPI Script Write Read.vi"("error in (no error)"=w1601, "write data"=w1591, "spi script reference in"=w1606) -> ("error out"=w1608:errorcluster, "script read index"=w1596:u32, "spi script reference out"=w1609:T1)  [unwired: 1 in, 5 out]
        n617 = local write "Data Bytes Written"(w1591) -> ()
        n618 = call "NI-845x SPI Script CS Low.vi"("error in (no error)"=w1608, "chip select (0)"=w1585, "spi script reference in"=w1609) -> ("error out"=w1604:errorcluster, "spi script reference out"=w1603:T1)  [unwired: 7 in]
        n619 = Bundle By Name(cluster=w1607, "script read index"=w1596) -> (w1597:T10)
        n620 = call-poly "NI-845x SPI Script Delay.vi"("error in (no error)"=w1604, "delay in microseconds (0)"=u16 1, "spi script reference in"=w1603) -> ("error out"=w1600:errorcluster, "spi script reference out"=w1599:T1)  [unwired: 7 in]
        n621 = call "NI-845x SPI Script CS High.vi"("error in (no error)"=w1600, "chip select (0)"=w1585, "spi script reference in"=w1599) -> ("error out"=w1595:errorcluster, "spi script reference out"=w1594:T1)  [unwired: 7 in]
        n622 = call-poly "NI-845x SPI Script Delay.vi"("error in (no error)"=w1595, "delay in milliseconds (0)"=w1593, "spi script reference in"=w1594) -> ("error out"=w1590:errorcluster, "spi script reference out"=w1589:T1)  [unwired: 7 in]
        n623 = call "NI-845x SPI Script CS Low.vi"("error in (no error)"=w1590, "chip select (0)"=w1585, "spi script reference in"=w1589) -> ("error out"=w1588:errorcluster)  [unwired: 7 in, 1 out]
        n624 = call <vilib>:"Add State(s) to Queue__jki_lib_state_machine.vi"("State(s) in Front (\"\")"="UI: Display Status >>  [Alert!][ERASE ALL Completed][100]" ("State(s) in Front (\"\")"), "State(s) in (\"\")"=w1611) -> ("States Out"=w1610:string)  [unwired: 13 in]
      }
      frame "NI845x: RUN Script - Read Data - Close Device" {
        # "Close SPI bus, Run Script, Read the Data Array from Device, Close the reference to Device"
        n625 = Unbundle By Name(w1646) -> ("EEPROM Device Type"=w1637:T6, "script read index"=w1641:u32, "NI845x Device ID"=w1640:T5, "SPI Script Reference"=w1647:T1)
        n626 = case shown="\"Microchip 93LC86C [8452]\"" w1637 {
          tunnel: [2 ("index") 2 ("index") 2 ("index") 3 ("index") 2 ("index")] -> w1639
          frame "Generic EEPROM", Default {
          }
          frame "ST-M93C86" {
          }
          frame "Microchip LC56BT" {
          }
          frame "Microchip 93LC86C [8451]" {
          }
          frame "Microchip 93LC86C [8452]" {
            # "default = 3"
          }
        }
        n627 = call "NI-845x SPI Script Disable SPI.vi"("error in (no error)"=w1649, "spi script reference in"=w1647) -> ("error out"=w1650:errorcluster, "spi script reference out"=w1651:T1)  [unwired: 8 out]
        n628 = call "NI-845x SPI Run Script.vi"("error in (no error)"=w1650, "device reference in"=w1640, "spi script reference in"=w1651) -> ("error out"=w1644:errorcluster, "spi script reference out"=w1645:T1)  [unwired: 1 in, 6 out]
        n629 = call "NI-845x SPI Extract Script Read Data.vi"("error in (no error)"=w1644, "script read index"=w1641, "spi script reference in"=w1645) -> ("error out"=w1643:errorcluster, "read data"=w1636:u8[], "spi script reference out"=w1642:T1)  [unwired: 6 out]
        n630 = Array Subset(array=w1636, index=w1639) -> (w1634:u8[])  [unwired: 1 in]
        n631 = call-poly "NI-845x Close Reference.vi"("error in (no error)"=w1643, "spi script reference"=w1642) -> ("error out"=w1648:errorcluster)  [unwired: 9 out]
        n632 = case shown="\"Microchip 93LC86C [8452]\"" w1637 {
          tunnel: w1634 -> [w1654 w1665 w1679 w1680 w1691]
          tunnel: [w1654 w1664 w1679 w1680 w1690] -> w1635
          frame "Generic EEPROM", Default {
            # "Check your device datasheet\nfor READ format details"
          }
          frame "ST-M93C86" {
            # "// then assemble the array of booleans  in series\n// MSb is added first to array"
            # "// Then slice the assembled boolean array\nback to separate 8-bit u8 array of numbers.\n// MSb s/b the first element of 8-bit array"
            # "strip the dummy \"0\" bit\nfrom first 8-bits read (MSb)"
            # "// strip the dummy \"00\" bit from first 8-bits read and pass the remainder\nto  assemble the array of booleans  in series\n// Slice the assembled boolean array back to  separate 8-bit u8 array of numbers"
            n633 = Delete From Array(array=w1665, index=0) -> (deleted portion=w1661:u8, array with subset deleted=w1663:u8[])  [unwired: 1 in]
            n634 = Number To Boolean Array(number=w1661) -> (Boolean array=w1660:bool[])
            n635 = Array Size(array=w1665) -> (size(s)=w1657:i32)
            n636 = Delete From Array(array=w1660, length=1) -> (array with subset deleted=w1659:bool[])  [unwired: 1 in, 1 out]
            n637 = Reverse 1D Array(array=w1659) -> (reversed array=w1655:bool[])
            n638 = for {
              tunnel: w1663 -> [w1678] mode=indexing
              shift-right: [w1677] -> w1656
              shift-left: w1655 -> [w1675]
              n639 = Number To Boolean Array(number=w1678) -> (Boolean array=w1676:bool[])
              n640 = Array Size(array=w1675) -> (size(s)=w1674:i32)
              n641 = Reverse 1D Array(array=w1676) -> (reversed array=w1673:bool[])
              n642 = Insert Into Array(array=w1675, index=w1674, new element=w1673) -> (w1677:bool[])
            }
            n643 = for {
              N: w1657 -> [_]
              tunnel: [w1671] -> w1664 mode=indexing
              tunnel: w1656 -> [w1667]
              i -> [w1669]
              w1668 = 8 ("length")
              n644 = Multiply(x=w1668, y=w1669) -> (x*y=w1670:i32)
              n645 = Delete From Array(array=w1667, length=w1668, index=w1670) -> (deleted portion=w1672:bool[])  [unwired: 1 out]
              n646 = Reverse 1D Array(array=w1672) -> (reversed array=w1666:bool[])
              n647 = Boolean Array To Number(Boolean array=w1666) -> (number=w1671:u32)
            }
          }
          frame "Microchip LC56BT" {
          }
          frame "Microchip 93LC86C [8451]" {
            # "// strip the dummy \"00\" bit from first 8-bits read and pass the remainder\nto  assemble the array of booleans  in series\n// Slice the assembled boolean array back to  separate 8-bit u8 array of numbers"
          }
          frame "Microchip 93LC86C [8452]" {
            # "// Then slice the assembled boolean array\nback to separate 8-bit u8 array of numbers.\n// MSb s/b the first element of 8-bit array"
            # "// then assemble the array of booleans  in series\n// MSb is added first to array"
            # "strip the dummy \"0\" bit\nfrom first 8-bits read (MSb)"
            # "// strip the dummy \"00\" bit from first 8-bits read and pass the remainder\nto  assemble the array of booleans  in series\n// Slice the assembled boolean array back to  separate 8-bit u8 array of numbers"
            n648 = Delete From Array(array=w1691, index=0) -> (deleted portion=w1687:u8, array with subset deleted=w1689:u8[])  [unwired: 1 in]
            n649 = Number To Boolean Array(number=w1687) -> (Boolean array=w1686:bool[])
            n650 = Array Size(array=w1691) -> (size(s)=w1683:i32)
            n651 = Delete From Array(array=w1686, length=1) -> (array with subset deleted=w1685:bool[])  [unwired: 1 in, 1 out]
            n652 = Reverse 1D Array(array=w1685) -> (reversed array=w1681:bool[])
            n653 = for {
              tunnel: w1689 -> [w1704] mode=indexing
              shift-right: [w1703] -> w1682
              shift-left: w1681 -> [w1701]
              n654 = Number To Boolean Array(number=w1704) -> (Boolean array=w1702:bool[])
              n655 = Array Size(array=w1701) -> (size(s)=w1700:i32)
              n656 = Reverse 1D Array(array=w1702) -> (reversed array=w1699:bool[])
              n657 = Insert Into Array(array=w1701, index=w1700, new element=w1699) -> (w1703:bool[])
            }
            n658 = for {
              N: w1683 -> [_]
              tunnel: [w1697] -> w1690 mode=indexing
              tunnel: w1682 -> [w1693]
              i -> [w1695]
              w1694 = 8 ("length")
              n659 = Multiply(x=w1694, y=w1695) -> (x*y=w1696:i32)
              n660 = Delete From Array(array=w1693, length=w1694, index=w1696) -> (deleted portion=w1698:bool[])  [unwired: 1 out]
              n661 = Reverse 1D Array(array=w1698) -> (reversed array=w1692:bool[])
              n662 = Boolean Array To Number(Boolean array=w1692) -> (number=w1697:u32)
            }
          }
        }
        n663 = local write "Read Data"(w1634) -> ()
        n664 = Bundle By Name(cluster=w1646, "Enable Debug?"=FALSE, "Read Data"=w1635) -> (w1638:T10)
        n665 = call <vilib>:"Add State(s) to Queue__jki_lib_state_machine.vi"("State(s) in Front (\"\")"="UI: Display Status >>  [Alert!][Parse Read Data Completed][100]" ("State(s) in Front (\"\")"), "State(s) in (\"\")"=w1653) -> ("States Out"=w1652:string)  [unwired: 13 in]
      }
      frame "NI845x: Run Script - Close SPI - Close Device" {
        n666 = Unbundle By Name(w1716) -> ("NI845x Device ID"=w1713:T5, "SPI Script Reference"=w1717:T1)
        n667 = call "NI-845x SPI Script Disable SPI.vi"("error in (no error)"=w1719, "spi script reference in"=w1717) -> ("error out"=w1720:errorcluster, "spi script reference out"=w1721:T1)  [unwired: 8 out]
        n668 = call "NI-845x SPI Run Script.vi"("error in (no error)"=w1720, "device reference in"=w1713, "spi script reference in"=w1721) -> ("error out"=w1714:errorcluster, "spi script reference out"=w1715:T1)  [unwired: 1 in, 6 out]
        n669 = call-poly "NI-845x Close Reference.vi"("error in (no error)"=w1714, "spi script reference"=w1715) -> ("error out"=w1718:errorcluster)  [unwired: 9 out]
        n670 = Bundle By Name(cluster=w1716, "Enable Debug?"=FALSE) -> (w1712:T10)
        n671 = call <vilib>:"Add State(s) to Queue__jki_lib_state_machine.vi"("State(s) in Front (\"\")"="UI: Display Status >>  [Alert!][EEPROM Device Program Completed][100]" ("State(s) in Front (\"\")"), "State(s) in (\"\")"=w1723) -> ("States Out"=w1722:string)  [unwired: 13 in]
      }
      frame "NI845x: Execute Script" {
        n672 = Unbundle By Name(w1730) -> ("NI845x Device ID"=w1727:T5, "SPI Script Reference"=w1731:T1)
        n673 = call "NI-845x SPI Script Disable SPI.vi"("error in (no error)"=w1733, "spi script reference in"=w1731) -> ("error out"=w1734:errorcluster, "spi script reference out"=w1735:T1)  [unwired: 8 out]
        n674 = call "NI-845x SPI Run Script.vi"("error in (no error)"=w1734, "device reference in"=w1727, "spi script reference in"=w1735) -> ("error out"=w1728:errorcluster, "spi script reference out"=w1729:T1)  [unwired: 1 in, 6 out]
        n675 = call-poly "NI-845x Close Reference.vi"("error in (no error)"=w1728, "spi script reference"=w1729) -> ("error out"=w1732:errorcluster)  [unwired: 9 out]
        n676 = Bundle By Name(cluster=w1730, "Enable Debug?"=FALSE) -> (w1726:T10)
        n677 = call <vilib>:"Add State(s) to Queue__jki_lib_state_machine.vi"("State(s) in Front (\"\")"="UI: Display Status >>  [Alert!][EEPROM Device Program Completed][100]" ("State(s) in Front (\"\")"), "State(s) in (\"\")"=w1737) -> ("States Out"=w1736:string)  [unwired: 13 in]
      }
      frame "NI845x: Upload BInary File" {
        # "// Purge all remaining states\n// create new states to repeat until\n// all remaining WRITE data"
        # "// save remaining WRITE data"
        # "// NI-845x can only take d62 (0x3E) max # scripts. Split the array and repeat call to this page"
        n678 = Unbundle By Name(w1766) -> ("EEPROM Binary File Array"=w1738:string[][], "EEPROM Device Type"=w1757:T6, "CS/SS Line (0-6)"=w1769:u32, "Page Write Delay (ms)"=w1767:u8, "SPI Script Reference"=w1756:T1, "WRITE"=w1770:u8, "Invert Opcode"=w1762:bool, "Endianness (WRITE)"=w1765:bool, "Invert Data Bits [MSB]"=w1764:bool, "Invert Data Bits [LSB]"=w1763:bool, "EEPROM Program Data"=w1750:string[][])
        n679 = Array Size(array=w1750) -> (size(s)=w1752:i32[])
        n680 = Array Size(array=w1738) -> (size(s)=w1749:i32[])
        n681 = Index Array(array=w1752, index=0) -> (element=w1745:i32)
        n682 = Index Array(array=w1749, index=0) -> (element=w1744:i32)
        n683 = case shown="\"Generic EEPROM\", Default" w1757 {
          tunnel: [32 ("length")] -> w1743
          frame "Generic EEPROM", Default {
          }
        }
        n684 = Quotient & Remainder(x=w1745, y=w1743) -> (floor(x/y)=w1742:i32)  [unwired: 1 out]
        n685 = Quotient & Remainder(x=w1744, y=w1743) -> (floor(x/y)=w1741:i32)  [unwired: 1 out]
        n686 = Subtract(x=w1742, y=w1741) -> (x-y=w1740:i32)
        n687 = Increment(x=w1740) -> (x+1=w1739:i32)
        n688 = To Double Precision Float(number=w1742) -> (double precision float=w1746:dbl)
        n689 = property on="Program Data Array" class="Slide (strict)"(error in=w1754, "Scale.Maximum"=w1746, "Value"=w1739, "Scale.Minimum"=0.0 ("Scale.Range:Minimum")) -> (error out=w1753:errorcluster)  [unwired: 1 in, 1 out]
        n690 = Delete From Array(array=w1738, length=w1743, index (row)=0) -> (deleted portion=w1761:string[][], array with subset deleted=w1759:string[][])  [unwired: 1 in]
        n691 = for {
          tunnel: w1753 -> [w1780]
          tunnel: w1770 -> [w1799]
          tunnel: w1769 -> [w1816]
          tunnel: [w1778] -> w1768
          tunnel: w1767 -> [w1781]
          tunnel: w1761 -> [w1822] mode=indexing
          tunnel: w1765 -> [w1791]
          tunnel: w1764 -> [w1792]
          tunnel: w1763 -> [w1786]
          tunnel: w1762 -> [w1782]
          tunnel: w1756 -> [w1779]
          w1785 = FALSE ("Invert LSB [F]")
          w1795 = 10 ("index")
          # "1. 93C86 has 10-bit address field 2 MSB bits must be merged\ninto the LSB of the opcode field\n2. NI-845x transmits MSb (bit) first so rotate the bits??\n3. ST MC93C86 is big-endian arrangement (MSB byte stored at higher-order byte of word and stored at lowest address."
          # "Data"
          # "Address"
          n692 = Number To Boolean Array(number=w1799) -> (Boolean array=w1812:bool[])
          n693 = Index Array(array=w1822, index=0) -> (element=w1824:string)
          n694 = Index Array(array=w1822, index=1) -> (element=w1820:string)
          n695 = Delete From Array(array=w1812, length=5 ("index"), index=0) -> (deleted portion=w1784:bool[])  [unwired: 1 out]
          n696 = call "Hex_String_to_Binary_String.vi"("bitness"=enum16{"8", "16", "32", "64"}."16", "Hexadecimal String"=w1824) -> ("number"=w1813:u64)  [unwired: 1 in, 2 out]
          n697 = case shown="True" w1782 {
            tunnel: w1784 -> [w1827 w1829]
            tunnel: [w1827 w1828] -> w1783
            frame False {
            }
            frame True {
              n698 = Reverse 1D Array(array=w1829) -> (reversed array=w1828:bool[])
            }
          }
          n699 = call "Hex_String_to_Binary_String.vi"("bitness"=enum16{"8", "16", "32", "64"}."16", "Hexadecimal String"=w1820) -> ("number"=w1819:u64)  [unwired: 1 in, 2 out]
          n700 = To Unsigned Word Integer(number=w1813) -> (unsigned 16bit integer=w1800:u16)
          n701 = To Unsigned Word Integer(number=w1819) -> (unsigned 16bit integer=w1790:u16)
          n702 = Number To Boolean Array(number=w1800) -> (Boolean array=w1804:bool[])
          n703 = case shown="True" w1791 {
            tunnel: [w1834 w1838] -> w1776
            tunnel: [w1833 w1839] -> w1777
            tunnel: w1790 -> [w1832 w1837]
            tunnel: w1792 -> [w1831 w1836]
            tunnel: w1786 -> [w1830 w1835]
            frame True {
              # "Big Endian\nMSB first"
              n704 = call "Split and Invert u16 to two u8.vi"("Invert LSB [F]"=w1830, "Invert MSB [F]"=w1831, "Input (u16)"=w1832) -> ("LSB (u8)"=w1834:u8, "MSB (u8)"=w1833:u8)  [unwired: 6 in, 1 out]
            }
            frame False {
              # "Little Endian\nLSB first"
              n705 = call "Split and Invert u16 to two u8.vi"("Invert LSB [F]"=w1835, "Invert MSB [F]"=w1836, "Input (u16)"=w1837) -> ("LSB (u8)"=w1839:u8, "MSB (u8)"=w1838:u8)  [unwired: 6 in, 1 out]
            }
          }
          n706 = Delete From Array(array=w1804, length=w1795, index=0) -> (deleted portion=w1789:bool[])  [unwired: 1 out]
          n707 = Insert Into Array(array=w1789, index=w1795, new element=w1783) -> (w1806:bool[])
          n708 = Boolean Array To Number(Boolean array=w1806) -> (number=w1798:u32)
          n709 = call "Split and Invert u16 to two u8.vi"("Invert LSB [F]"=w1785, "Invert MSB [F]"=w1785, "Input (u16)"=w1798) -> ("LSB (u8)"=w1793:u8, "MSB (u8)"=w1794:u8)  [unwired: 6 in, 1 out]
          n710 = call "NI-845x SPI Script CS High.vi"("error in (no error)"=w1780, "chip select (0)"=w1816, "spi script reference in"=w1779) -> ("error out"=w1802:errorcluster, "spi script reference out"=w1801:T1)  [unwired: 7 in]
          n711 = Build Array(w1794, w1793, w1777, w1776) -> (w1797:u8[])
          n712 = call "NI-845x SPI Script Write Read.vi"("error in (no error)"=w1802, "write data"=w1797, "spi script reference in"=w1801) -> ("error out"=w1818:errorcluster, "spi script reference out"=w1817:T1)  [unwired: 1 in, 6 out]
          n713 = local write "Data Bytes Written"(w1797) -> ()
          n714 = call "NI-845x SPI Script CS Low.vi"("error in (no error)"=w1818, "chip select (0)"=w1816, "spi script reference in"=w1817) -> ("error out"=w1810:errorcluster, "spi script reference out"=w1808:T1)  [unwired: 7 in]
          n715 = call-poly "NI-845x SPI Script Delay.vi"("error in (no error)"=w1810, "delay in microseconds (0)"=u16 1, "spi script reference in"=w1808) -> ("error out"=w1809:errorcluster, "spi script reference out"=w1807:T1)  [unwired: 7 in]
          n716 = call "NI-845x SPI Script CS High.vi"("error in (no error)"=w1809, "chip select (0)"=w1816, "spi script reference in"=w1807) -> ("error out"=w1815:errorcluster, "spi script reference out"=w1814:T1)  [unwired: 7 in]
          n717 = call-poly "NI-845x SPI Script Delay.vi"("error in (no error)"=w1815, "delay in milliseconds (0)"=w1781, "spi script reference in"=w1814) -> ("error out"=w1788:errorcluster, "spi script reference out"=w1787:T1)  [unwired: 7 in]
          n718 = call "NI-845x SPI Script CS Low.vi"("error in (no error)"=w1788, "spi script reference in"=w1787) -> ("error out"=w1778:errorcluster)  [unwired: 8 in, 1 out]
        }
        n719 = Empty Array?(array=w1759) -> (empty?=w1758:bool)
        n720 = case shown="True" w1758 {
          tunnel: ["NI845x: Execute Script\nNI845x: Init SPI\nNI845x: EWEN\nNI845x: Upload BInary File" ("State(s) in Front (\"\")") "NI845x: EWDS\nNI845x: Run Script - Close SPI - Close Device\nUI: Cursor Set >> Idle\nUI: Display Status >>  [Alert!][Upload BInary File Completed][100]" ("State(s) in Front (\"\")")] -> w1755
          frame False {
          }
          frame True {
          }
        }
        n721 = Bundle By Name(cluster=w1766, "EEPROM Binary File Array"=w1759) -> (w1771:T10)
        n722 = call <vilib>:"Add State(s) to Queue__jki_lib_state_machine.vi"("State(s) in (\"\")"=w1755) -> ("States Out"=w1772:string)  [unwired: 14 in]
      }
      frame "---------- Archive -------------" {
        # "Template Separator\n(You can make a copy of, or modify, this frame)"
        n723 = call <vilib>:"Add State(s) to Queue__jki_lib_state_machine.vi"("State(s) in (\"\")"=w1843) -> ("States Out"=w1842:string)  [unwired: 14 in]
      }
      frame "NI845x: READ [Generic]" {
        # "This is reserved for a generic EEPROM with data paging capability\n** Use this as a template for other EEPROM device types **\nSEE DEVICE DATA SHEET FOR TIMING INFORMATION"
        n724 = Unbundle By Name(w1856) -> ("CS/SS Line (0-6)"=w1857:u32, "CS Idle Level"=w1851:enum16{"Low (Assert High)", "High (Assert Low)"}, "SPI Script Reference"=w1858:T1, "EEPROM Device Type"=w1848:T6, "READ"=w1852:u8, "Endianness (WRITE)"=w1853:bool, "Address"=w1846:u16, "Bytes to Read"=w1847:u32, "Target Page Size (bytes)"=w1845:u32)
        n725 = call "CreateWriteCluster.vi"("Page Size in Bytes"=w1845, "EEPROM Starting Address"=w1846, "Number of Bytes to Write"=w1847) -> ("Array of Write Cluster Information"=w1844:T12)  [unwired: 1 in]
        n726 = for {
          tunnel: w1858 -> [w1879]
          tunnel: w1857 -> [w1878]
          tunnel: w1855 -> [w1877]
          tunnel: [w1876] -> w1854
          tunnel: w1853 -> [w1875]
          tunnel: w1852 -> [w1874]
          tunnel: w1851 -> [w1873]
          tunnel: [w1872] -> w1849
          tunnel: w1848 -> [w1865]
          tunnel: w1844 -> [w1864] mode=indexing
          n727 = case shown="\"Low (Assert High)\"" w1873 {
            tunnel: [w1919 w1924] -> w1881
            tunnel: [w1918 w1923] -> w1880
            tunnel: w1879 -> [w1917 w1922]
            tunnel: w1878 -> [w1916 w1921]
            tunnel: w1877 -> [w1915 w1920]
            frame "High (Assert Low)", Default {
              n728 = call "NI-845x SPI Script CS Low.vi"("error in (no error)"=w1915, "chip select (0)"=w1916, "spi script reference in"=w1917) -> ("error out"=w1919:errorcluster, "spi script reference out"=w1918:T1)  [unwired: 7 in]
            }
            frame "Low (Assert High)" {
              n729 = call "NI-845x SPI Script CS High.vi"("error in (no error)"=w1920, "chip select (0)"=w1921, "spi script reference in"=w1922) -> ("error out"=w1924:errorcluster, "spi script reference out"=w1923:T1)  [unwired: 7 in]
            }
          }
          n730 = Unbundle By Name(w1864) -> ("EEPROM Address"=w1861:u16, "Data Index"=w1862:u32, "Length"=w1863:u32)
          n731 = Select(t=i16 0, s=w1875, f=i16 -8) -> (s? t:f=w1868:i16)
          n732 = Rotate(1:w1861, 2:w1868) -> (0:w1867:u16)
          n733 = Initialize Array(w1862, w1863) -> (w1866:u32[])
          n734 = case shown="\"Microchip LC56BT\", Default" w1865 {
            tunnel: w1867 -> [w1887 w1905]
            tunnel: [w1885 w1906] -> w1871
            tunnel: w1874 -> [w1886 w1900]
            tunnel: w1875 -> [_ w1901]
            tunnel: w1866 -> [w1884 w1890]
            tunnel: w1861 -> [_ w1891]
            frame "ST-M93C86" {
              n735 = Split Number(x=w1887) -> (hi(x)=w1889:u8, lo(x)=w1888:u8)
              n736 = Build Array (concatenate)(w1886, w1889, w1888, w1884) -> (w1885:u32[])
            }
            frame "Microchip LC56BT", Default {
              n737 = Number To Boolean Array(number=w1891) -> (Boolean array=w1893:bool[])
              n738 = Number To Boolean Array(number=w1900) -> (Boolean array=w1899:bool[])
              n739 = Split Number(x=w1905) -> (hi(x)=w1903:u8, lo(x)=w1904:u8)
              n740 = Index Array(array=w1893, index=8) -> (element=w1892:bool)
              n741 = Replace Array Subset(array=w1899, new element=w1892, index=3) -> (w1897:bool[])
              n742 = Select(t=w1904, s=w1901, f=w1903) -> (s? t:f=w1902:u8)
              n743 = Boolean Array To Number(Boolean array=w1897) -> (number=w1896:u32)
              n744 = To Unsigned Byte Integer(number=w1896) -> (unsigned 8bit integer=w1895:u8)
              n745 = Build Array (concatenate)(w1895, w1902, w1890) -> (w1906:u32[])
            }
          }
          n746 = call "NI-845x SPI Script Write Read.vi"("error in (no error)"=w1881, "write data"=w1871, "spi script reference in"=w1880) -> ("error out"=w1883:errorcluster, "script read index"=w1872:u32, "spi script reference out"=w1882:T1)  [unwired: 1 in, 5 out]
          n747 = case shown="\"Low (Assert High)\"" w1873 {
            tunnel: w1883 -> [w1910 w1914]
            tunnel: w1882 -> [w1909 w1913]
            tunnel: w1878 -> [w1908 w1912]
            tunnel: [w1907 w1911] -> w1876
            frame "High (Assert Low)", Default {
              n748 = call "NI-845x SPI Script CS High.vi"("error in (no error)"=w1910, "chip select (0)"=w1908, "spi script reference in"=w1909) -> ("error out"=w1907:errorcluster)  [unwired: 7 in, 1 out]
            }
            frame "Low (Assert High)" {
              n749 = call "NI-845x SPI Script CS Low.vi"("error in (no error)"=w1914, "chip select (0)"=w1912, "spi script reference in"=w1913) -> ("error out"=w1911:errorcluster)  [unwired: 7 in, 1 out]
            }
          }
        }
        n750 = Bundle By Name(cluster=w1856, "script read index"=w1849) -> (w1850:T10)
        n751 = call <vilib>:"Add State(s) to Queue__jki_lib_state_machine.vi"("State(s) in (\"\")"=w1860) -> ("States Out"=w1859:string)  [unwired: 14 in]
      }
      frame "NI845x: WRITE [Generic]" {
        # "This is reserved for a generic EEPROM with data paging capability\n** Use this as a template for other EEPROM device types **\nSEE DEVICE DATA SHEET FOR TIMING INFORMATION"
        n752 = Unbundle By Name(w1941) -> ("CS/SS Line (0-6)"=w1932:u32, "CS Idle Level"=w1933:enum16{"Low (Assert High)", "High (Assert Low)"}, "EEPROM Device Type"=w1931:T6, "Page Write Delay (ms)"=w1939:u8, "SPI Script Reference"=w1940:T1, "Endianness (WRITE)"=w1938:bool, "WRITE"=w1935:u8, "Address"=w1930:u16, "Bytes to Read"=w1927:u32, "Target Page Size (bytes)"=w1929:u32, "Bit Pattern (WRITE ALL)"=w1926:T4)
        n753 = call "CreateWriteCluster.vi"("Page Size in Bytes"=w1929, "EEPROM Starting Address"=w1930, "Number of Bytes to Write"=w1927) -> ("Array of Write Cluster Information"=w1928:T12)  [unwired: 1 in]
        n754 = for {
          N: w1927 -> [_]
          tunnel: w1926 -> [w1946]
          tunnel: [w1945] -> w1925 mode=indexing
          n755 = call "Bit Test Pattern.vi"("Bit Pattern(u64)"=w1946) -> ("msb-lo(u16)"=w1945:u16)  [unwired: 5 in, 5 out]
        }
        n756 = for {
          tunnel: w1942 -> [w1956]
          tunnel: w1940 -> [w1955]
          tunnel: w1939 -> [_]
          tunnel: w1931 -> [w1977]
          tunnel: w1938 -> [w1976]
          tunnel: [w1975] -> w1936
          tunnel: w1935 -> [w1974]
          tunnel: w1932 -> [w1967]
          tunnel: w1933 -> [w1966]
          tunnel: [w1968] -> w1934
          tunnel: w1933 -> [w1954]
          tunnel: w1932 -> [w1953]
          tunnel: w1928 -> [w1952] mode=indexing
          tunnel: w1925 -> [w1949]
          w1958 = 2 ("index")
          # "Tcsl"
          n757 = Unbundle By Name(w1952) -> ("EEPROM Address"=w1951:u16, "Data Index"=w1948:u32, "Length"=w1950:u32)
          n758 = Select(t=i16 0, s=w1976, f=i16 -8) -> (s? t:f=w1963:i16)
          n759 = Rotate(1:w1951, 2:w1963) -> (0:w1960:u16)
          n760 = Array Subset(array=w1949, index=w1948, length=w1950) -> (w1947:u16[])
          n761 = case shown="\"Microchip LC56BT\", Default" w1977 {
            tunnel: [w1989 w2010] -> w1959
            tunnel: w1960 -> [w1990 w2009]
            tunnel: w1974 -> [w1991 w1999]
            tunnel: w1976 -> [_ w2007]
            tunnel: w1947 -> [w1988 w1995]
            tunnel: w1951 -> [_ w1994]
            frame "ST-M93C86" {
              n762 = Split Number(x=w1990) -> (hi(x)=w1992:u8, lo(x)=w1993:u8)
              n763 = Build Array (concatenate)(w1991, w1992, w1993, w1988) -> (w1989:u16[])
            }
            frame "Microchip LC56BT", Default {
              n764 = Number To Boolean Array(number=w1994) -> (Boolean array=w1998:bool[])
              n765 = Split Number(x=w2009) -> (hi(x)=w2008:u8, lo(x)=w2006:u8)
              n766 = Number To Boolean Array(number=w1999) -> (Boolean array=w2004:bool[])
              n767 = Index Array(array=w1998, index=8) -> (element=w1996:bool)
              n768 = Replace Array Subset(array=w2004, new element=w1996, index=3) -> (w2002:bool[])
              n769 = Boolean Array To Number(Boolean array=w2002) -> (number=w2001:u32)
              n770 = Select(t=w2006, s=w2007, f=w2008) -> (s? t:f=w2005:u8)
              n771 = To Unsigned Byte Integer(number=w2001) -> (unsigned 8bit integer=w2000:u8)
              n772 = Build Array (concatenate)(w2000, w2005, w1995) -> (w2010:u16[])
            }
          }
          n773 = case shown="\"Low (Assert High)\"" w1954 {
            tunnel: [w1982 w1987] -> w1962
            tunnel: [w1981 w1986] -> w1961
            tunnel: w1956 -> [w1980 w1985]
            tunnel: w1955 -> [w1979 w1984]
            tunnel: w1953 -> [w1978 w1983]
            frame "High (Assert Low)" {
              n774 = call "NI-845x SPI Script CS Low.vi"("error in (no error)"=w1980, "chip select (0)"=w1978, "spi script reference in"=w1979) -> ("error out"=w1981:errorcluster, "spi script reference out"=w1982:T1)  [unwired: 7 in]
            }
            frame "Low (Assert High)" {
              n775 = call "NI-845x SPI Script CS High.vi"("error in (no error)"=w1985, "chip select (0)"=w1983, "spi script reference in"=w1984) -> ("error out"=w1986:errorcluster, "spi script reference out"=w1987:T1)  [unwired: 7 in]
            }
          }
          n776 = call "NI-845x SPI Script Write Read.vi"("error in (no error)"=w1961, "write data"=w1959, "spi script reference in"=w1962) -> ("error out"=w1973:errorcluster, "script read index"=w1975:u32, "spi script reference out"=w1972:T1)  [unwired: 1 in, 5 out]
          n777 = Array Subset(array=w1959, index=w1958, length=w1958) -> (w1957:u16[])
          n778 = case shown="\"Low (Assert High)\"" w1966 {
            tunnel: [w2015 w2020] -> w1971
            tunnel: [w2014 w2019] -> w1970
            tunnel: w1973 -> [w2013 w2018]
            tunnel: w1972 -> [w2012 w2017]
            tunnel: w1967 -> [w2011 w2016]
            frame "High (Assert Low)" {
              n779 = call "NI-845x SPI Script CS High.vi"("error in (no error)"=w2013, "chip select (0)"=w2011, "spi script reference in"=w2012) -> ("error out"=w2015:errorcluster, "spi script reference out"=w2014:T1)  [unwired: 7 in]
            }
            frame "Low (Assert High)" {
              n780 = call "NI-845x SPI Script CS Low.vi"("error in (no error)"=w2018, "chip select (0)"=w2016, "spi script reference in"=w2017) -> ("error out"=w2020:errorcluster, "spi script reference out"=w2019:T1)  [unwired: 7 in]
            }
          }
          n781 = local write "Data Bytes Written"(w1957) -> ()
          n782 = call-poly "NI-845x SPI Script Delay.vi"("error in (no error)"=w1971, "delay in microseconds (0)"=u16 1, "spi script reference in"=w1970) -> ("error out"=w1968:errorcluster)  [unwired: 8 out]
        }
        n783 = Bundle By Name(cluster=w1941, "script read index"=w1936) -> (w1937:T10)
        n784 = call <vilib>:"Add State(s) to Queue__jki_lib_state_machine.vi"("State(s) in (\"\")"=w1944) -> ("States Out"=w1943:string)  [unwired: 14 in]
      }
    }
  }
